vi "MC_8_27_12cbad_JW.vi"() -> ()   [LabVIEW 2011]
uses:
  <vilib>/Utility/file.llb/Read From Spreadsheet File (string).vi
  <vilib>/Utility/inputDevices.llb/keyboardAcquire.vi
  <vilib>/Utility/file.llb/Write To Spreadsheet File (DBL).vi
  <vilib>/Utility/file.llb/Write To Spreadsheet File (string).vi
  <vilib>/regexp/Match Regular Expression.xnode
panel:
  out "Vd Header Row 2":sgl
  in  "default (0 dbl)":ext format="%.2e"
  out "Vd Header Row":sgl
  out "Transport Array":string[][](array[string])
  in  "Treatment Concentration (mM):":dbl=nan
  in  "Surface Treatment:":string="NaN"
  in  "# Drops*:":dbl=inf
  in  "Solution Temp (C):":dbl=nan
  in  "Relative Humidity (%):":dbl=nan
  in  "Room Temp (F):":dbl=nan
  in  "Time (s):":dbl=nan
  in  "RPM:":dbl=nan
  in  "Wait Time (s):":dbl=nan
  in  "Sample #:":dbl=1.0
  in  "Fabricator:":string="NaN"
  in  "Ramp (s):":dbl=3.0
  out "X Axis Display Type":string
  out "Opj X Axis":string
  in  "Room Temp":dbl=294.0
  out "No Image 2":path=path "\\\\acad1\\physics/Jurchescu-group/JW-PD/Image Not Found.png"
  out "Save1 Array":string[][](array[string])
  out "Lin Vd":dbl
  out "Lin-Vg Array-Used":dbl[](array[numeric])
  out "Lin Id-Used":dbl[](array[numeric])
  out "Rec: Comments":string
  out "Folder Index":dbl caption="Length"
  out "Current \nRecord":string[](array[string])
  out "Transformer \nHeaders":string[](array[string])
  out "Current Device ID":string
  out "Column":string
  out "Row":string
  out "Rec: Concentration":dbl
  out "Rec: Solvent":string
  out "Rec: Method":string
  in  "?":T1(tab)
  in  "Transport File":path
  out "Transport Folder":path
  out "Rec: Material":string
  out "Accel (RPM/s):":dbl
  in  "Transfer File":path
  out "Transfer Folder":path
  in  "Image Folder":path
  out "Image File":path=path "D:/UserData/Desktop/Jeremy/WFU/Research/Programs/VI mods/Image Not Found.png"
  in  "Manual Comments":bool
  in  "Comments:":string
  out "Calc: On/Off":dbl caption="On/Off-Sat" format="%#.2e"
  out "Calc: Off I-Sat":dbl caption="Off I-Sat" format="%#.2e"
  in  "Manuel-Dielectric":bool
  in  "Manuel-Length":bool
  out "Calc: VT-Lin":dbl
  out "New: VT-Lin":dbl
  out "Rec: VT-Lin":dbl caption="VT-Lin" format="%#_3g"
  out "Calc: Trap Density-STS":dbl format="%#.2e"
  out "New: Trap Density-STS":dbl format="%#.2e"
  out "Rec: Trap Density-STS":dbl caption="N-Sat (STS)" format="%#.2e"
  out "Calc: Trap Density-VT":dbl format="%#.2e"
  out "New: Trap Density-VT":dbl format="%#.2e"
  out "Rec: Trap Density-VT":dbl caption="N-Sat (VT)" format="%#.2e"
  out "Calc: Mobility-Lin":dbl format="%#.2e"
  out "New: Mobility-Lin":dbl format="%#_4e"
  out "Rec: Mobility-Lin":dbl caption="Mobility-Lin" format="%#_3e"
  out "Calc: Mobility-Sat":dbl format="%#.2e"
  out "Rec: Length":dbl caption="Length" format="%#_3g"
  out "Rec: Width":dbl caption="Width" format="%#_4g"
  out "Rec: Dielectric (d)":dbl caption="Dielectric (d)" format="%#_3g"
  in  "Cancel Button":bool
  in  "Up Button":bool
  in  "Down Button":bool
  out "Data Name:":string
  in  "Save Changes?":bool
  in  "New: Dielectric":dbl
  in  "New: Length":dbl
  in  "New: Width":dbl
  out "New: Mobility-Sat":dbl format="%#.2e"
  in  "Blank Button":bool
  in  "Zoom":i16(slide)=-3 scale=-5.0..5.0
  out "Image Out 2":T2(plugin-control)
  out "Image Out":T2(plugin-control)
  in  "Magnification":u16(ring) items=["5x", "10x", "20x", "50x", "80x"]
  out "Total Width":dbl
  out "Distances":dbl[](array[numeric])
  in  "Undo Button":bool
  in  "Remove Button":bool
  out "Rec: Mobility-Sat":dbl caption="Mobility-Sat" format="%#.2e"
  in  "Export":bool
  out "Calc: VT-Sat":dbl format="%#.2g"
  out "New: VT-Sat":dbl format="%#.2g"
  in  "Manual-Width":bool caption="Manual"
  out "Calc: STS":dbl format="%#.2g"
  out "New: STS":dbl format="%#.2g"
  out "Rec: VT-Sat":dbl caption="VT-Sat" format="%#.2g"
  out "Rec: STS":dbl caption="STS-Sat" format="%#.2g"
  out "Rec: On/Off":dbl caption="On/Off-Sat" format="%#.2e"
  in  "Save Changes? 2":bool
  in  "Save Changes? 3":bool
  out "Rec: Temp":dbl caption="Sample Temp" format="%.1f"
  in  "New: Temp":dbl format="%.1f"
  out "Rec: Off I-Sat":dbl caption="Off I-Sat" format="%#.2e"
  in  "Independant Variable":string(combo)="Length (um):"
  in  "Transfer Plots":T3(tab)=enum."Saturation"
  in  "Lin-Trans Slider":dbl(slide) step=1.0 scale=-22.0..89.0 scale format="%#_1p"
  out "Sqrt-Lin":cluster{dbl[], dbl[]}[](graph)
  in  "Next Sqrt Lin":bool
  in  "Previous Sqrt Lin":bool
  in  "Sat-Trans Slider":dbl(slide) step=1.0 scale=-22.0..89.0 scale format="%#_1p"
  out "Sqrt-Sat":cluster{dbl[], dbl[]}[](graph)
  in  "Previous Sqrt Sat":bool
  in  "Next Sqrt Sat":bool
  out "Raw- Lin":cluster{dbl[], dbl[]}[](graph)
  out "Raw- Sat":cluster{dbl[], dbl[]}[](graph)
  in  "Log Plots":enum32{"Linear", "Saturation", "Transport"}(tab)=enum."Saturation"
  in  "Lin-Log Slider":dbl(slide) step=1.0 scale=-1.0..82.0 scale format="%#_1p"
  in  "Previous Log Lin":bool
  in  "Next Log Lin":bool
  out "Log-Lin":cluster{dbl[], dbl[]}[](graph)
  in  "Sat-Log Slider":dbl(slide) step=1.0 scale=-1.0..82.0 scale format="%#_1p"
  out "Log-Sat":cluster{dbl[], dbl[]}[](graph)
  in  "Previous Log Sat":bool
  in  "Next Log Sat":bool
  out "Transport":cluster{dbl[], dbl[]}[](graph)
  in  "Manual-Temp":bool caption="Manual"
  out "Date Created":string caption="Fabricated"
  out "Date Recorded":string="Date Recorded" caption="Measured"
  out "Image Name":string
  out "Index":string
  in  "Num Pts":dbl=5.0
  in  "NumPoints Log":dbl=5.0 caption="Num Pts"
  in  "Origin Project File":path=path "\\\\acad1\\physics/Jurchescu-group/JW-PD/Group Library/Origin Project Files/DeviceData_8_10_12a_JW.opj"
  in  "No Image File":path=path "\\\\acad1\\physics/Jurchescu-group/JW-PD/Mega Awesome/Image Not Found.png"
  out "String":string
  out "Index 2":dbl
  out "Sat Id-Log-Used":dbl[](array[numeric])
  out "Vg Array-Log-Used":dbl[](array[numeric])
  out "ROI Descriptor out":T4 {"Contours"."Type" items=["No Selection", "Point", "Line", "Rectangle", "Oval", "Polygon", "Freehand Region", "Annulus", "Unused2", "Unused3", "Broken Line", "Freehand Line", "Rotated Rectangle"]}
  out "ROI Descriptor":T4 {"Contours"."Type" items=["No Selection", "Point", "Line", "Rectangle", "Oval", "Polygon", "Freehand Region", "Annulus", "Unused2", "Unused3", "Broken Line", "Freehand Line", "Rotated Rectangle"]}
  out "Numeric 3":dbl
  out "Array 6":dbl[][](array[numeric])
  out "Cluster":T5
  out "Array 5":dbl[](array[numeric])
  out "Array 4":dbl[](array[numeric])
  out "Array 3":dbl[](array[numeric])
  out "Numeric 2":dbl
  out "Numeric":dbl
  out "Sat Id-Used":dbl[](array[numeric])
  out "Sat Vg Array-Used":dbl[](array[numeric])
  out "MobVi Index":dbl
  in  "Row Start":dbl=20.0
  # "Sample Properties"
  # "*     Inf = Full coverage\n   NaN = Unknown or Not Applicable"
  # "Data Locations"
  # "Transport Location"
  # "Transfer Location"
  # "Image Location"
  # "Recorded"
  # "Calculated"
  # "Re-Calculated"
  # "Manual"
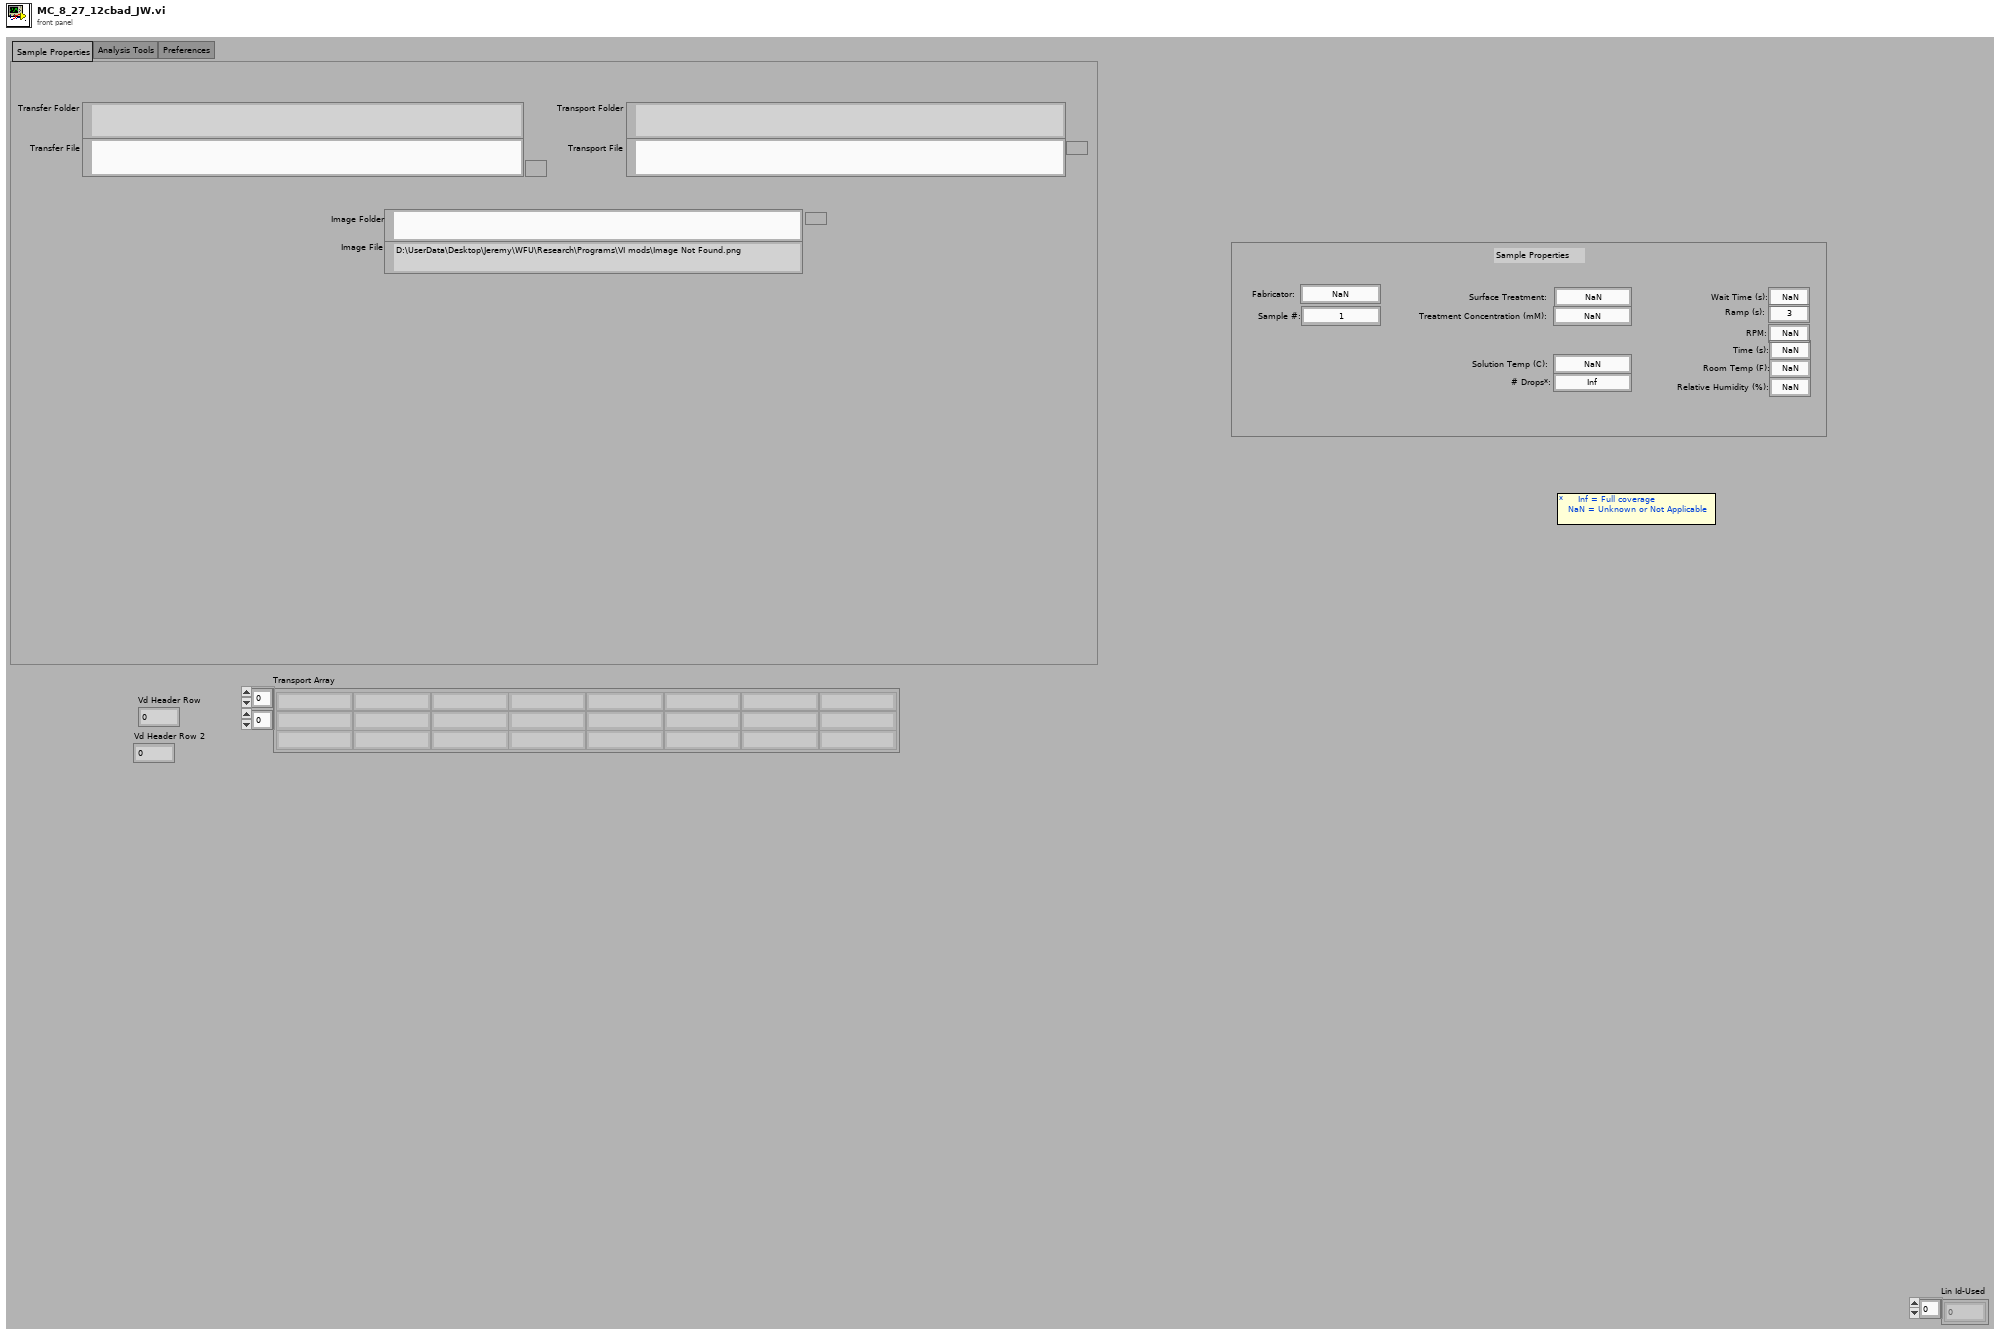
[diagram p1: front panel]
types:
  T1 = enum32{"Sample Properties", "Analysis Tools", "Preferences", "Current Database"}
  T2 = typedef "IMAQ Image.ctl" = refnum<image>
  T3 = enum32{"Linear", "Saturation", "Raw-Linear", "Raw-Saturation"}
  T4 = typedef "ROI Descriptor" = cluster{"Global Rectangle":i32[], "Contours":cluster{"ID":enum32{"External", "Internal"}, "Type":u32, "Coordinates":i32[]}[]}
  T5 = cluster{"Numeric":dbl, "Numeric 2":dbl, "Numeric 3":dbl, "Numeric 4":dbl}
  T6 = cluster{"Mobility-Sat":dbl, "Moblitity-Lin":dbl, "On/Off":dbl, "Off Current":dbl, "Vt-Sat":dbl, "STS":dbl, "Trap Density-VT":dbl, "Trap Density-STS":dbl}
  T7 = cluster{"Date Recorded":string, "Index":string, "Length":dbl, "Width":dbl, "Sample Temp":dbl}
  T8 = cluster{"Date Created":string, "Material":string, "Solvent":string, "Concentration":dbl, "Method":string, "Dielectric (nm)":dbl, "Treatment":string, "Comments":string}
  T9 = cluster{"Raw Sat":cluster{dbl[], dbl[]}[], "Sqrt Sat":cluster{dbl[], dbl[]}[], "Log Sat":cluster{dbl[], dbl[]}[], "Raw Lin":cluster{dbl[], dbl[]}[], "Sqrt Lin":cluster{dbl[], dbl[]}[], "Log Lin":cluster{dbl[], dbl[]}[]}
  T10 = cluster{"Mobility-Sat":dbl, "Vt-Sat":dbl, "Mobility-Lin":dbl, "Vt-Lin":dbl, "Off I-Sat":dbl, "On/Off I-Sat":dbl}
  T11 = cluster{"[0]":cluster{dbl[], dbl[]}, "[1]":cluster{dbl[], dbl[]}, "[2]":cluster{dbl[], dbl[]}, "[3]":cluster{dbl[], dbl[]}, "[4]":cluster{dbl[], dbl[]}, "[5]":cluster{dbl[], dbl[]}, "[6]":cluster{dbl[], dbl[]}, "[7]":cluster{dbl[], dbl[]}, "[8]":cluster{dbl[], dbl[]}}
  T12 = cluster{"Global Rectangle":i32[], "Contours":cluster{"Contour Type":u32, "ROI Type":u32, "Points":i32[]}[]}
  T13 = typedef "LVBoundsTypeDef.ctl" = cluster{"Width":u32, "Height":u32}
  T14 = enum16{"0", "1", "2", "3", "4", "5", "6", "7", "8", "9", "A", "B", "C", "D", "E", "F", "G", "H", "I", "J", "K", "L", "M", "N", "O", "P", "Q", "R", "S", "T", "U", "V", "W", "X", "Y", "Z", "F1", "F2", "F3", "F4", "F5", "F6", "F7", "F8", "F9", "F10", "F11", "F12", "F13", "F14", "F15", "ADD", "BACK", "BACKSLASH", "CAPITAL", "COMMA", "DECIMAL", "DELETE", "DIVIDE", "DOWN", "END", "EQUALS", "ESCAPE", "GRAVE (`)", "HOME", "INSERT", "LBRACKET", "LCONTROL", "LEFT", "L ALT", "LSHIFT", "LWIN", "MINUS", "MULTIPLY", "NEXT", "NUMLOCK", "NUMPAD_0", "NUMPAD_1", "NUMPAD_2", "NUMPAD_3", "NUMPAD_4", "NUMPAD_5", "NUMPAD_6", "NUMPAD_7", "NUMPAD_8", "NUMPAD_9", "PAUSE", "PERIOD", "PRIOR (PG UP)", "RBRACKET", "RCONTROL", "RETURN", "RIGHT", "R ALT", "RSHIFT", "RWIN", "SCROLL", "SEMICOLON", "SLASH", "SPACE", "SUBTRACT", "TAB", "UP", "ENTER (num pad)", "' (quote)"}[]
  T15 = enum16{"0", "1", "2", "3", "4", "5", "6", "7", "8", "9", "A", "B", "C", "D", "E", "F", "G", "H", "I", "J", "K", "L", "M", "N", "O", "P", "Q", "R", "S", "T", "U", "V", "W", "X", "Y", "Z", "F1", "F2", "F3", "F4", "F5", "F6", "F7", "F8", "F9", "F10", "F11", "F12", "F13", "F14", "F15", "ADD", "BACK", "BACKSLASH", "CAPITAL", "COMMA", "DECIMAL", "DELETE", "DIVIDE", "DOWN", "END", "EQUALS", "ESCAPE", "GRAVE (`)", "HOME", "INSERT", "LBRACKET", "LCONTROL", "LEFT", "L ALT", "LSHIFT", "LWIN", "MINUS", "MULTIPLY", "NEXT", "NUMLOCK", "NUMPAD_0", "NUMPAD_1", "NUMPAD_2", "NUMPAD_3", "NUMPAD_4", "NUMPAD_5", "NUMPAD_6", "NUMPAD_7", "NUMPAD_8", "NUMPAD_9", "PAUSE", "PERIOD", "PRIOR (PG UP)", "RBRACKET", "RCONTROL", "RETURN", "RIGHT", "R ALT", "RSHIFT", "RWIN", "SCROLL", "SEMICOLON", "SLASH", "SPACE", "SUBTRACT", "TAB", "UP", "ENTER (num pad)", "' (quote)"}
  T16 = cluster{"Contour Type":u32, "ROI Type":u32, "Points":i32[]}[]
  T17 = cluster{i32[], cluster{"Contour Type":u32, "ROI Type":u32, "Points":i32[]}[]}
  T18 = cluster{"Independant  Variable Indicator":string, "Parameter String Indicator":string}
  T19 = cluster{string, sgl, bool, bool, bool, bool, bool, bool, i32}
  T20 = cluster{i32, cluster{string, sgl, bool, bool, bool, bool, bool, bool, i32}, i32, i32}
  T21 = cluster{"Contour Type":u32, "ROI Type":u32, "Points":i32[]}
  T22 = cluster{"Points[0]":i32, "Points[1]":i32, "Points[2]":i32, "Points[3]":i32, "Points[4]":i32, "Points[5]":i32, "Points[6]":i32, "Points[7]":i32, "Points[8]":i32}
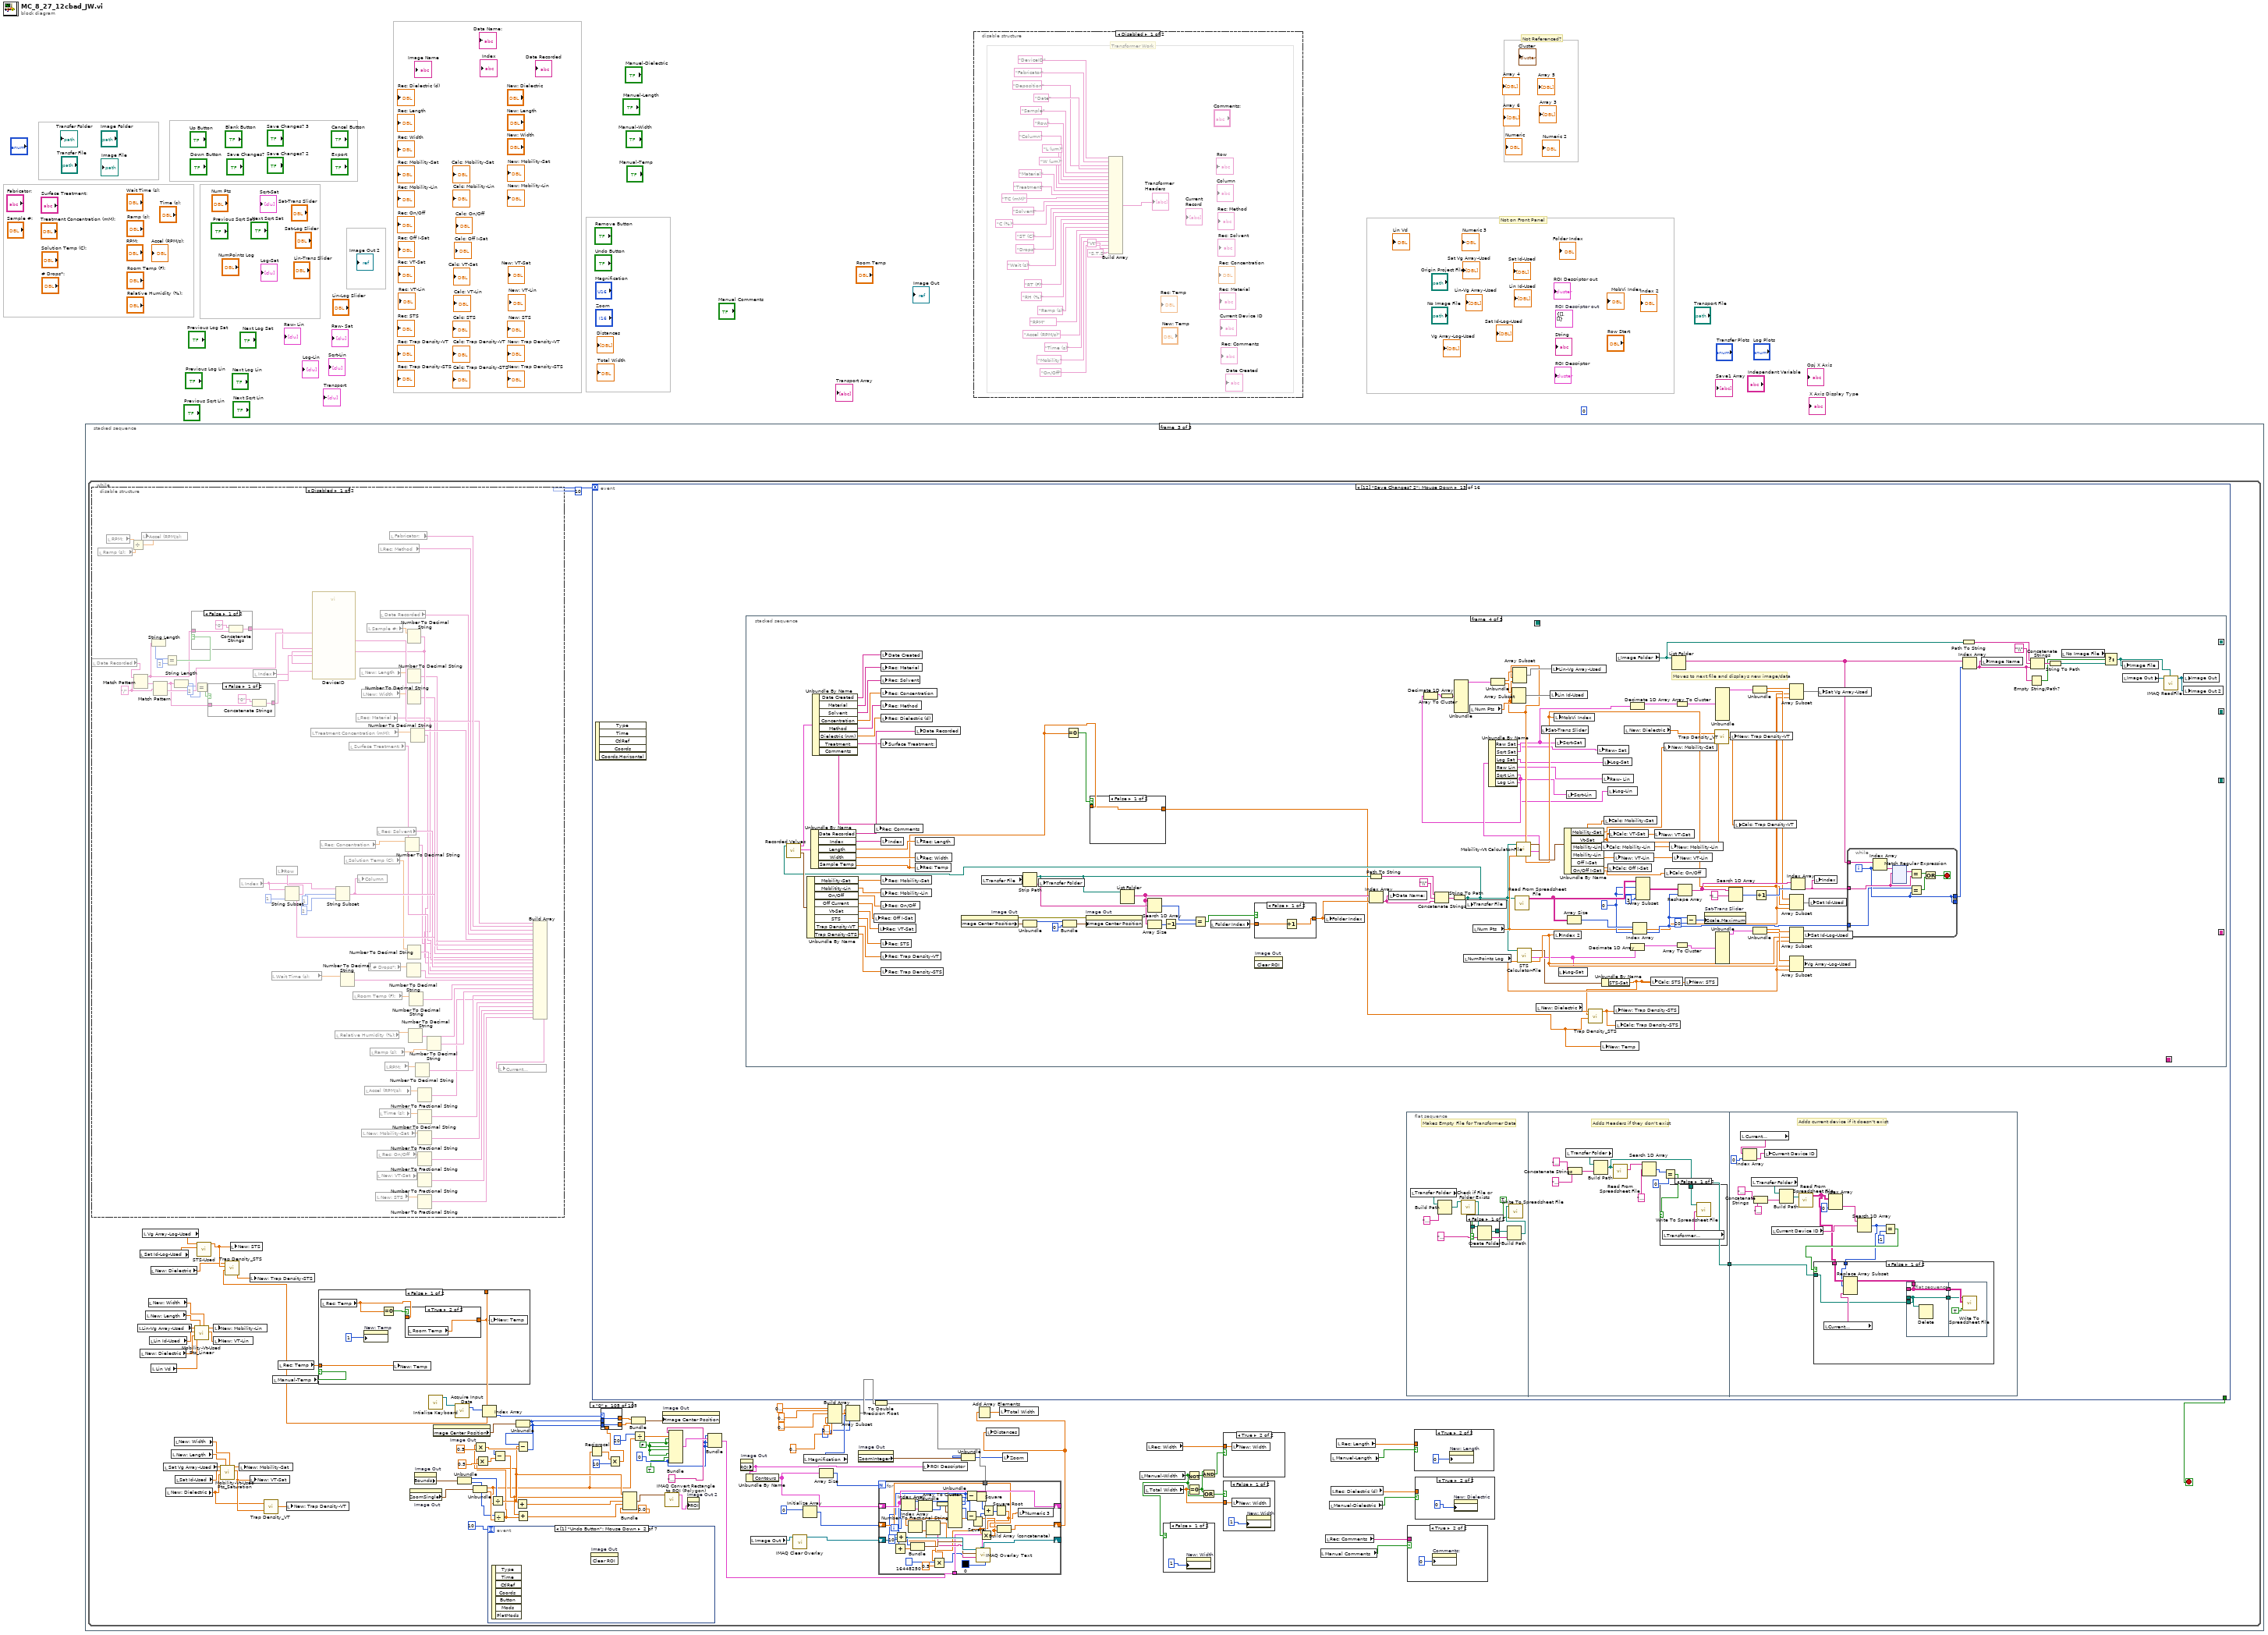
[diagram p0: block diagram]
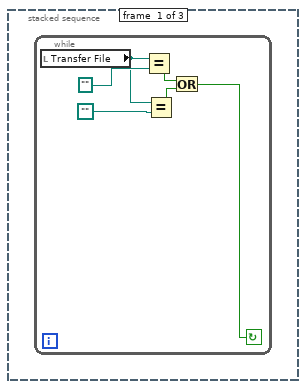
[diagram p3: hidden frame]
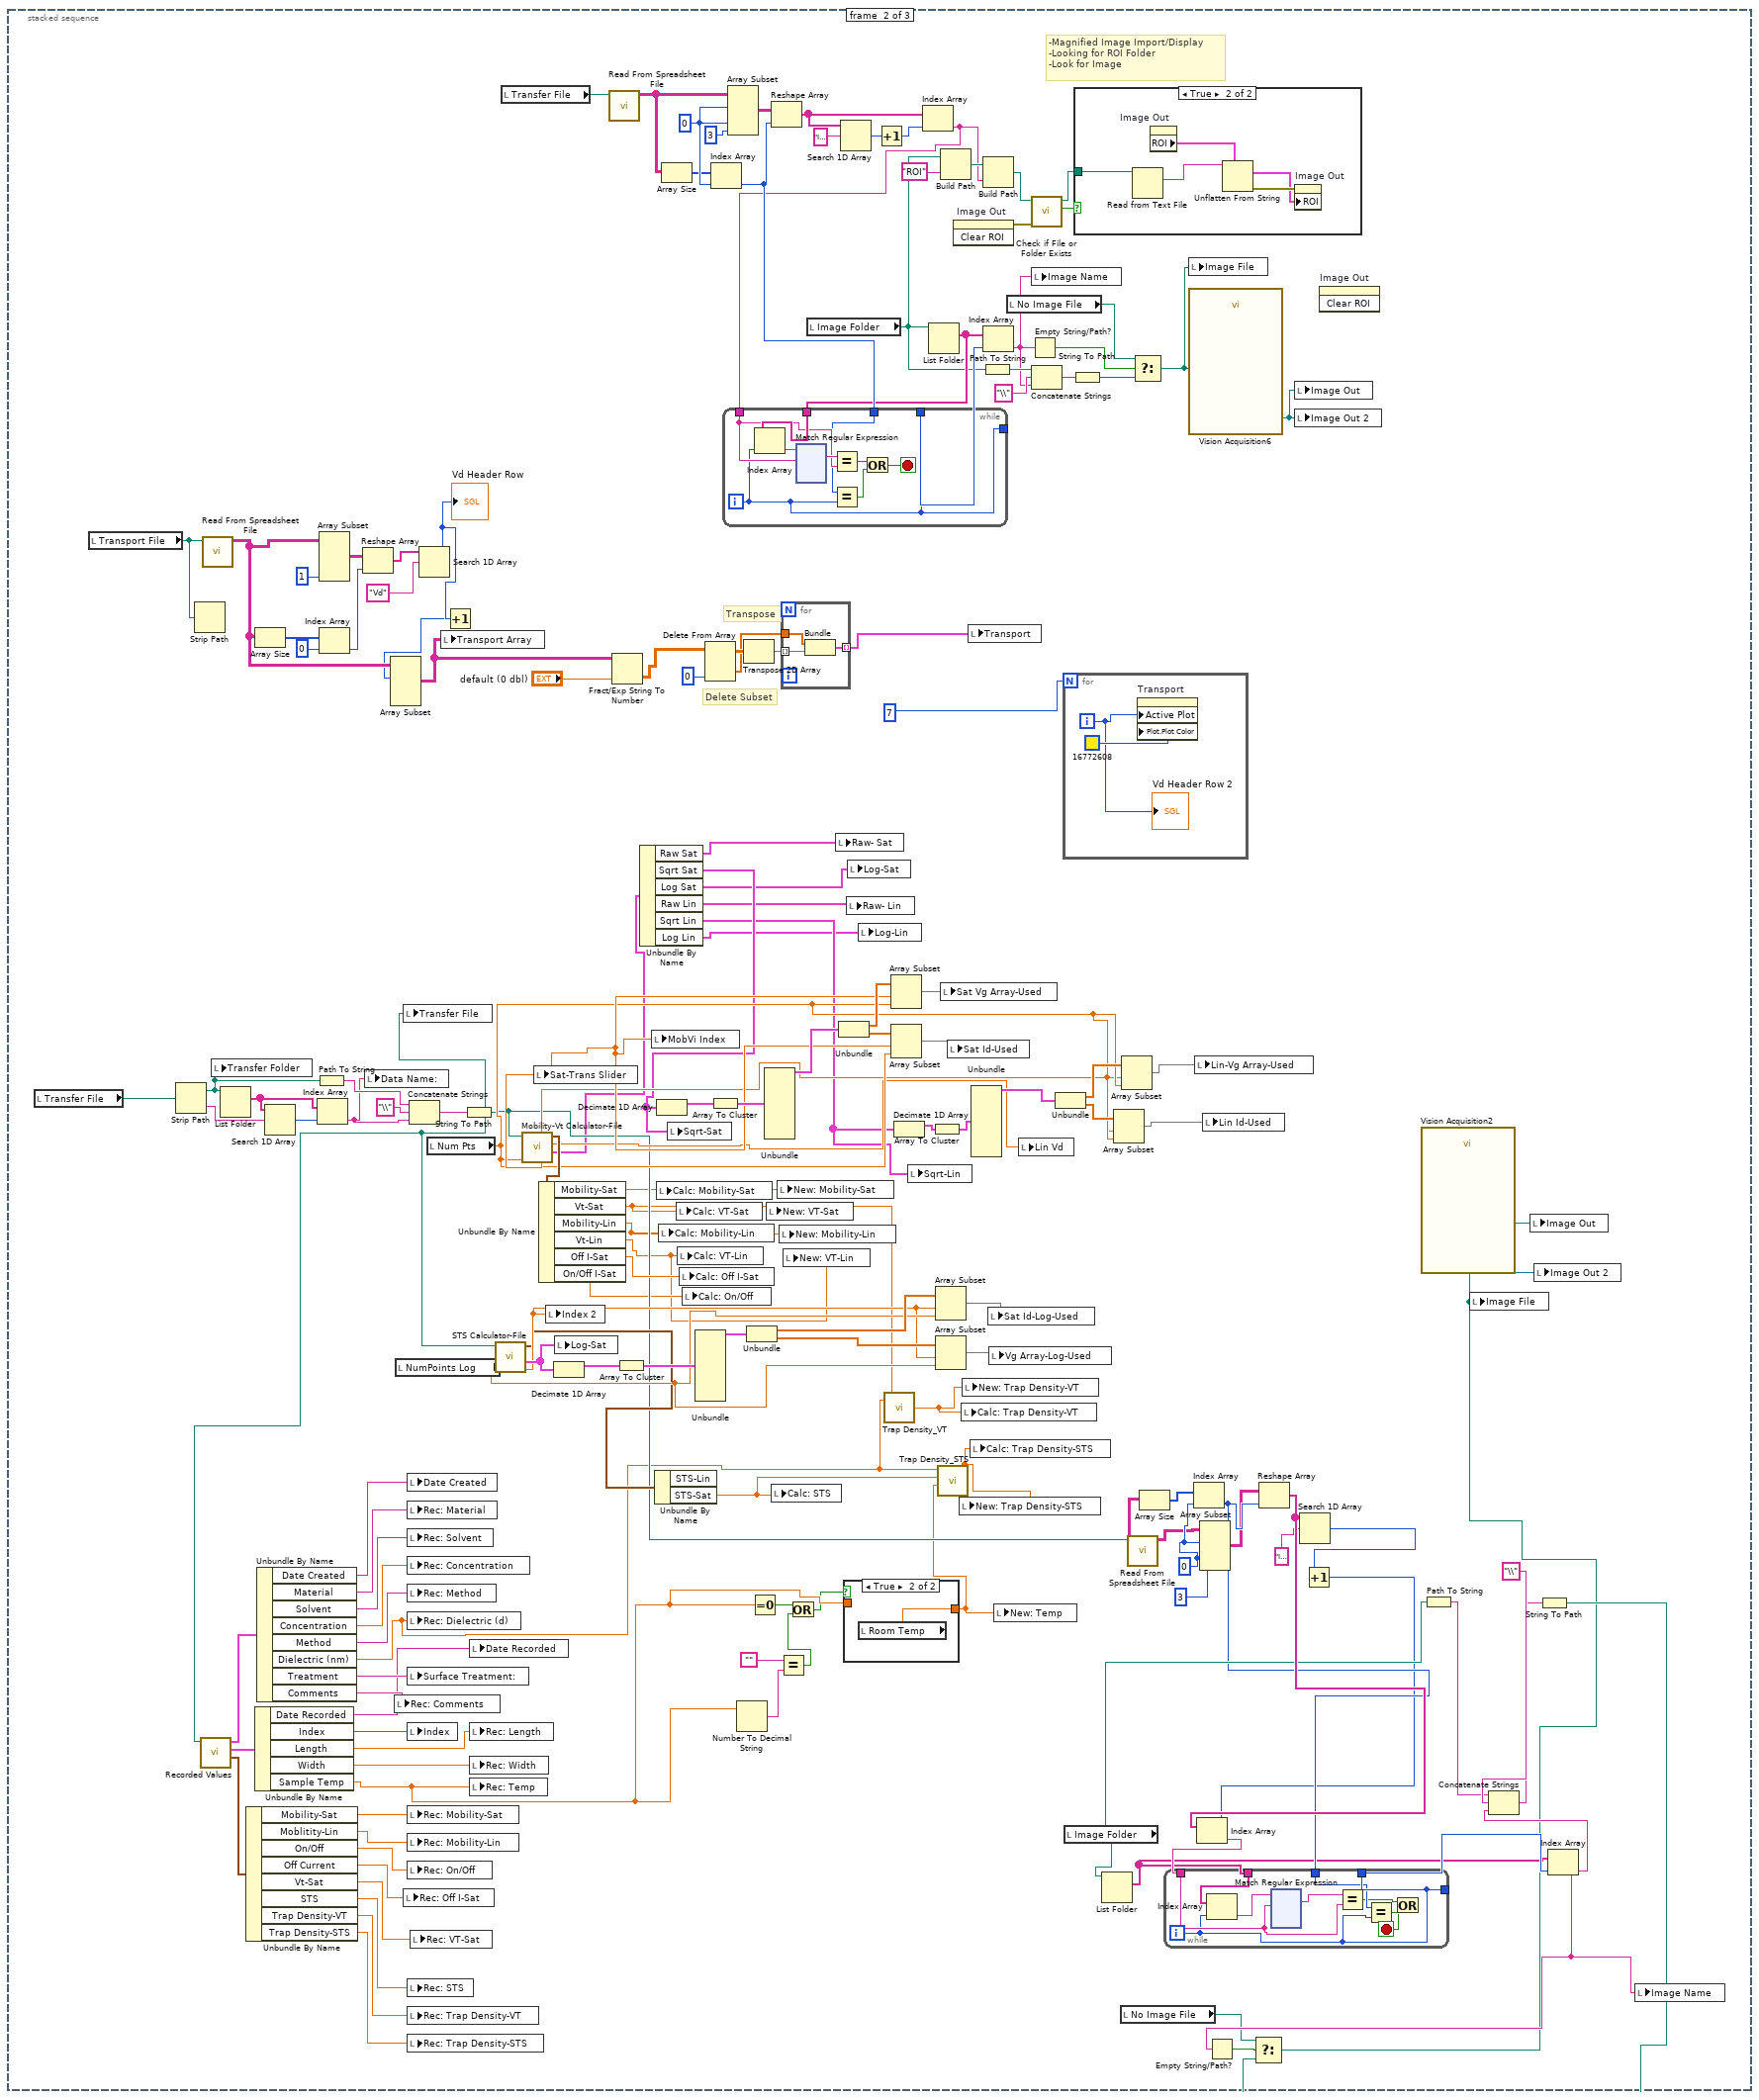
[diagram p4: hidden frame]
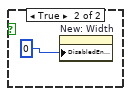
[diagram p10: hidden frame]
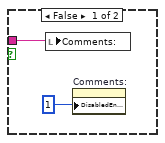
[diagram p11: hidden frame]
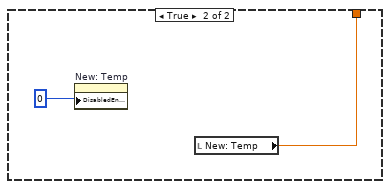
[diagram p13: hidden frame]
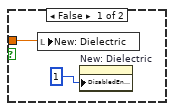
[diagram p14: hidden frame]
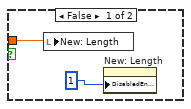
[diagram p15: hidden frame]
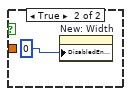
[diagram p17: hidden frame]
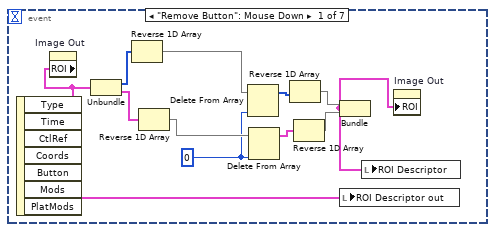
[diagram p18: hidden frame]
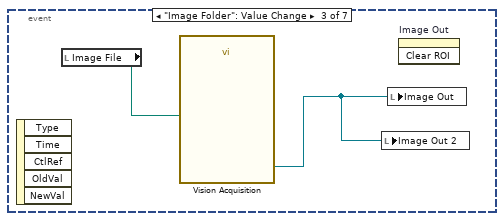
[diagram p19: hidden frame]
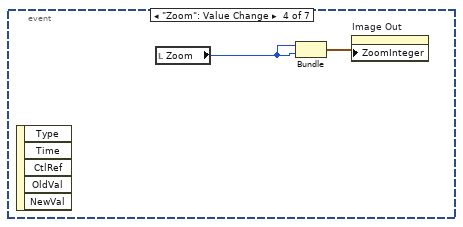
[diagram p20: hidden frame]
diagram:
  (unwired) 0
  (unwired) T4 {"Global Rectangle"=[], "Contours"=[]}  # ROI Descriptor out
  # "Not Referenced?"
  # "Not on Front Panel"
  n1 = stacked-sequence {
    frame #0 {
      n2 = while {
        stop <- w1 continue-if-true
        n3 = local read "Transfer File"() -> (w3:path)
        n4 = Equal?(x=w3, y=path "") -> (x = y?=w5:bool)
        n5 = Equal?(x=w3, y=path "") -> (x = y?=w4:bool)
        n6 = Or(x=w5, y=w4) -> (x .or. y?=w1:bool)
      }
    }
    frame #1 {
      w130 = 0
      w154 = 0
      # "Transpose"
      # "Delete Subset"
      # "-Magnified Image Import/Display\n-Looking for ROI Folder\n-Look for Image"
      n7 = local read "Transfer File"() -> (w134:path)
      n8 = local read "Transport File"() -> (w26:path)
      n9 = Strip Path(path=w134) -> (stripped path=w135:path, name=w121:string)
      n10 = Strip Path(path=w26) -> ()  [unwired: 2 out]
      n11 = call-poly <vilib>:"Read From Spreadsheet File.vi"("file path (dialog if empty)"=w26) -> ("all rows"=w19:string[][])  [unwired: 6 in, 4 out]
      n12 = local write "Transfer Folder"(w135) -> ()
      n13 = List Folder(path=w135) -> (filenames=w125:string[])  [unwired: 3 in, 3 out]
      n14 = Array Size(array=w19) -> (size(s)=w25:i32[])
      n15 = Search 1D Array(1D array=w125, element=w121) -> (index of element=w124:i32)  [unwired: 1 in]
      n16 = Path To String(path=w135) -> (string=w120:string)
      n17 = Index Array(array=w125, index=w124) -> (element=w90:string)
      n18 = Array Subset(array=w19, length (col)=1) -> (w21:string[][])  [unwired: 3 in]
      n19 = Index Array(array=w25, index=0) -> (element=w14:i32)
      n20 = Reshape Array(w21, w14) -> (w20:string[])
      n21 = local write "Data Name:"(w90) -> ()
      n22 = local read "NumPoints Log"() -> (w66:dbl)
      n23 = Concatenate Strings(w120, "\\", w90) -> (w122:string)
      n24 = Search 1D Array(1D array=w20, element="Vd") -> (index of element=w18:i32)  [unwired: 1 in]
      "Vd Header Row" <- w18
      n25 = local read "Num Pts"() -> (w57:dbl)
      n26 = Increment(x=w18) -> (x+1=w17:i32)
      n27 = Array Subset(array=w19, index (row)=w17) -> (w15:string[][])  [unwired: 3 in]
      n28 = local write "Transport Array"(w15) -> ()
      n29 = String To Path(string=w122) -> (path=w51:path)
      n30 = call "Recorded Values.vi"("Path"=w51) -> ("Recorded Char"=w88:T6, "Recorded Prop"=w87:T7, "Fabrication Prop"=w89:T8)  [unwired: 8 in]
      n31 = Unbundle By Name(w88) -> ("Mobility-Sat"=w76:dbl, "Moblitity-Lin"=w75:dbl, "On/Off"=w74:dbl, "Off Current"=w73:dbl, "Vt-Sat"=w37:dbl, "STS"=w72:dbl, "Trap Density-VT"=w71:dbl, "Trap Density-STS"=w70:dbl)
      n32 = Unbundle By Name(w87) -> ("Date Recorded"=w80:string, "Index"=w79:string, "Length"=w78:dbl, "Width"=w77:dbl, "Sample Temp"=w43:dbl)
      n33 = Unbundle By Name(w89) -> ("Date Created"=w69:string, "Material"=w86:string, "Solvent"=w85:string, "Concentration"=w84:dbl, "Method"=w83:string, "Dielectric (nm)"=w47:dbl, "Treatment"=w82:string, "Comments"=w81:string)
      n34 = local write "Rec: Comments"(w81) -> ()
      n35 = local write "Transfer File"(w51) -> ()
      n36 = local write "Rec: Off I-Sat"(w73) -> ()
      n37 = local write "Date Created"(w69) -> ()
      n38 = local write "Rec: Material"(w86) -> ()
      n39 = local write "Rec: Solvent"(w85) -> ()
      n40 = local write "Rec: Concentration"(w84) -> ()
      n41 = local write "Rec: Method"(w83) -> ()
      n42 = local write "Rec: Dielectric (d)"(w47) -> ()
      n43 = local write "Surface Treatment:"(w82) -> ()
      n44 = local write "Index"(w79) -> ()
      n45 = local write "Rec: Mobility-Sat"(w76) -> ()
      n46 = local write "Rec: Mobility-Lin"(w75) -> ()
      n47 = local write "Rec: On/Off"(w74) -> ()
      n48 = local write "Rec: STS"(w72) -> ()
      n49 = local write "Rec: Trap Density-VT"(w71) -> ()
      n50 = local write "Rec: Trap Density-STS"(w70) -> ()
      n51 = local write "Rec: VT-Sat"(w37) -> ()
      n52 = local write "Date Recorded"(w80) -> ()
      n53 = local write "Rec: Length"(w78) -> ()
      n54 = local write "Rec: Width"(w77) -> ()
      n55 = local write "Rec: Temp"(w43) -> ()
      n56 = call "STS Calculator-File.vi"("NumPts"=w66, "Path"=w51) -> ("STS Index-Sat"=w64:dbl, "XY Graph-Sat"=w65:cluster{dbl[], dbl[]}[], "Ouput"=w63:cluster{"STS-Sat":dbl, "STS-Lin":dbl})  [unwired: 5 in, 2 out]
      n57 = local read "Transfer File"() -> (w149:path)
      n58 = call "Mobility-Vt Calculator-File.vi"("NumPts"=w57, "Path"=w51) -> ("Graph Cluster"=w27:T9, "Lin Vd"=w53:dbl, "Output"=w68:T10, "Index-Sat"=w67:dbl, "Index-Lin"=w56:dbl)  [unwired: 5 in]
      n59 = local write "Sat-Trans Slider"(w67) -> ()
      n60 = Unbundle By Name(w68) -> ("Mobility-Sat"=w46:dbl, "Vt-Sat"=w45:dbl, "Mobility-Lin"=w36:dbl, "Vt-Lin"=w34:dbl, "Off I-Sat"=w52:dbl, "On/Off I-Sat"=w35:dbl)
      n61 = local write "Index 2"(w64) -> ()
      n62 = Decimate 1D Array(w65) -> (w112:cluster{dbl[], dbl[]}[])  [unwired: 1 out]
      n63 = local write "Log-Sat"(w65) -> ()
      n64 = call-poly <vilib>:"Read From Spreadsheet File.vi"("file path (dialog if empty)"=w149) -> ("all rows"=w152:string[][])  [unwired: 6 in, 4 out]
      n65 = Fract/Exp String To Number(string=w15, default (0 dbl)="default (0 dbl)") -> (number=w9:ext[][])  [unwired: 2 in, 1 out]
      n66 = Array To Cluster(array=w112) -> (cluster=w114:T11)
      n67 = Unbundle By Name(w27) -> ("Raw Sat"=w31:cluster{dbl[], dbl[]}[], "Sqrt Sat"=w33:cluster{dbl[], dbl[]}[], "Log Sat"=w28:cluster{dbl[], dbl[]}[], "Raw Lin"=w30:cluster{dbl[], dbl[]}[], "Sqrt Lin"=w32:cluster{dbl[], dbl[]}[], "Log Lin"=w29:cluster{dbl[], dbl[]}[])
      n68 = local write "MobVi Index"(w67) -> ()
      n69 = Unbundle By Name(w63) -> ("STS-Sat"=w50:dbl)  [unwired: 1 out]
      n70 = Decimate 1D Array(w33) -> (w148:cluster{dbl[], dbl[]}[])  [unwired: 1 out]
      n71 = local write "Calc: Mobility-Sat"(w46) -> ()
      n72 = local write "Calc: Mobility-Lin"(w36) -> ()
      n73 = Array Size(array=w152) -> (size(s)=w153:i32[])
      n74 = local write "Sqrt-Sat"(w33) -> ()
      n75 = local write "Calc: VT-Sat"(w45) -> ()
      n76 = local write "Calc: VT-Lin"(w34) -> ()
      n77 = local write "Calc: Off I-Sat"(w52) -> ()
      n78 = local write "Calc: On/Off"(w35) -> ()
      n79 = Unbundle(w114) -> ("[0]"=w113:cluster{dbl[], dbl[]})  [unwired: 8 out]
      n80 = Delete From Array(array=w9, index (col)=0 ("Deaktivierter Index (Spalte)")) -> (deleted portion=w11:ext[], array with subset deleted=w12:ext[][])  [unwired: 2 in]
      n81 = Array To Cluster(array=w148) -> (cluster=w146:T11)
      n82 = Index Array(array=w153, index=w154) -> (element=w160:i32)
      n83 = Array Subset(array=w152, index (row)=w154, index (col)=w154, length (col)=3) -> (w151:string[][])  [unwired: 1 in]
      n84 = Number To Decimal String(number=w43) -> (decimal integer string=w41:string)  [unwired: 1 in]
      n85 = Transpose 2D Array(2D array=w12) -> (transposed array=w13:ext[][])
      n86 = Unbundle(w113) -> (w110:dbl[], w109:dbl[])
      n87 = Equal To 0?(x=w43) -> (x = 0?=w42:bool)
      n88 = Unbundle(w146) -> ("[0]"=w147:cluster{dbl[], dbl[]})  [unwired: 8 out]
      n89 = local write "New: VT-Sat"(w45) -> ()
      n90 = Reshape Array(w151, w160) -> (w165:string[])
      n91 = local write "Calc: STS"(w50) -> ()
      n92 = local write "New: Mobility-Sat"(w46) -> ()
      n93 = Equal?(x="", y=w41) -> (x = y?=w39:bool)
      n94 = local write "New: Mobility-Lin"(w36) -> ()
      n95 = for {
        tunnel: w11 -> [w169]
        tunnel: w13 -> [w170] mode=indexing
        tunnel: [w168] -> w8 mode=indexing
        n96 = Bundle(w169, w170) -> (w168:cluster{ext[], ext[]})  [unwired: 1 in]
      }
      n97 = local write "New: VT-Lin"(w34) -> ()
      n98 = Or(x=w42, y=w39) -> (x .or. y?=w38:bool)
      n99 = local read "Image Folder"() -> (w91:path)
      n100 = local write "Raw- Sat"(w31) -> ()
      n101 = Unbundle(w147) -> (w111:dbl[], w115:dbl[])
      n102 = Search 1D Array(1D array=w165, element="Index:") -> (index of element=w157:i32)  [unwired: 1 in]
      n103 = case shown="True" w38 {
        tunnel: [w171 w172] -> w49
        tunnel: w43 -> [w171 _]
        frame False {
        }
        frame True {
          n104 = local read "Room Temp"() -> (w172:dbl)
        }
      }
      n105 = local write "Raw- Lin"(w30) -> ()
      n106 = local write "Log-Sat"(w28) -> ()
      n107 = local write "Log-Lin"(w29) -> ()
      n108 = Increment(x=w157) -> (x+1=w156:i32)
      n109 = call "Trap Density_VT.vi"("VT"=w45, "Dielectric"=w47) -> ("Trap Density-VT"=w44:dbl)
      n110 = Array Subset(array=w111, index=w67, length=w57) -> (w118:dbl[])
      n111 = Array Subset(array=w115, index=w67, length=w57) -> (w119:dbl[])
      n112 = Decimate 1D Array(w32) -> (w62:cluster{dbl[], dbl[]}[])  [unwired: 1 out]
      n113 = local write "Sqrt-Lin"(w32) -> ()
      n114 = Index Array(array=w165, index=w156) -> (element=w92:string)
      n115 = List Folder(path=w91) -> (filenames=w158:string[])  [unwired: 3 in, 3 out]
      n116 = while {
        tunnel: w158 -> [w305]
        tunnel: w92 -> [w303]
        tunnel: [w302] -> _
        tunnel: [w302] -> w159
        tunnel: w160 -> [w301]
        i -> [w302]
        stop <- w298 stop-if-true
        n117 = Index Array(array=w305, index=w302) -> (element=w306:string)
        n118 = xnode "Match Regular Expression"("input string"=w306, "regular expression"=w303) -> ("whole match"=w304:string)  [unwired: 4 in, 4 out]
        n119 = Equal?(x=w304, y=w303) -> (x = y?=w300:bool)
        n120 = Equal?(x=w301, y=w302) -> (x = y?=w299:bool)
        n121 = Or(x=w300, y=w299) -> (x .or. y?=w298:bool)
      }
      n122 = Array To Cluster(array=w62) -> (cluster=w61:T11)
      n123 = Array Subset(array=w110, index=w64, length=w66) -> (w117:dbl[])
      n124 = Array Subset(array=w109, index=w64, length=w66) -> (w116:dbl[])
      n125 = call "Trap Density_STS.vi"("Temp (T) [K]"=w49, "S.T.S. (S)"=w50, "Dielectric"=w47) -> ("Trap Density (N)"=w48:dbl)  [unwired: 8 in]
      n126 = Build Path(base path=w91, name or relative path="ROI") -> (appended path=w94:path)
      n127 = local write "Sat Vg Array-Used"(w118) -> ()
      n128 = local write "Sat Id-Used"(w119) -> ()
      n129 = invoke on="Image Out" class="ImageControl" method="Clear ROI"() -> (error out=w98:errorcluster)  [unwired: 3 in, 2 out]
      n130 = local write "New: Trap Density-STS"(w48) -> ()
      n131 = local write "Calc: Trap Density-VT"(w44) -> ()
      n132 = local write "New: Trap Density-VT"(w44) -> ()
      n133 = local write "Transport"(w8) -> ()
      n134 = local write "Calc: Trap Density-STS"(w48) -> ()
      n135 = Unbundle(w61) -> ("[0]"=w60:cluster{dbl[], dbl[]})  [unwired: 8 out]
      n136 = Path To String(path=w91) -> (string=w162:string)
      n137 = Build Path(base path=w94, name or relative path=w92) -> (appended path=w93:path)
      n138 = Index Array(array=w158, index=w159) -> (element=w108:string)
      n139 = local write "Sat Id-Log-Used"(w117) -> ()
      n140 = local write "Vg Array-Log-Used"(w116) -> ()
      n141 = local write "New: Temp"(w49) -> ()
      n142 = local read "No Image File"() -> (w99:path)
      n143 = local write "Lin Vd"(w53) -> ()
      n144 = Empty String/Path?(string/path=w108) -> (empty?=w107:bool)
      n145 = call <vilib>:"Check if File or Folder Exists.vi"("error in (no error)"=w98, "path"=w93) -> ("file or folder exists?"=w96:bool, "dup path"=w97:path)  [unwired: 7 in, 1 out]
      n146 = local write "Image Name"(w108) -> ()
      n147 = Concatenate Strings(w162, "\\", w108) -> (w163:string)
      n148 = Unbundle(w60) -> (w59:dbl[], w58:dbl[])
      n149 = for {
        N: 7 -> [_]
        i -> [w166]
        n150 = property on="Transport" class="XYGraph (strict)"("Active Plot"=w166, "Plot.Plot Color"=u32 16772608) -> ()  [unwired: 2 in, 2 out]
        "Vd Header Row 2" <- w166
      }
      n151 = local read "Image Folder"() -> (w141:path)
      n152 = String To Path(string=w163) -> (path=w106:path)
      n153 = case shown="True" w96 {
        tunnel: w97 -> [_ w173]
        frame False {
        }
        frame True {
          n154 = Read from Text File(file (use dialog)=w173) -> (text=w177:string)  [unwired: 3 in, 3 out]
          n155 = property on="Image Out" class="ImageControl"() -> ("ROI"=w174:T12)  [unwired: 2 in, 2 out]
          n156 = Unflatten From String(type=w174, binary string=w177) -> (value=w175:T12, error out=w176:errorcluster)  [unwired: 3 in, 1 out]
          n157 = property on="Image Out" class="ImageControl"(error in=w176, "ROI"=w175) -> ()  [unwired: 1 in, 2 out]
        }
      }
      n158 = List Folder(path=w141) -> (filenames=w137:string[])  [unwired: 3 in, 3 out]
      n159 = Array Subset(array=w58, index=w56, length=w57) -> (w54:dbl[])
      n160 = local read "No Image File"() -> (w100:path)
      n161 = Array Subset(array=w59, index=w56, length=w57) -> (w55:dbl[])
      n162 = call-poly <vilib>:"Read From Spreadsheet File.vi"("file path (dialog if empty)"=w51) -> ("all rows"=w128:string[][])  [unwired: 6 in, 4 out]
      n163 = Select(t=w99, s=w107, f=w106) -> (s? t:f=w105:path)
      n164 = Array Size(array=w128) -> (size(s)=w129:i32[])
      n165 = local write "Image File"(w105) -> ()
      n166 = call "Vision Acquisition6"("Image Path"=w105) -> ("Image Out"=w161:T2)  [unwired: 25 in, 1 out]
      n167 = Index Array(array=w129, index=w130) -> (element=w140:i32)
      n168 = local write "Lin-Vg Array-Used"(w55) -> ()
      n169 = Array Subset(array=w128, index (row)=w130, index (col)=w130, length (col)=3) -> (w127:string[][])  [unwired: 1 in]
      n170 = local write "Lin Id-Used"(w54) -> ()
      n171 = Reshape Array(w127, w140) -> (w145:string[])
      n172 = local write "Image Out"(w161) -> ()
      n173 = local write "Image Out 2"(w161) -> ()
      n174 = Search 1D Array(1D array=w145, element="Index:") -> (index of element=w133:i32)  [unwired: 1 in]
      n175 = Increment(x=w133) -> (x+1=w132:i32)
      n176 = Index Array(array=w145, index=w132) -> (element=w138:string)
      n177 = while {
        tunnel: w137 -> [w185]
        tunnel: w138 -> [w183]
        tunnel: [w182] -> _
        tunnel: [w182] -> w139
        tunnel: w140 -> [w181]
        i -> [w182]
        stop <- w178 stop-if-true
        n178 = Index Array(array=w185, index=w182) -> (element=w186:string)
        n179 = xnode "Match Regular Expression"("input string"=w186, "regular expression"=w183) -> ("whole match"=w184:string)  [unwired: 4 in, 4 out]
        n180 = Equal?(x=w184, y=w183) -> (x = y?=w180:bool)
        n181 = Equal?(x=w181, y=w182) -> (x = y?=w179:bool)
        n182 = Or(x=w180, y=w179) -> (x .or. y?=w178:bool)
      }
      n183 = invoke on="Image Out" class="ImageControl" method="Clear ROI"() -> ()  [unwired: 3 in, 3 out]
      n184 = Path To String(path=w141) -> (string=w142:string)
      n185 = Index Array(array=w137, index=w139) -> (element=w103:string)
      n186 = Empty String/Path?(string/path=w103) -> (empty?=w104:bool)
      n187 = Concatenate Strings(w142, "\\", w103) -> (w143:string)
      n188 = String To Path(string=w143) -> (path=w102:path)
      n189 = Select(t=w100, s=w104, f=w102) -> (s? t:f=w101:path)
      n190 = call "Vision Acquisition2"("Image Path"=w101) -> ("Image Out"=w136:T2)  [unwired: 25 in, 1 out]
      n191 = local write "Image File"(w101) -> ()
      n192 = local write "Image Out"(w136) -> ()
      n193 = local write "Image Out 2"(w136) -> ()
      n194 = local write "Image Name"(w103) -> ()
    }
    frame #2 {
      n195 = while {
        stop <- w517 stop-if-true
        w467 = FALSE
        w465 = 0
        n196 = disable-structure shown="Disabled" {
          frame Disabled {
            w551 = "/"
            n197 = local read "Date Recorded"() -> (w554:string)
            n198 = local read "Ramp (s):"() -> (w521:dbl)
            n199 = local read "RPM:"() -> (w522:dbl)
            n200 = Divide(x=w522, y=w521) -> (x/y=w520:dbl)
            n201 = Match Pattern(string=w554, regular expression=w551) -> (before substring=w545:string, after substring=w552:string)  [unwired: 1 in, 2 out]
            n202 = local write "Accel (RPM/s):"(w520) -> ()
            n203 = String Length(string=w545) -> (length=w548:i32)
            n204 = Match Pattern(string=w552, regular expression=w551) -> (before substring=w539:string, after substring=w550:string)  [unwired: 1 in, 2 out]
            n205 = Equal?(x=w548, y=2) -> (x = y?=w546:bool)
            n206 = String Length(string=w539) -> (length=w541:i32)
            n207 = case shown="False" w546 {
              tunnel: w545 -> [w591 w593]
              tunnel: [w590 w593] -> w544
              frame False {
                n208 = Concatenate Strings("0", w591) -> (w590:string)
              }
              frame True {
              }
            }
            n209 = Equal?(x=w541, y=2) -> (x = y?=w543:bool)
            n210 = case shown="False" w543 {
              tunnel: w539 -> [w587 w589]
              tunnel: [w586 w589] -> w540
              frame False {
                n211 = Concatenate Strings("0", w587) -> (w586:string)
              }
              frame True {
              }
            }
            n212 = local read "Index"() -> (w524:string)
            n213 = local read "Index"() -> (w538:string)
            n214 = local read "Wait Time (s):"() -> (w584:dbl)
            n215 = String Subset(string=w524, length (rest)=1) -> (substring=w579:string)  [unwired: 1 in]
            n216 = local write "Row"(w579) -> ()
            n217 = local read "Treatment Concentration (mM):"() -> (w532:dbl)
            n218 = local read "Rec: Concentration"() -> (w519:dbl)
            n219 = local read "Relative Humidity (%):"() -> (w529:dbl)
            n220 = String Subset(string=w524, offset (0)=1, length (rest)=2) -> (substring=w580:string)
            n221 = Number To Decimal String(number=w584) -> (decimal integer string=w585:string)  [unwired: 1 in]
            n222 = local read "Solution Temp (C):"() -> (w573:dbl)
            n223 = local read "Surface Treatment:"() -> (w531:string)
            n224 = local read "Room Temp (F):"() -> (w577:dbl)
            n225 = local read "Rec: Material"() -> (w527:string)
            n226 = local write "Column"(w580) -> ()
            n227 = local read "New: Length"() -> (w537:dbl)
            n228 = local read "New: Width"() -> (w536:dbl)
            n229 = local read "New: Mobility-Sat"() -> (w566:dbl)
            n230 = local read "Accel (RPM/s):"() -> (w564:dbl)
            n231 = local read "Sample #:"() -> (w556:dbl)
            n232 = local read "# Drops*:"() -> (w574:dbl)
            n233 = local read "Ramp (s):"() -> (w582:dbl)
            n234 = local read "New: STS"() -> (w558:dbl)
            n235 = local read "Rec: Solvent"() -> (w533:string)
            n236 = local read "New: VT-Sat"() -> (w560:dbl)
            n237 = local read "Rec: On/Off"() -> (w562:dbl)
            n238 = local read "Rec: Method"() -> (w557:string)
            n239 = local read "Time (s):"() -> (w569:dbl)
            n240 = local read "Date Recorded"() -> (w553:string)
            n241 = local read "RPM:"() -> (w570:dbl)
            n242 = local read "Fabricator:"() -> (w578:string)
            n243 = Number To Decimal String(number=w519) -> (decimal integer string=w518:string)  [unwired: 1 in]
            n244 = Number To Decimal String(number=w574) -> (decimal integer string=w575:string)  [unwired: 1 in]
            n245 = Number To Decimal String(number=w556) -> (decimal integer string=w549:string)  [unwired: 1 in]
            n246 = call "DeviceID"("Sample"=w549, "Year"=w550, "Month"=w544, "Day"=w540, "Index"=w538) -> ("Result"=w555:string)  [unwired: 9 in, 1 out]
            n247 = Number To Decimal String(number=w537) -> (decimal integer string=w535:string)  [unwired: 1 in]
            n248 = Number To Decimal String(number=w536) -> (decimal integer string=w534:string)  [unwired: 1 in]
            n249 = Number To Decimal String(number=w573) -> (decimal integer string=w572:string)  [unwired: 1 in]
            n250 = Number To Decimal String(number=w529) -> (decimal integer string=w528:string)  [unwired: 1 in]
            n251 = Number To Decimal String(number=w577) -> (decimal integer string=w576:string)  [unwired: 1 in]
            n252 = Number To Decimal String(number=w532) -> (decimal integer string=w530:string)  [unwired: 1 in]
            n253 = Number To Decimal String(number=w570) -> (decimal integer string=w571:string)  [unwired: 1 in]
            n254 = Number To Fractional String(number=w564) -> (F-format string=w565:string)  [unwired: 3 in]
            n255 = Number To Decimal String(number=w569) -> (decimal integer string=w568:string)  [unwired: 1 in]
            n256 = Number To Fractional String(number=w566) -> (F-format string=w567:string)  [unwired: 3 in]
            n257 = Number To Fractional String(number=w562) -> (F-format string=w563:string)  [unwired: 3 in]
            n258 = Number To Fractional String(number=w560) -> (F-format string=w561:string)  [unwired: 3 in]
            n259 = Number To Fractional String(number=w558) -> (F-format string=w559:string)  [unwired: 3 in]
            n260 = Number To Decimal String(number=w582) -> (decimal integer string=w583:string)  [unwired: 1 in]
            n261 = Build Array(w555, w578, w557, w553, w549, w579, w580, w535, w534, w527, w531, w530, w533, w518, w572, w575, w585, w576, w528, w583, w571, w565, w568, w567, w563, w561, w559) -> (w581:string[])
            n262 = local write "Current \nRecord"(w581) -> ()
          }
          frame Enabled {
          }
        }
        n263 = local read "Lin-Vg Array-Used"() -> (w435:dbl[])
        n264 = local read "Sat Id-Log-Used"() -> (w439:dbl[])
        n265 = local read "New: Dielectric"() -> (w432:dbl)
        n266 = local read "Vg Array-Log-Used"() -> (w438:dbl[])
        n267 = local read "New: Length"() -> (w434:dbl)
        n268 = local read "New: Width"() -> (w431:dbl)
        n269 = local read "Lin Id-Used"() -> (w436:dbl[])
        n270 = local read "New: Dielectric"() -> (w428:dbl)
        n271 = local read "Lin Vd"() -> (w430:dbl)
        n272 = local read "Sat Vg Array-Used"() -> (w441:dbl[])
        n273 = local read "New: Dielectric"() -> (w426:dbl)
        n274 = local read "New: Length"() -> (w442:dbl)
        n275 = local read "New: Width"() -> (w444:dbl)
        n276 = local read "Sat Id-Used"() -> (w440:dbl[])
        n277 = call "Mobility-Vt-Used Pts_Linear.vi"("Width"=w431, "Length"=w434, "Vd"=w430, "Dielectric (d)"=w432, "Sat Id Used"=w436, "Vg Used"=w435) -> ("Vt"=w437:dbl, "Mobility"=w433:dbl)  [unwired: 3 in, 1 out]
        n278 = call "STS-Used.vi"("Id Used"=w439, "Vg-Used"=w438) -> ("STS"=w429:dbl)  [unwired: 9 in]
        n279 = local write "New: Mobility-Lin"(w433) -> ()
        n280 = local write "New: VT-Lin"(w437) -> ()
        n281 = call "Mobility-Vt-Used Pts_Saturation.vi"("Width"=w444, "Length"=w442, "Dielectric (d)"=w426, "Sat Id Used"=w440, "Vg Used"=w441) -> ("Vt"=w427:dbl, "Mobility"=w443:dbl)  [unwired: 4 in, 1 out]
        n282 = local write "New: STS"(w429) -> ()
        n283 = local write "New: Mobility-Sat"(w443) -> ()
        n284 = local write "New: VT-Sat"(w427) -> ()
        n285 = call "Trap Density_VT.vi"("VT"=w427, "Dielectric"=w426) -> ("Trap Density-VT"=w425:dbl)
        n286 = local read "Manual-Temp"() -> (w422:bool)
        n287 = local read "Rec: Temp"() -> (w423:dbl)
        n288 = local write "New: Trap Density-VT"(w425) -> ()
        n289 = case shown="False" w422 {
          tunnel: w423 -> [w603 _]
          tunnel: [w600 w607] -> w421
          frame False {
            n290 = local read "Rec: Temp"() -> (w601:dbl)
            n291 = property on="New: Temp" class="DigNum (strict)"("DisabledEnum"=1) -> ()  [unwired: 2 in, 2 out]
            n292 = Equal To 0?(x=w601) -> (x = 0?=w602:bool)
            n293 = local write "New: Temp"(w603) -> ()
            n294 = case shown="True" w602 {
              tunnel: [w604 w605] -> w600
              tunnel: w601 -> [w604 _]
              frame False {
              }
              frame True {
                n295 = local read "Room Temp"() -> (w605:dbl)
              }
            }
            n296 = local write "New: Temp"(w600) -> ()
          }
          frame True {
            n297 = property on="New: Temp" class="DigNum (strict)"("DisabledEnum"=0) -> ()  [unwired: 2 in, 2 out]
            n298 = local read "New: Temp"() -> (w607:dbl)
          }
        }
        n299 = call "Trap Density_STS.vi"("Temp (T) [K]"=w421, "S.T.S. (S)"=w429, "Dielectric"=w428) -> ("Trap Density (N)"=w424:dbl)  [unwired: 8 in]
        n300 = local write "New: Trap Density-STS"(w424) -> ()
        n301 = property on="Image Out" class="ImageControl"() -> ("ZoomSingle"=w485:cluster{"X":sgl, "Y":sgl})  [unwired: 2 in, 2 out]
        n302 = property on="Image Out" class="ImageControl"() -> ("Bounds"=w486:T13)  [unwired: 2 in, 2 out]
        n303 = call <vilib>:"Intialize Keyboard.vi"() -> ("device ID"=w497:refnum<k1>)  [unwired: 10 in, 1 out]
        n304 = property on="Image Out" class="ImageControl"() -> ("Image Center Position"=w492:cluster{"X":u32, "Y":u32})  [unwired: 2 in, 2 out]
        n305 = call-poly <vilib>:"Acquire Input Data.vi"("device ID"=w497) -> ("keys pressed"=w496:T14)  [unwired: 16 in, 2 out]
        n306 = Unbundle(w486) -> ("Width"=w483:u32, "Height"=w482:u32)
        n307 = Unbundle(w485) -> ("X"=w460:sgl, "Y"=w484:sgl)
        n308 = Index Array(array=w496) -> (element=w500:T15)  [unwired: 1 in]
        n309 = event shown="[1] \"Undo Button\": Mouse Down" {
          selector: _ -> [_ _ _ _ _ _ _]
          dyn-events: _ -> [_ _ _ _ _ _ _]
          timeout: 10 -> [_ _ _ _ _ _ _]
          event "Remove Button": Mouse Down {
            w620 = 0
            n310 = event-data() -> ()  [unwired: 1 in, 7 out]
            n311 = property on="Image Out" class="ImageControl"() -> ("ROI"=w618:T12)  [unwired: 2 in, 2 out]
            n312 = Unbundle(w618) -> ("Global Rectangle"=w621:i32[], "Contours"=w623:T16)
            n313 = Reverse 1D Array(array=w621) -> (reversed array=w622:i32[])
            n314 = Reverse 1D Array(array=w623) -> (reversed array=w624:T16)
            n315 = Delete From Array(array=w622, index=w620) -> (array with subset deleted=w625:i32[])  [unwired: 1 in, 1 out]
            n316 = Delete From Array(array=w624, index=w620) -> (array with subset deleted=w626:T16)  [unwired: 1 in, 1 out]
            n317 = Reverse 1D Array(array=w625) -> (reversed array=w627:i32[])
            n318 = Reverse 1D Array(array=w626) -> (reversed array=w628:T16)
            n319 = Bundle(w627, w628) -> (w619:T17)  [unwired: 1 in]
            n320 = local write "ROI Descriptor out"(w618) -> ()
            n321 = local write "ROI Descriptor"(w619) -> ()
            n322 = property on="Image Out" class="ImageControl"("ROI"=w619) -> ()  [unwired: 2 in, 2 out]
          }
          event "Undo Button": Mouse Down {
            n323 = event-data() -> ()  [unwired: 1 in, 7 out]
            n324 = invoke on="Image Out" class="ImageControl" method="Clear ROI"() -> ()  [unwired: 3 in, 3 out]
          }
          event "Image Folder": Value Change {
            n325 = event-data() -> ()  [unwired: 1 in, 5 out]
            n326 = local read "Image File"() -> (w630:path)
            n327 = call "Vision Acquisition"("Image Path"=w630) -> ("Image Out"=w629:T2)  [unwired: 25 in, 1 out]
            n328 = local write "Image Out 2"(w629) -> ()
            n329 = local write "Image Out"(w629) -> ()
            n330 = invoke on="Image Out" class="ImageControl" method="Clear ROI"() -> ()  [unwired: 3 in, 3 out]
          }
          event "Zoom": Value Change {
            n331 = event-data() -> ()  [unwired: 1 in, 5 out]
            n332 = local read "Zoom"() -> (w631:i16)
            n333 = Bundle("Zoom"=w631, "Zoom"=w631) -> (w632:cluster{"Zoom":i16, "Zoom":i16})  [unwired: 1 in]
            n334 = property on="Image Out" class="ImageControl"("ZoomInteger"=w632) -> ()  [unwired: 2 in, 2 out]
          }
          event Timeout {
            n335 = event-data() -> ()  [unwired: 1 in, 2 out]
          }
          event "Image Out": Mouse Enter {
            (unwired) 6
            n336 = event-data() -> ()  [unwired: 1 in, 3 out]
            n337 = call "Simulate_Keyboard.vi"("Action"=0, "Virtual Key"=162) -> ()  [unwired: 7 in, 1 out]
          }
          event "Image Out": Mouse Leave {
            n338 = event-data() -> ()  [unwired: 1 in, 3 out]
            n339 = flat-sequence {
              frame #0 {
                n340 = Wait (ms)(milliseconds to wait=10) -> ()  [unwired: 1 out]
              }
              frame #1 {
                (unwired) 6
                n341 = call "Simulate_Keyboard.vi"("Action"=2, "Virtual Key"=162) -> ()  [unwired: 7 in, 1 out]
              }
            }
          }
        }
        n342 = Divide(x=w483, y=w460) -> (x/y=w473:sgl)
        n343 = Multiply(x=w473, y=0.5) -> (x*y=w479:dbl)
        n344 = Divide(x=w482, y=w484) -> (x/y=w472:sgl)
        n345 = Multiply(x=w472, y=0.5) -> (x*y=w478:dbl)
        n346 = Unbundle(w492) -> ("X"=w474:u32, "Y"=w475:u32)
        n347 = Subtract(x=w475, y=w478) -> (x-y=w476:dbl)
        n348 = Subtract(x=w474, y=w479) -> (x-y=w477:dbl)
        n349 = Add(x=w477, y=w473) -> (x+y=w491:dbl)
        n350 = Add(x=w476, y=w472) -> (x+y=w490:dbl)
        n351 = Reciprocal(x=w460) -> (1/x=w459:sgl)
        n352 = event shown="[12] \"Save Changes? 2\": Mouse Down" {
          selector: _ -> [_ _ _ _ _ _ _ _ _ _ _ _ _ _ _ _]
          dyn-events: _ -> [_ _ _ _ _ _ _ _ _ _ _ _ _ _ _ _]
          timeout: 10 -> [_ _ _ _ _ _ _ _ _ _ _ _ _ _ _ _]
          tunnel: [_ _ _ _ _ _ _ _ _ _ _ _ _ TRUE _ TRUE] -> w517
          event Timeout {
            n353 = event-data() -> ()  [unwired: 1 in, 2 out]
          }
          event "Down Button": Mouse Down {
            w977 = 0
            n354 = event-data() -> ()  [unwired: 1 in, 7 out]
            n355 = local read "Transfer File"() -> (w982:path)
            n356 = Strip Path(path=w982) -> (stripped path=w973:path, name=w991:string)
            n357 = local write "Transfer Folder"(w973) -> ()
            n358 = List Folder(path=w973) -> (filenames=w987:string[], error out=w927:errorcluster)  [unwired: 3 in, 2 out]
            n359 = local read "Folder Index"() -> (w929:dbl)
            n360 = Array Size(array=w987) -> (size(s)=w983:i32)
            n361 = Search 1D Array(1D array=w987, element=w991) -> (index of element=w984:i32)  [unwired: 1 in]
            n362 = property on="Image Out" class="ImageControl"() -> (error out=w930:errorcluster, "Image Center Position"=w934:cluster{"X":u32, "Y":u32})  [unwired: 2 in, 1 out]
            n363 = Decrement(x=w983) -> (x-1=w985:i32)
            n364 = Equal?(x=w984, y=w985) -> (x = y?=w986:bool)
            n365 = invoke on="Image Out" class="ImageControl" method="Clear ROI"() -> ()  [unwired: 3 in, 3 out]
            n366 = case shown="False" w986 {
              tunnel: w929 -> [w1144 _]
              tunnel: [w1143 0] -> w928
              tunnel: w927 -> [w1142 w1145]
              tunnel: [w1142 w1145] -> w926
              frame False {
                n367 = Increment(x=w1144) -> (x+1=w1143:dbl)
              }
              frame True {
              }
            }
            n368 = Unbundle(w934) -> ("X"=w932:u32)  [unwired: 1 out]
            n369 = local write "Folder Index"(w928) -> ()
            n370 = Bundle("X"=w932, 0) -> (w933:cluster{"X":u32, i32})  [unwired: 1 in]
            n371 = property on="Image Out" class="ImageControl"(error in=w930, "Image Center Position"=w933) -> ()  [unwired: 1 in, 2 out]
            n372 = Path To String(path=w973) -> (string=w992:string)
            n373 = Index Array(array=w987, index=w928) -> (element=w988:string)
            n374 = local write "Data Name:"(w988) -> ()
            n375 = Concatenate Strings(w992, "\\", w988) -> (w990:string)
            n376 = String To Path(string=w990) -> (path=w901:path)
            n377 = call "Recorded Values.vi"("Path"=w901) -> ("Recorded Char"=w994:T6, "Recorded Prop"=w995:T7, "Fabrication Prop"=w993:T8)  [unwired: 8 in]
            n378 = Unbundle By Name(w994) -> ("Mobility-Sat"=w1007:dbl, "Moblitity-Lin"=w1008:dbl, "On/Off"=w1009:dbl, "Off Current"=w1010:dbl, "Vt-Sat"=w896:dbl, "STS"=w1011:dbl, "Trap Density-VT"=w1012:dbl, "Trap Density-STS"=w1013:dbl)
            n379 = Unbundle By Name(w993) -> ("Date Created"=w1014:string, "Material"=w996:string, "Solvent"=w997:string, "Concentration"=w998:dbl, "Method"=w999:string, "Dielectric (nm)"=w1000:dbl, "Treatment"=w1001:string, "Comments"=w1002:string)
            n380 = Unbundle By Name(w995) -> ("Date Recorded"=w1003:string, "Index"=w1004:string, "Length"=w1005:dbl, "Width"=w1006:dbl, "Sample Temp"=w898:dbl)
            n381 = local write "Date Created"(w1014) -> ()
            n382 = local write "Rec: Off I-Sat"(w1010) -> ()
            n383 = local write "Rec: Comments"(w1002) -> ()
            n384 = local write "Rec: Material"(w996) -> ()
            n385 = local write "Rec: VT-Sat"(w896) -> ()
            n386 = local write "Rec: Concentration"(w998) -> ()
            n387 = local write "Rec: Method"(w999) -> ()
            n388 = local write "Rec: Dielectric (d)"(w1000) -> ()
            n389 = local write "Surface Treatment:"(w1001) -> ()
            n390 = local write "Index"(w1004) -> ()
            n391 = local write "Rec: Mobility-Sat"(w1007) -> ()
            n392 = local write "Rec: Mobility-Lin"(w1008) -> ()
            n393 = local write "Rec: On/Off"(w1009) -> ()
            n394 = local write "Rec: STS"(w1011) -> ()
            n395 = local write "Rec: Trap Density-VT"(w1012) -> ()
            n396 = local write "Rec: Trap Density-STS"(w1013) -> ()
            n397 = local write "Rec: Solvent"(w997) -> ()
            n398 = local write "Date Recorded"(w1003) -> ()
            n399 = local write "Rec: Length"(w1005) -> ()
            n400 = local write "Rec: Width"(w1006) -> ()
            n401 = local write "Rec: Temp"(w898) -> ()
            n402 = Equal To 0?(x=w898) -> (x = 0?=w899:bool)
            n403 = case shown="True" w899 {
              tunnel: [w1015 w1016] -> w897
              tunnel: w898 -> [w1015 _]
              frame False {
              }
              frame True {
                n404 = local read "Room Temp"() -> (w1016:dbl)
              }
            }
            n405 = local read "NumPoints Log"() -> (w922:dbl)
            n406 = local write "Transfer File"(w901) -> ()
            n407 = local read "Num Pts"() -> (w925:dbl)
            n408 = call-poly <vilib>:"Read From Spreadsheet File.vi"("file path (dialog if empty)"=w901) -> ("all rows"=w979:string[][])  [unwired: 6 in, 4 out]
            n409 = call "Mobility-Vt Calculator-File.vi"("NumPts"=w925, "Path"=w901) -> ("Graph Cluster"=w894:T9, "Output"=w924:T10, "Index-Sat"=w923:dbl, "Index-Lin"=w909:dbl)  [unwired: 5 in, 1 out]
            n410 = local read "New: Dielectric"() -> (w906:dbl)
            n411 = call "STS Calculator-File.vi"("NumPts"=w922, "Path"=w901) -> ("STS Index-Sat"=w921:dbl, "XY Graph-Sat"=w920:cluster{dbl[], dbl[]}[], "Ouput"=w919:cluster{"STS-Sat":dbl, "STS-Lin":dbl})  [unwired: 5 in, 2 out]
            n412 = local write "Sat-Trans Slider"(w923) -> ()
            n413 = Unbundle By Name(w924) -> ("Mobility-Sat"=w918:dbl, "Vt-Sat"=w905:dbl, "Mobility-Lin"=w917:dbl, "Vt-Lin"=w916:dbl, "Off I-Sat"=w902:dbl, "On/Off I-Sat"=w895:dbl)
            n414 = Unbundle By Name(w919) -> ("STS-Sat"=w900:dbl)  [unwired: 1 out]
            n415 = local write "Index 2"(w921) -> ()
            n416 = local write "MobVi Index"(w923) -> ()
            n417 = local write "Log-Sat"(w920) -> ()
            n418 = Array Size(array=w979) -> (size(s)=w978:i32[])
            n419 = Unbundle By Name(w894) -> ("Raw Sat"=w891:cluster{dbl[], dbl[]}[], "Sqrt Sat"=w893:cluster{dbl[], dbl[]}[], "Log Sat"=w890:cluster{dbl[], dbl[]}[], "Raw Lin"=w889:cluster{dbl[], dbl[]}[], "Sqrt Lin"=w892:cluster{dbl[], dbl[]}[], "Log Lin"=w888:cluster{dbl[], dbl[]}[])
            n420 = local write "Sqrt-Sat"(w893) -> ()
            n421 = call "Trap Density_VT.vi"("VT"=w905, "Dielectric"=w906) -> ("Trap Density-VT"=w904:dbl)
            n422 = call "Trap Density_STS.vi"("Temp (T) [K]"=w897, "S.T.S. (S)"=w900, "Dielectric"=w906) -> ("Trap Density (N)"=w903:dbl)  [unwired: 8 in]
            n423 = local write "New: STS"(w900) -> ()
            n424 = local write "Calc: STS"(w900) -> ()
            n425 = local write "Calc: Mobility-Sat"(w918) -> ()
            n426 = local write "Calc: Off I-Sat"(w916) -> ()
            n427 = local write "Calc: Mobility-Lin"(w917) -> ()
            n428 = Index Array(array=w978, index=w977) -> (element=w959:i32)
            n429 = Decimate 1D Array(w920) -> (w953:cluster{dbl[], dbl[]}[])  [unwired: 1 out]
            n430 = Decimate 1D Array(w893) -> (w963:cluster{dbl[], dbl[]}[])  [unwired: 1 out]
            n431 = local write "Calc: Off I-Sat"(w902) -> ()
            n432 = local write "Calc: On/Off"(w895) -> ()
            n433 = Decimate 1D Array(w892) -> (w915:cluster{dbl[], dbl[]}[])  [unwired: 1 out]
            n434 = local write "Calc: VT-Sat"(w905) -> ()
            n435 = Array Subset(array=w979, index (row)=w977, index (col)=w977, length (col)=3) -> (w980:string[][])  [unwired: 1 in]
            n436 = local write "Calc: Trap Density-VT"(w904) -> ()
            n437 = local write "Calc: Trap Density-STS"(w903) -> ()
            n438 = local write "New: Trap Density-STS"(w903) -> ()
            n439 = local write "New: Trap Density-VT"(w904) -> ()
            n440 = Array To Cluster(array=w953) -> (cluster=w951:T11)
            n441 = Array To Cluster(array=w963) -> (cluster=w965:T11)
            n442 = local write "Raw- Sat"(w891) -> ()
            n443 = local write "Sqrt-Lin"(w892) -> ()
            n444 = local write "Raw- Lin"(w889) -> ()
            n445 = local write "Log-Sat"(w890) -> ()
            n446 = local write "New: VT-Lin"(w916) -> ()
            n447 = local write "Log-Lin"(w888) -> ()
            n448 = local write "New: VT-Sat"(w905) -> ()
            n449 = local write "New: Mobility-Sat"(w918) -> ()
            n450 = local write "New: Mobility-Lin"(w917) -> ()
            n451 = Reshape Array(w980, w959) -> (w966:string[])
            n452 = Array To Cluster(array=w915) -> (cluster=w914:T11)
            n453 = Subtract(x=w959, y=20) -> (x-y=w958:i32)
            n454 = property on="Sat-Trans Slider" class="Slide (strict)"("Scale.Maximum"=w958) -> ()  [unwired: 2 in, 2 out]
            n455 = Unbundle(w951) -> ("[0]"=w952:cluster{dbl[], dbl[]})  [unwired: 8 out]
            n456 = Unbundle(w965) -> ("[0]"=w964:cluster{dbl[], dbl[]})  [unwired: 8 out]
            n457 = Unbundle(w914) -> ("[0]"=w911:cluster{dbl[], dbl[]})  [unwired: 8 out]
            n458 = Search 1D Array(1D array=w966, element="Index:") -> (index of element=w974:i32)  [unwired: 1 in]
            n459 = local read "Num Pts"() -> (w910:dbl)
            n460 = Unbundle(w911) -> (w913:dbl[], w912:dbl[])
            n461 = Increment(x=w974) -> (x+1=w975:i32)
            n462 = Unbundle(w952) -> (w950:dbl[], w949:dbl[])
            n463 = Unbundle(w964) -> (w955:dbl[], w954:dbl[])
            n464 = Array Subset(array=w913, index=w909, length=w910) -> (w908:dbl[])
            n465 = Array Subset(array=w912, index=w909, length=w910) -> (w907:dbl[])
            n466 = Array Subset(array=w950, index=w921, length=w922) -> (w957:dbl[])
            n467 = Array Subset(array=w949, index=w921, length=w922) -> (w956:dbl[])
            n468 = Array Subset(array=w955, index=w923, length=w925) -> (w962:dbl[])
            n469 = Array Subset(array=w954, index=w923, length=w925) -> (w961:dbl[])
            n470 = Index Array(array=w966, index=w975) -> (element=w938:string)
            n471 = local write "Lin-Vg Array-Used"(w908) -> ()
            n472 = local write "Sat Vg Array-Used"(w962) -> ()
            n473 = local write "Vg Array-Log-Used"(w956) -> ()
            n474 = local write "Lin Id-Used"(w907) -> ()
            n475 = local read "Image Folder"() -> (w936:path)
            n476 = local write "Sat Id-Used"(w961) -> ()
            n477 = local write "Sat Id-Log-Used"(w957) -> ()
            n478 = List Folder(path=w936, error in=w926) -> (filenames=w972:string[], error out=w939:errorcluster)  [unwired: 2 in, 2 out]
            n479 = while {
              tunnel: w972 -> [w1029]
              tunnel: w938 -> [w1027]
              tunnel: [w1026] -> _
              tunnel: [w1026] -> w971
              tunnel: w959 -> [w1025]
              i -> [w1026]
              stop <- w1022 stop-if-true
              n480 = Index Array(array=w1029, index=w1026) -> (element=w1030:string)
              n481 = xnode "Match Regular Expression"("input string"=w1030, "regular expression"=w1027) -> ("whole match"=w1028:string)  [unwired: 4 in, 4 out]
              n482 = Equal?(x=w1028, y=w1027) -> (x = y?=w1024:bool)
              n483 = Equal?(x=w1025, y=w1026) -> (x = y?=w1023:bool)
              n484 = Or(x=w1024, y=w1023) -> (x .or. y?=w1022:bool)
            }
            n485 = Build Path(base path=w936, name or relative path="ROI") -> (appended path=w935:path)
            n486 = Path To String(path=w936) -> (string=w969:string)
            n487 = Index Array(array=w972, index=w971) -> (element=w947:string)
            n488 = invoke on="Image Out" class="ImageControl" method="Clear ROI"(error in=w939) -> (error out=w942:errorcluster)  [unwired: 2 in, 2 out]
            n489 = local write "Image Name"(w947) -> ()
            n490 = Build Path(base path=w935, name or relative path=w938) -> (appended path=w943:path)
            n491 = call <vilib>:"Check if File or Folder Exists.vi"("error in (no error)"=w942, "path"=w943) -> ("file or folder exists?"=w940:bool, "dup path"=w941:path)  [unwired: 7 in, 1 out]
            n492 = Concatenate Strings(w969, "\\", w947) -> (w968:string)
            n493 = case shown="False" w940 {
              tunnel: w941 -> [_ w1017]
              frame False {
              }
              frame True {
                n494 = Read from Text File(file (use dialog)=w1017) -> (text=w1021:string)  [unwired: 3 in, 3 out]
                n495 = property on="Image Out" class="ImageControl"() -> ("ROI"=w1018:T12)  [unwired: 2 in, 2 out]
                n496 = Unflatten From String(type=w1018, binary string=w1021) -> (value=w1019:T12, error out=w1020:errorcluster)  [unwired: 3 in, 1 out]
                n497 = property on="Image Out" class="ImageControl"(error in=w1020, "ROI"=w1019) -> ()  [unwired: 1 in, 2 out]
              }
            }
            n498 = String To Path(string=w968) -> (path=w946:path)
            n499 = Empty String/Path?(string/path=w947) -> (empty?=w948:bool)
            n500 = local read "No Image File"() -> (w944:path)
            n501 = Select(t=w944, s=w948, f=w946) -> (s? t:f=w945:path)
            n502 = local write "Image File"(w945) -> ()
            n503 = call "Vision Acquisition4"("Image Path"=w945) -> ("Image Out"=w970:T2)  [unwired: 25 in, 1 out]
            n504 = local write "Image Out"(w970) -> ()
            n505 = local write "Image Out 2"(w970) -> ()
          }
          event "Transfer File": Value Change {
            w1258 = 0
            n506 = event-data() -> ()  [unwired: 1 in, 5 out]
            n507 = local read "Transfer File"() -> (w1254:path)
            n508 = Strip Path(path=w1254) -> (stripped path=w1253:path, name=w1267:string)
            n509 = local write "Transfer Folder"(w1253) -> ()
            n510 = property on="Image Out" class="ImageControl"() -> (error out=w1209:errorcluster, "Image Center Position"=w1213:cluster{"X":u32, "Y":u32})  [unwired: 2 in, 1 out]
            n511 = List Folder(path=w1253) -> (filenames=w1263:string[], error out=w1219:errorcluster)  [unwired: 3 in, 2 out]
            n512 = Search 1D Array(1D array=w1263, element=w1267) -> (index of element=w1208:i32)  [unwired: 1 in]
            n513 = local write "Folder Index"(w1208) -> ()
            n514 = Unbundle(w1213) -> ("X"=w1211:u32)  [unwired: 1 out]
            n515 = Path To String(path=w1253) -> (string=w1268:string)
            n516 = Index Array(array=w1263, index=w1208) -> (element=w1264:string)
            n517 = Bundle("X"=w1211, 0) -> (w1212:cluster{"X":u32, i32})  [unwired: 1 in]
            n518 = local write "Data Name:"(w1264) -> ()
            n519 = property on="Image Out" class="ImageControl"(error in=w1209, "Image Center Position"=w1212) -> ()  [unwired: 1 in, 2 out]
            n520 = Concatenate Strings(w1268, "\\", w1264) -> (w1266:string)
            n521 = String To Path(string=w1266) -> (path=w1160:path)
            n522 = call "Recorded Values.vi"("Path"=w1160) -> ("Recorded Char"=w1206:T6, "Recorded Prop"=w1205:T7, "Fabrication Prop"=w1207:T8)  [unwired: 8 in]
            n523 = Unbundle By Name(w1206) -> ("Mobility-Sat"=w1193:dbl, "Moblitity-Lin"=w1192:dbl, "On/Off"=w1191:dbl, "Off Current"=w1190:dbl, "Vt-Sat"=w1156:dbl, "STS"=w1189:dbl, "Trap Density-VT"=w1188:dbl, "Trap Density-STS"=w1187:dbl)
            n524 = Unbundle By Name(w1207) -> ("Date Created"=w1186:string, "Material"=w1204:string, "Solvent"=w1203:string, "Concentration"=w1202:dbl, "Method"=w1201:string, "Dielectric (nm)"=w1200:dbl, "Treatment"=w1199:string, "Comments"=w1198:string)
            n525 = Unbundle By Name(w1205) -> ("Date Recorded"=w1197:string, "Index"=w1196:string, "Length"=w1195:dbl, "Width"=w1194:dbl, "Sample Temp"=w1158:dbl)
            n526 = local write "Date Created"(w1186) -> ()
            n527 = local write "Rec: Material"(w1204) -> ()
            n528 = local write "Rec: Off I-Sat"(w1190) -> ()
            n529 = local write "Rec: Comments"(w1198) -> ()
            n530 = local write "Rec: VT-Sat"(w1156) -> ()
            n531 = local write "Rec: Concentration"(w1202) -> ()
            n532 = local write "Rec: Method"(w1201) -> ()
            n533 = local write "Rec: Dielectric (d)"(w1200) -> ()
            n534 = local write "Surface Treatment:"(w1199) -> ()
            n535 = local write "Index"(w1196) -> ()
            n536 = local write "Rec: Mobility-Sat"(w1193) -> ()
            n537 = local write "Rec: Mobility-Lin"(w1192) -> ()
            n538 = local write "Rec: On/Off"(w1191) -> ()
            n539 = local write "Rec: STS"(w1189) -> ()
            n540 = local write "Rec: Trap Density-VT"(w1188) -> ()
            n541 = local write "Rec: Trap Density-STS"(w1187) -> ()
            n542 = local write "Rec: Solvent"(w1203) -> ()
            n543 = local write "Date Recorded"(w1197) -> ()
            n544 = local write "Rec: Length"(w1195) -> ()
            n545 = local write "Rec: Width"(w1194) -> ()
            n546 = local write "Rec: Temp"(w1158) -> ()
            n547 = Equal To 0?(x=w1158) -> (x = 0?=w1159:bool)
            n548 = case shown="False" w1159 {
              tunnel: [w1269 w1270] -> w1157
              tunnel: w1158 -> [w1269 _]
              frame False {
              }
              frame True {
                n549 = local read "Room Temp"() -> (w1270:dbl)
              }
            }
            n550 = local read "NumPoints Log"() -> (w1182:dbl)
            n551 = local write "Transfer File"(w1160) -> ()
            n552 = local read "Num Pts"() -> (w1183:dbl)
            n553 = call-poly <vilib>:"Read From Spreadsheet File.vi"("file path (dialog if empty)"=w1160) -> ("all rows"=w1260:string[][])  [unwired: 6 in, 4 out]
            n554 = local read "New: Dielectric"() -> (w1166:dbl)
            n555 = call "STS Calculator-File.vi"("NumPts"=w1182, "Path"=w1160) -> ("STS Index-Sat"=w1180:dbl, "XY Graph-Sat"=w1181:cluster{dbl[], dbl[]}[], "Ouput"=w1179:cluster{"STS-Sat":dbl, "STS-Lin":dbl})  [unwired: 5 in, 2 out]
            n556 = call "Mobility-Vt Calculator-File.vi"("NumPts"=w1183, "Path"=w1160) -> ("Graph Cluster"=w1153:T9, "Output"=w1184:T10, "Index-Sat"=w1185:dbl, "Index-Lin"=w1172:dbl)  [unwired: 5 in, 1 out]
            n557 = Unbundle By Name(w1184) -> ("Mobility-Sat"=w1168:dbl, "Vt-Sat"=w1162:dbl, "Mobility-Lin"=w1167:dbl, "Vt-Lin"=w1154:dbl, "Off I-Sat"=w1161:dbl, "On/Off I-Sat"=w1155:dbl)
            n558 = local write "Index 2"(w1180) -> ()
            n559 = Unbundle By Name(w1179) -> ("STS-Sat"=w1163:dbl)  [unwired: 1 out]
            n560 = local write "MobVi Index"(w1185) -> ()
            n561 = local write "Log-Sat"(w1181) -> ()
            n562 = local write "Sat-Trans Slider"(w1185) -> ()
            n563 = Array Size(array=w1260) -> (size(s)=w1259:i32[])
            n564 = call "Trap Density_VT.vi"("VT"=w1162, "Dielectric"=w1166) -> ("Trap Density-VT"=w1165:dbl)
            n565 = call "Trap Density_STS.vi"("Temp (T) [K]"=w1157, "S.T.S. (S)"=w1163, "Dielectric"=w1166) -> ("Trap Density (N)"=w1164:dbl)  [unwired: 8 in]
            n566 = local write "Calc: Mobility-Lin"(w1167) -> ()
            n567 = local write "Calc: Mobility-Sat"(w1168) -> ()
            n568 = local write "Calc: VT-Sat"(w1162) -> ()
            n569 = local write "Calc: Off I-Sat"(w1161) -> ()
            n570 = local write "Calc: VT-Lin"(w1154) -> ()
            n571 = local write "Calc: On/Off"(w1155) -> ()
            n572 = local write "Calc: STS"(w1163) -> ()
            n573 = Unbundle By Name(w1153) -> ("Raw Sat"=w1150:cluster{dbl[], dbl[]}[], "Sqrt Sat"=w1151:cluster{dbl[], dbl[]}[], "Log Sat"=w1149:cluster{dbl[], dbl[]}[], "Raw Lin"=w1148:cluster{dbl[], dbl[]}[], "Sqrt Lin"=w1152:cluster{dbl[], dbl[]}[], "Log Lin"=w1147:cluster{dbl[], dbl[]}[])
            n574 = Decimate 1D Array(w1152) -> (w1178:cluster{dbl[], dbl[]}[])  [unwired: 1 out]
            n575 = local write "Calc: Trap Density-VT"(w1165) -> ()
            n576 = local write "Calc: Trap Density-STS"(w1164) -> ()
            n577 = local write "New: Trap Density-STS"(w1164) -> ()
            n578 = local write "New: Trap Density-VT"(w1165) -> ()
            n579 = local write "Sqrt-Lin"(w1152) -> ()
            n580 = local write "New: VT-Sat"(w1162) -> ()
            n581 = Decimate 1D Array(w1181) -> (w1234:cluster{dbl[], dbl[]}[])  [unwired: 1 out]
            n582 = Index Array(array=w1259, index=w1258) -> (element=w1240:i32)
            n583 = Decimate 1D Array(w1151) -> (w1243:cluster{dbl[], dbl[]}[])  [unwired: 1 out]
            n584 = local write "Sqrt-Sat"(w1151) -> ()
            n585 = local write "New: Mobility-Lin"(w1167) -> ()
            n586 = Array Subset(array=w1260, index (row)=w1258, index (col)=w1258, length (col)=3) -> (w1261:string[][])  [unwired: 1 in]
            n587 = local write "New: VT-Lin"(w1154) -> ()
            n588 = Array To Cluster(array=w1178) -> (cluster=w1177:T11)
            n589 = local write "New: STS"(w1163) -> ()
            n590 = local write "New: Mobility-Sat"(w1168) -> ()
            n591 = Array To Cluster(array=w1234) -> (cluster=w1232:T11)
            n592 = Array To Cluster(array=w1243) -> (cluster=w1245:T11)
            n593 = Reshape Array(w1261, w1240) -> (w1246:string[])
            n594 = Subtract(x=w1240, y=20) -> (x-y=w1238:i32)
            n595 = local write "Raw- Sat"(w1150) -> ()
            n596 = Unbundle(w1177) -> ("[0]"=w1176:cluster{dbl[], dbl[]})  [unwired: 8 out]
            n597 = local write "Raw- Lin"(w1148) -> ()
            n598 = local write "Log-Sat"(w1149) -> ()
            n599 = local read "Num Pts"() -> (w1173:dbl)
            n600 = property on="Sat-Trans Slider" class="Slide (strict)"("Scale.Maximum"=w1238) -> ()  [unwired: 2 in, 2 out]
            n601 = local write "Log-Lin"(w1147) -> ()
            n602 = Unbundle(w1176) -> (w1175:dbl[], w1174:dbl[])
            n603 = Unbundle(w1232) -> ("[0]"=w1233:cluster{dbl[], dbl[]})  [unwired: 8 out]
            n604 = Unbundle(w1245) -> ("[0]"=w1244:cluster{dbl[], dbl[]})  [unwired: 8 out]
            n605 = Search 1D Array(1D array=w1246, element="Index:") -> (index of element=w1255:i32)  [unwired: 1 in]
            n606 = local read "Num Pts"() -> (w1169:dbl)
            n607 = Array Subset(array=w1175, index=w1172, length=w1173) -> (w1171:dbl[])
            n608 = Array Subset(array=w1174, index=w1172, length=w1173) -> (w1170:dbl[])
            n609 = Increment(x=w1255) -> (x+1=w1256:i32)
            n610 = Unbundle(w1233) -> (w1230:dbl[], w1229:dbl[])
            n611 = Unbundle(w1244) -> (w1231:dbl[], w1235:dbl[])
            n612 = local read "Image Folder"() -> (w1215:path)
            n613 = local write "Lin-Vg Array-Used"(w1171) -> ()
            n614 = Array Subset(array=w1230, index=w1180, length=w1182) -> (w1237:dbl[])
            n615 = Array Subset(array=w1229, index=w1180, length=w1182) -> (w1236:dbl[])
            n616 = Array Subset(array=w1231, index=w1185, length=w1169) -> (w1242:dbl[])
            n617 = Array Subset(array=w1235, index=w1185, length=w1169) -> (w1241:dbl[])
            n618 = Index Array(array=w1246, index=w1256) -> (element=w1217:string)
            n619 = local write "Lin Id-Used"(w1170) -> ()
            n620 = local write "Sat Vg Array-Used"(w1242) -> ()
            n621 = local write "Vg Array-Log-Used"(w1236) -> ()
            n622 = local write "Sat Id-Log-Used"(w1237) -> ()
            n623 = local write "Sat Id-Used"(w1241) -> ()
            n624 = local write "Index"(w1217) -> ()
            n625 = List Folder(path=w1215, error in=w1219) -> (filenames=w1251:string[], error out=w1218:errorcluster)  [unwired: 2 in, 2 out]
            n626 = Build Path(base path=w1215, name or relative path="ROI") -> (appended path=w1214:path)
            n627 = invoke on="Image Out" class="ImageControl" method="Clear ROI"(error in=w1218) -> (error out=w1222:errorcluster)  [unwired: 2 in, 2 out]
            n628 = Build Path(base path=w1214, name or relative path=w1217) -> (appended path=w1223:path)
            n629 = while {
              tunnel: w1251 -> [w1283]
              tunnel: w1217 -> [w1281]
              tunnel: [w1280] -> _
              tunnel: [w1280] -> w1250
              tunnel: w1240 -> [w1279]
              i -> [w1280]
              stop <- w1276 stop-if-true
              n630 = Index Array(array=w1283, index=w1280) -> (element=w1284:string)
              n631 = xnode "Match Regular Expression"("input string"=w1284, "regular expression"=w1281) -> ("whole match"=w1282:string)  [unwired: 4 in, 4 out]
              n632 = Equal?(x=w1282, y=w1281) -> (x = y?=w1278:bool)
              n633 = Equal?(x=w1279, y=w1280) -> (x = y?=w1277:bool)
              n634 = Or(x=w1278, y=w1277) -> (x .or. y?=w1276:bool)
            }
            n635 = call <vilib>:"Check if File or Folder Exists.vi"("error in (no error)"=w1222, "path"=w1223) -> ("file or folder exists?"=w1220:bool, "dup path"=w1221:path)  [unwired: 7 in, 1 out]
            n636 = case shown="True" w1220 {
              tunnel: w1221 -> [_ w1271]
              frame False {
              }
              frame True {
                n637 = Read from Text File(file (use dialog)=w1271) -> (text=w1275:string)  [unwired: 3 in, 3 out]
                n638 = property on="Image Out" class="ImageControl"() -> ("ROI"=w1272:T12)  [unwired: 2 in, 2 out]
                n639 = Unflatten From String(type=w1272, binary string=w1275) -> (value=w1273:T12, error out=w1274:errorcluster)  [unwired: 3 in, 1 out]
                n640 = property on="Image Out" class="ImageControl"(error in=w1274, "ROI"=w1273) -> ()  [unwired: 1 in, 2 out]
              }
            }
            n641 = invoke on="Image Out" class="ImageControl" method="Clear ROI"() -> ()  [unwired: 3 in, 3 out]
            n642 = Path To String(path=w1215) -> (string=w1249:string)
            n643 = Index Array(array=w1251, index=w1250) -> (element=w1227:string)
            n644 = Concatenate Strings(w1249, "\\", w1227) -> (w1248:string)
            n645 = local write "Image Name"(w1227) -> ()
            n646 = String To Path(string=w1248) -> (path=w1226:path)
            n647 = Empty String/Path?(string/path=w1227) -> (empty?=w1228:bool)
            n648 = local read "No Image File"() -> (w1224:path)
            n649 = Select(t=w1224, s=w1228, f=w1226) -> (s? t:f=w1225:path)
            n650 = local write "Image File"(w1225) -> ()
            n651 = call "Vision Acquisition3"("Image Path"=w1225) -> ("Image Out"=w1252:T2)  [unwired: 25 in, 1 out]
            n652 = local write "Image Out"(w1252) -> ()
            n653 = local write "Image Out 2"(w1252) -> ()
          }
          event "Up Button": Mouse Down {
            w1508 = 0
            n654 = event-data() -> ()  [unwired: 1 in, 5 out]
            n655 = local read "Transfer File"() -> (w1504:path)
            n656 = Strip Path(path=w1504) -> (stripped path=w1503:path, name=w1519:string)
            n657 = local write "Transfer Folder"(w1503) -> ()
            n658 = List Folder(path=w1503) -> (filenames=w1513:string[], error out=w1470:errorcluster)  [unwired: 3 in, 2 out]
            n659 = Array Size(array=w1513) -> (size(s)=w1458:i32)
            n660 = Search 1D Array(1D array=w1513, element=w1519) -> (index of element=w1514:i32)  [unwired: 1 in]
            n661 = Equal To 0?(x=w1514) -> (x = 0?=w1515:bool)
            n662 = local read "Folder Index"() -> (w1457:dbl)
            n663 = property on="Image Out" class="ImageControl"() -> (error out=w1460:errorcluster, "Image Center Position"=w1464:cluster{"X":u32, "Y":u32})  [unwired: 2 in, 1 out]
            n664 = case shown="True" w1515 {
              tunnel: w1457 -> [w1649 _]
              tunnel: [w1648 w1650] -> w1456
              tunnel: w1458 -> [_ w1651]
              frame False {
                n665 = Decrement(x=w1649) -> (x-1=w1648:dbl)
              }
              frame True {
                n666 = Decrement(x=w1651) -> (x-1=w1650:i32)
              }
            }
            n667 = Unbundle(w1464) -> ("X"=w1462:u32)  [unwired: 1 out]
            n668 = local write "Folder Index"(w1456) -> ()
            n669 = Bundle("X"=w1462, 0) -> (w1463:cluster{"X":u32, i32})  [unwired: 1 in]
            n670 = Path To String(path=w1503) -> (string=w1520:string)
            n671 = Index Array(array=w1513, index=w1456) -> (element=w1516:string)
            n672 = local write "Data Name:"(w1516) -> ()
            n673 = property on="Image Out" class="ImageControl"(error in=w1460, "Image Center Position"=w1463) -> ()  [unwired: 1 in, 2 out]
            n674 = Concatenate Strings(w1520, "\\", w1516) -> (w1518:string)
            n675 = String To Path(string=w1518) -> (path=w1408:path)
            n676 = call "Recorded Values.vi"("Path"=w1408) -> ("Recorded Char"=w1454:T6, "Recorded Prop"=w1453:T7, "Fabrication Prop"=w1455:T8)  [unwired: 8 in]
            n677 = Unbundle By Name(w1454) -> ("Mobility-Sat"=w1441:dbl, "Moblitity-Lin"=w1440:dbl, "On/Off"=w1439:dbl, "Off Current"=w1438:dbl, "Vt-Sat"=w1404:dbl, "STS"=w1437:dbl, "Trap Density-VT"=w1436:dbl, "Trap Density-STS"=w1435:dbl)
            n678 = Unbundle By Name(w1455) -> ("Date Created"=w1434:string, "Material"=w1452:string, "Solvent"=w1451:string, "Concentration"=w1450:dbl, "Method"=w1449:string, "Dielectric (nm)"=w1448:dbl, "Treatment"=w1447:string, "Comments"=w1446:string)
            n679 = Unbundle By Name(w1453) -> ("Date Recorded"=w1445:string, "Index"=w1444:string, "Length"=w1443:dbl, "Width"=w1442:dbl, "Sample Temp"=w1405:dbl)
            n680 = local write "Date Created"(w1434) -> ()
            n681 = local write "Rec: Material"(w1452) -> ()
            n682 = local write "Rec: Off I-Sat"(w1438) -> ()
            n683 = local write "Rec: Comments"(w1446) -> ()
            n684 = local write "Rec: VT-Sat"(w1404) -> ()
            n685 = local write "Rec: Solvent"(w1451) -> ()
            n686 = local write "Rec: Concentration"(w1450) -> ()
            n687 = local write "Rec: Method"(w1449) -> ()
            n688 = local write "Rec: Dielectric (d)"(w1448) -> ()
            n689 = local write "Surface Treatment:"(w1447) -> ()
            n690 = local write "Index"(w1444) -> ()
            n691 = local write "Rec: Mobility-Sat"(w1441) -> ()
            n692 = local write "Rec: Mobility-Lin"(w1440) -> ()
            n693 = local write "Rec: On/Off"(w1439) -> ()
            n694 = local write "Rec: STS"(w1437) -> ()
            n695 = local write "Rec: Trap Density-VT"(w1436) -> ()
            n696 = local write "Rec: Trap Density-STS"(w1435) -> ()
            n697 = local write "Date Recorded"(w1445) -> ()
            n698 = local write "Rec: Length"(w1443) -> ()
            n699 = local write "Rec: Width"(w1442) -> ()
            n700 = local write "Rec: Temp"(w1405) -> ()
            n701 = Equal To 0?(x=w1405) -> (x = 0?=w1407:bool)
            n702 = case shown="False" w1407 {
              tunnel: [w1521 w1522] -> w1406
              tunnel: w1405 -> [w1521 _]
              frame False {
              }
              frame True {
                n703 = local read "Room Temp"() -> (w1522:dbl)
              }
            }
            n704 = local read "NumPoints Log"() -> (w1430:dbl)
            n705 = local write "Transfer File"(w1408) -> ()
            n706 = local read "Num Pts"() -> (w1433:dbl)
            n707 = local read "New: Dielectric"() -> (w1414:dbl)
            n708 = call "Mobility-Vt Calculator-File.vi"("NumPts"=w1433, "Path"=w1408) -> ("Graph Cluster"=w1402:T9, "Output"=w1432:T10, "Index-Sat"=w1431:dbl, "Index-Lin"=w1418:dbl)  [unwired: 5 in, 1 out]
            n709 = call "STS Calculator-File.vi"("NumPts"=w1430, "Path"=w1408) -> ("STS Index-Sat"=w1429:dbl, "XY Graph-Sat"=w1428:cluster{dbl[], dbl[]}[], "Ouput"=w1427:cluster{"STS-Sat":dbl, "STS-Lin":dbl})  [unwired: 5 in, 2 out]
            n710 = call-poly <vilib>:"Read From Spreadsheet File.vi"("file path (dialog if empty)"=w1408) -> ("all rows"=w1510:string[][])  [unwired: 6 in, 4 out]
            n711 = Unbundle By Name(w1432) -> ("Mobility-Sat"=w1417:dbl, "Vt-Sat"=w1410:dbl, "Mobility-Lin"=w1416:dbl, "Vt-Lin"=w1415:dbl, "Off I-Sat"=w1409:dbl, "On/Off I-Sat"=w1403:dbl)
            n712 = local write "Sat-Trans Slider"(w1431) -> ()
            n713 = Unbundle By Name(w1427) -> ("STS-Sat"=w1411:dbl)  [unwired: 1 out]
            n714 = local write "Index 2"(w1429) -> ()
            n715 = local write "MobVi Index"(w1431) -> ()
            n716 = local write "Log-Sat"(w1428) -> ()
            n717 = local write "Calc: Mobility-Sat"(w1417) -> ()
            n718 = local write "Calc: VT-Sat"(w1410) -> ()
            n719 = local write "Calc: Mobility-Lin"(w1416) -> ()
            n720 = local write "Calc: Off I-Sat"(w1409) -> ()
            n721 = local write "Calc: On/Off"(w1403) -> ()
            n722 = Array Size(array=w1510) -> (size(s)=w1509:i32[])
            n723 = local write "Calc: VT-Lin"(w1415) -> ()
            n724 = call "Trap Density_VT.vi"("VT"=w1410, "Dielectric"=w1414) -> ("Trap Density-VT"=w1413:dbl)
            n725 = call "Trap Density_STS.vi"("Temp (T) [K]"=w1406, "S.T.S. (S)"=w1411, "Dielectric"=w1414) -> ("Trap Density (N)"=w1412:dbl)  [unwired: 8 in]
            n726 = Unbundle By Name(w1402) -> ("Raw Sat"=w1399:cluster{dbl[], dbl[]}[], "Sqrt Sat"=w1400:cluster{dbl[], dbl[]}[], "Log Sat"=w1398:cluster{dbl[], dbl[]}[], "Raw Lin"=w1397:cluster{dbl[], dbl[]}[], "Sqrt Lin"=w1401:cluster{dbl[], dbl[]}[], "Log Lin"=w1396:cluster{dbl[], dbl[]}[])
            n727 = local write "Sqrt-Sat"(w1400) -> ()
            n728 = local write "Calc: STS"(w1411) -> ()
            n729 = local write "New: STS"(w1411) -> ()
            n730 = Decimate 1D Array(w1401) -> (w1426:cluster{dbl[], dbl[]}[])  [unwired: 1 out]
            n731 = local write "Calc: Trap Density-VT"(w1413) -> ()
            n732 = local write "New: VT-Sat"(w1410) -> ()
            n733 = local write "Calc: Trap Density-STS"(w1412) -> ()
            n734 = local write "New: Trap Density-STS"(w1412) -> ()
            n735 = local write "New: Trap Density-VT"(w1413) -> ()
            n736 = local write "New: VT-Lin"(w1415) -> ()
            n737 = local write "Sqrt-Lin"(w1401) -> ()
            n738 = local write "New: Mobility-Sat"(w1417) -> ()
            n739 = local write "New: Mobility-Lin"(w1416) -> ()
            n740 = Decimate 1D Array(w1428) -> (w1487:cluster{dbl[], dbl[]}[])  [unwired: 1 out]
            n741 = Index Array(array=w1509, index=w1508) -> (element=w1493:i32)
            n742 = Decimate 1D Array(w1400) -> (w1497:cluster{dbl[], dbl[]}[])  [unwired: 1 out]
            n743 = Array To Cluster(array=w1426) -> (cluster=w1425:T11)
            n744 = Array Subset(array=w1510, index (row)=w1508, index (col)=w1508, length (col)=3) -> (w1511:string[][])  [unwired: 1 in]
            n745 = local write "Raw- Sat"(w1399) -> ()
            n746 = local write "Raw- Lin"(w1397) -> ()
            n747 = local write "Log-Sat"(w1398) -> ()
            n748 = local write "Log-Lin"(w1396) -> ()
            n749 = Array To Cluster(array=w1487) -> (cluster=w1485:T11)
            n750 = Array To Cluster(array=w1497) -> (cluster=w1499:T11)
            n751 = Reshape Array(w1511, w1493) -> (w1500:string[])
            n752 = Subtract(x=w1493, y=20) -> (x-y=w1492:i32)
            n753 = Unbundle(w1425) -> ("[0]"=w1422:cluster{dbl[], dbl[]})  [unwired: 8 out]
            n754 = property on="Sat-Trans Slider" class="Slide (strict)"("Scale.Maximum"=w1492) -> ()  [unwired: 2 in, 2 out]
            n755 = local read "Num Pts"() -> (w1419:dbl)
            n756 = Unbundle(w1485) -> ("[0]"=w1486:cluster{dbl[], dbl[]})  [unwired: 8 out]
            n757 = Unbundle(w1499) -> ("[0]"=w1498:cluster{dbl[], dbl[]})  [unwired: 8 out]
            n758 = Unbundle(w1422) -> (w1421:dbl[], w1420:dbl[])
            n759 = Search 1D Array(1D array=w1500, element="Index:") -> (index of element=w1505:i32)  [unwired: 1 in]
            n760 = Increment(x=w1505) -> (x+1=w1506:i32)
            n761 = Unbundle(w1486) -> (w1484:dbl[], w1483:dbl[])
            n762 = Unbundle(w1498) -> (w1491:dbl[], w1490:dbl[])
            n763 = Array Subset(array=w1421, index=w1418, length=w1419) -> (w1423:dbl[])
            n764 = Array Subset(array=w1420, index=w1418, length=w1419) -> (w1424:dbl[])
            n765 = local read "Image Folder"() -> (w1459:path)
            n766 = local write "Lin-Vg Array-Used"(w1423) -> ()
            n767 = Array Subset(array=w1484, index=w1429, length=w1430) -> (w1489:dbl[])
            n768 = Array Subset(array=w1483, index=w1429, length=w1430) -> (w1488:dbl[])
            n769 = Array Subset(array=w1491, index=w1431, length=w1433) -> (w1496:dbl[])
            n770 = Array Subset(array=w1490, index=w1431, length=w1433) -> (w1495:dbl[])
            n771 = local write "Lin Id-Used"(w1424) -> ()
            n772 = Index Array(array=w1500, index=w1506) -> (element=w1466:string)
            n773 = local write "Sat Vg Array-Used"(w1496) -> ()
            n774 = local write "Vg Array-Log-Used"(w1488) -> ()
            n775 = local write "Sat Id-Log-Used"(w1489) -> ()
            n776 = local write "Sat Id-Used"(w1495) -> ()
            n777 = local write "Index"(w1466) -> ()
            n778 = List Folder(path=w1459, error in=w1470) -> (filenames=w1502:string[], error out=w1469:errorcluster)  [unwired: 2 in, 2 out]
            n779 = Build Path(base path=w1459, name or relative path="ROI") -> (appended path=w1467:path)
            n780 = invoke on="Image Out" class="ImageControl" method="Clear ROI"(error in=w1469) -> (error out=w1473:errorcluster)  [unwired: 2 in, 2 out]
            n781 = while {
              tunnel: w1502 -> [w1535]
              tunnel: w1466 -> [w1533]
              tunnel: [w1532] -> w1501
              tunnel: w1493 -> [w1531]
              i -> [w1532]
              stop <- w1528 stop-if-true
              n782 = Index Array(array=w1535, index=w1532) -> (element=w1536:string)
              n783 = xnode "Match Regular Expression"("input string"=w1536, "regular expression"=w1533) -> ("whole match"=w1534:string)  [unwired: 4 in, 4 out]
              n784 = Equal?(x=w1534, y=w1533) -> (x = y?=w1530:bool)
              n785 = Equal?(x=w1531, y=w1532) -> (x = y?=w1529:bool)
              n786 = Or(x=w1530, y=w1529) -> (x .or. y?=w1528:bool)
            }
            n787 = Build Path(base path=w1467, name or relative path=w1466) -> (appended path=w1465:path)
            n788 = call <vilib>:"Check if File or Folder Exists.vi"("error in (no error)"=w1473, "path"=w1465) -> ("file or folder exists?"=w1471:bool, "dup path"=w1472:path)  [unwired: 7 in, 1 out]
            n789 = case shown="True" w1471 {
              tunnel: w1472 -> [_ w1523]
              frame False {
              }
              frame True {
                n790 = Read from Text File(file (use dialog)=w1523) -> (text=w1527:string)  [unwired: 3 in, 3 out]
                n791 = property on="Image Out" class="ImageControl"() -> ("ROI"=w1524:T12)  [unwired: 2 in, 2 out]
                n792 = Unflatten From String(type=w1524, binary string=w1527) -> (value=w1525:T12, error out=w1526:errorcluster)  [unwired: 3 in, 1 out]
                n793 = property on="Image Out" class="ImageControl"(error in=w1526, "ROI"=w1525) -> ()  [unwired: 1 in, 2 out]
              }
            }
            n794 = Index Array(array=w1502, index=w1501) -> (element=w1475:string)
            n795 = local write "Image Name"(w1475) -> ()
            n796 = Empty String/Path?(string/path=w1475) -> (empty?=w1482:bool)
            n797 = Build Path(base path=w1459, name or relative path=w1475) -> (appended path=w1474:path)
            n798 = local read "No Image File"() -> (w1481:path)
            n799 = Select(t=w1481, s=w1482, f=w1474) -> (s? t:f=w1476:path)
            n800 = call <vilib>:"Get File Extension.vi"("file"=w1476) -> ("lowercase file extension"=w1478:string)  [unwired: 7 in, 3 out]
            n801 = local write "Image File"(w1476) -> ()
            n802 = local write "String"(w1478) -> ()
            n803 = Search 1D Array(1D array=string[] ["bmp", "jpeg", "png", "jpg", "gif"], element=w1478) -> (index of element=w1477:i32)  [unwired: 1 in]
            n804 = call "Vision Acquisition5"("Image Path"=w1476) -> ("Image Out"=w1480:T2)  [unwired: 25 in, 1 out]
            n805 = Less Than 0?(x=w1477) -> ()  [unwired: 1 out]
            n806 = local write "Image Out"(w1480) -> ()
            n807 = local write "Image Out 2"(w1480) -> ()
          }
          event "Save Changes? 3": Mouse Down {
            n808 = event-data() -> ()  [unwired: 1 in, 7 out]
            n809 = local read "Image Folder"() -> (w1652:path)
            n810 = Build Path(base path=w1652, name or relative path="ROI") -> (appended path=w1659:path)
            n811 = call <vilib>:"Check if File or Folder Exists.vi"("path"=w1659) -> ("file or folder exists?"=w1661:bool, "dup path"=w1658:path)  [unwired: 8 in, 1 out]
            n812 = case shown="False" w1661 {
              tunnel: w1658 -> [w1663 w1664]
              tunnel: [w1662 w1664] -> w1653
              frame False {
                n813 = Create Folder(path (use dialog)=w1663) -> (created path=w1662:path)  [unwired: 2 in, 2 out]
              }
              frame True {
              }
            }
            n814 = local read "Index"() -> (w1655:string)
            n815 = property on="Image Out" class="ImageControl"() -> ("ROI"=w1657:T12)  [unwired: 2 in, 2 out]
            n816 = Build Path(base path=w1653, name or relative path=w1655) -> (appended path=w1654:path)
            n817 = Flatten To String(anything=w1657) -> (data string=w1656:string)  [unwired: 3 in, 2 out]
            n818 = Write to Text File(file (use dialog)=w1654, text=w1656) -> ()  [unwired: 2 in, 3 out]
          }
          event "Next Sqrt Sat": Mouse Down {
            n819 = event-data() -> ()  [unwired: 1 in, 5 out]
            n820 = local read "Sqrt-Sat"() -> (w1677:cluster{dbl[], dbl[]}[])
            n821 = Decimate 1D Array(w1677) -> (w1673:cluster{dbl[], dbl[]}[], w1672:cluster{dbl[], dbl[]}[])
            n822 = Array To Cluster(array=w1673) -> (cluster=w1683:T11)
            n823 = local read "MobVi Index"() -> (w1679:dbl)
            n824 = Unbundle(w1683) -> ("[0]"=w1682:cluster{dbl[], dbl[]})  [unwired: 8 out]
            n825 = local read "Num Pts"() -> (w1678:dbl)
            n826 = Unbundle(w1682) -> (w1681:dbl[], w1680:dbl[])
            n827 = Increment(x=w1679) -> (x+1=w1674:dbl)
            n828 = local read "New: Dielectric"() -> (w1668:dbl)
            n829 = local read "New: Length"() -> (w1667:dbl)
            n830 = local read "New: Width"() -> (w1666:dbl)
            n831 = local write "MobVi Index"(w1674) -> ()
            n832 = Array Subset(array=w1681, index=w1674, length=w1678) -> (w1670:dbl[])
            n833 = Array Subset(array=w1680, index=w1674, length=w1678) -> (w1669:dbl[])
            n834 = local write "Sat Vg Array-Used"(w1670) -> ()
            n835 = local write "Sat Id-Used"(w1669) -> ()
            n836 = call "Mobility-Vt-Used Pts_Saturation.vi"("Width"=w1666, "Length"=w1667, "Dielectric (d)"=w1668, "Sat Id Used"=w1669, "Vg Used"=w1670) -> ("Vt"=w1665:dbl, "Mobility"=w1671:dbl)  [unwired: 4 in, 1 out]
            n837 = Bundle(w1670, w1669) -> (w1676:cluster{dbl[], dbl[]})  [unwired: 1 in]
            n838 = Build Array (concatenate)(w1673, w1672, w1676) -> (w1675:cluster{dbl[], dbl[]}[])
            n839 = local write "New: Mobility-Sat"(w1671) -> ()
            n840 = local write "New: VT-Sat"(w1665) -> ()
            n841 = local write "Sqrt-Sat"(w1675) -> ()
          }
          event "Next Log Sat": Mouse Down {
            n842 = event-data() -> ()  [unwired: 1 in, 7 out]
            n843 = local read "Log-Sat"() -> (w1692:cluster{dbl[], dbl[]}[])
            n844 = Decimate 1D Array(w1692) -> (w1688:cluster{dbl[], dbl[]}[], w1687:cluster{dbl[], dbl[]}[])
            n845 = Array To Cluster(array=w1688) -> (cluster=w1698:T11)
            n846 = local read "Index 2"() -> (w1694:dbl)
            n847 = local read "NumPoints Log"() -> (w1693:dbl)
            n848 = Unbundle(w1698) -> ("[0]"=w1697:cluster{dbl[], dbl[]})  [unwired: 8 out]
            n849 = Unbundle(w1697) -> (w1696:dbl[], w1695:dbl[])
            n850 = Increment(x=w1694) -> (x+1=w1689:dbl)
            n851 = local write "Index 2"(w1689) -> ()
            n852 = Array Subset(array=w1695, index=w1689, length=w1693) -> (w1684:dbl[])
            n853 = Array Subset(array=w1696, index=w1689, length=w1693) -> (w1685:dbl[])
            n854 = call "STS-Used.vi"("Id Used"=w1685, "Vg-Used"=w1684) -> ("STS"=w1686:dbl)  [unwired: 9 in]
            n855 = Bundle(w1685, w1684) -> (w1691:cluster{dbl[], dbl[]})  [unwired: 1 in]
            n856 = local write "Vg Array-Log-Used"(w1684) -> ()
            n857 = local write "Sat Id-Log-Used"(w1685) -> ()
            n858 = local write "New: STS"(w1686) -> ()
            n859 = Build Array (concatenate)(w1688, w1687, w1691) -> (w1690:cluster{dbl[], dbl[]}[])
            n860 = local write "Log-Sat"(w1690) -> ()
          }
          event "Previous Log Sat": Mouse Down {
            n861 = event-data() -> ()  [unwired: 1 in, 7 out]
            n862 = local read "Log-Sat"() -> (w1708:cluster{dbl[], dbl[]}[])
            n863 = Decimate 1D Array(w1708) -> (w1705:cluster{dbl[], dbl[]}[], w1704:cluster{dbl[], dbl[]}[])
            n864 = Array To Cluster(array=w1705) -> (cluster=w1713:T11)
            n865 = local read "Index 2"() -> (w1701:dbl)
            n866 = local read "NumPoints Log"() -> (w1709:dbl)
            n867 = Unbundle(w1713) -> ("[0]"=w1712:cluster{dbl[], dbl[]})  [unwired: 8 out]
            n868 = Unbundle(w1712) -> (w1711:dbl[], w1710:dbl[])
            n869 = Decrement(x=w1701) -> (x-1=w1702:dbl)
            n870 = local write "Index 2"(w1702) -> ()
            n871 = Array Subset(array=w1711, index=w1702, length=w1709) -> (w1699:dbl[])
            n872 = Array Subset(array=w1710, index=w1702, length=w1709) -> (w1700:dbl[])
            n873 = local write "Vg Array-Log-Used"(w1700) -> ()
            n874 = local write "Sat Id-Log-Used"(w1699) -> ()
            n875 = Bundle(w1699, w1700) -> (w1707:cluster{dbl[], dbl[]})  [unwired: 1 in]
            n876 = call "STS-Used.vi"("Id Used"=w1699, "Vg-Used"=w1700) -> ("STS"=w1703:dbl)  [unwired: 9 in]
            n877 = Build Array (concatenate)(w1705, w1704, w1707) -> (w1706:cluster{dbl[], dbl[]}[])
            n878 = local write "New: STS"(w1703) -> ()
            n879 = local write "Log-Sat"(w1706) -> ()
          }
          event "Previous Sqrt Sat": Mouse Down {
            n880 = event-data() -> ()  [unwired: 1 in, 5 out]
            n881 = local read "Sqrt-Sat"() -> (w1727:cluster{dbl[], dbl[]}[])
            n882 = Decimate 1D Array(w1727) -> (w1724:cluster{dbl[], dbl[]}[], w1723:cluster{dbl[], dbl[]}[])
            n883 = Array To Cluster(array=w1724) -> (cluster=w1732:T11)
            n884 = local read "MobVi Index"() -> (w1722:dbl)
            n885 = Unbundle(w1732) -> ("[0]"=w1731:cluster{dbl[], dbl[]})  [unwired: 8 out]
            n886 = local read "Num Pts"() -> (w1728:dbl)
            n887 = Unbundle(w1731) -> (w1730:dbl[], w1729:dbl[])
            n888 = Decrement(x=w1722) -> (x-1=w1721:dbl)
            n889 = local read "New: Dielectric"() -> (w1715:dbl)
            n890 = local read "New: Length"() -> (w1716:dbl)
            n891 = local read "New: Width"() -> (w1717:dbl)
            n892 = local write "MobVi Index"(w1721) -> ()
            n893 = Array Subset(array=w1730, index=w1721, length=w1728) -> (w1720:dbl[])
            n894 = Array Subset(array=w1729, index=w1721, length=w1728) -> (w1719:dbl[])
            n895 = local write "Sat Vg Array-Used"(w1720) -> ()
            n896 = local write "Sat Id-Used"(w1719) -> ()
            n897 = call "Mobility-Vt-Used Pts_Linear.vi"("Width"=w1717, "Length"=w1716, "Dielectric (d)"=w1715, "Sat Id Used"=w1719, "Vg Used"=w1720) -> ("Vt"=w1714:dbl, "Mobility"=w1718:dbl)  [unwired: 4 in, 1 out]
            n898 = Bundle(w1720, w1719) -> (w1726:cluster{dbl[], dbl[]})  [unwired: 1 in]
            n899 = local write "New: VT-Sat"(w1714) -> ()
            n900 = Build Array (concatenate)(w1724, w1723, w1726) -> (w1725:cluster{dbl[], dbl[]}[])
            n901 = local write "New: Mobility-Sat"(w1718) -> ()
            n902 = local write "Sqrt-Sat"(w1725) -> ()
          }
          event "Sat-Trans Slider": Value Change {
            n903 = event-data() -> ()  [unwired: 1 in, 5 out]
            n904 = local read "Sqrt-Sat"() -> (w1745:cluster{dbl[], dbl[]}[])
            n905 = Decimate 1D Array(w1745) -> (w1742:cluster{dbl[], dbl[]}[], w1741:cluster{dbl[], dbl[]}[])
            n906 = Array To Cluster(array=w1742) -> (cluster=w1750:T11)
            n907 = Unbundle(w1750) -> ("[0]"=w1749:cluster{dbl[], dbl[]})  [unwired: 8 out]
            n908 = local read "Sat-Trans Slider"() -> (w1734:dbl)
            n909 = local read "Num Pts"() -> (w1746:dbl)
            n910 = Unbundle(w1749) -> (w1748:dbl[], w1747:dbl[])
            n911 = local read "New: Dielectric"() -> (w1735:dbl)
            n912 = local read "New: Length"() -> (w1736:dbl)
            n913 = local read "New: Width"() -> (w1737:dbl)
            n914 = local write "MobVi Index"(w1734) -> ()
            n915 = Array Subset(array=w1748, index=w1734, length=w1746) -> (w1740:dbl[])
            n916 = Array Subset(array=w1747, index=w1734, length=w1746) -> (w1739:dbl[])
            n917 = local write "Sat Vg Array-Used"(w1740) -> ()
            n918 = local write "Sat Id-Used"(w1739) -> ()
            n919 = call "Mobility-Vt-Used Pts_Linear.vi"("Width"=w1737, "Length"=w1736, "Dielectric (d)"=w1735, "Sat Id Used"=w1739, "Vg Used"=w1740) -> ("Vt"=w1733:dbl, "Mobility"=w1738:dbl)  [unwired: 4 in, 1 out]
            n920 = Bundle(w1740, w1739) -> (w1744:cluster{dbl[], dbl[]})  [unwired: 1 in]
            n921 = local write "New: VT-Sat"(w1733) -> ()
            n922 = Build Array (concatenate)(w1742, w1741, w1744) -> (w1743:cluster{dbl[], dbl[]}[])
            n923 = local write "New: Mobility-Sat"(w1738) -> ()
            n924 = local write "Sqrt-Sat"(w1743) -> ()
          }
          event "Sat-Log Slider": Value Change {
            n925 = event-data() -> ()  [unwired: 1 in, 5 out]
            n926 = local read "Log-Sat"() -> (w1759:cluster{dbl[], dbl[]}[])
            n927 = Decimate 1D Array(w1759) -> (w1756:cluster{dbl[], dbl[]}[], w1755:cluster{dbl[], dbl[]}[])
            n928 = Array To Cluster(array=w1756) -> (cluster=w1764:T11)
            n929 = Unbundle(w1764) -> ("[0]"=w1763:cluster{dbl[], dbl[]})  [unwired: 8 out]
            n930 = local read "NumPoints Log"() -> (w1760:dbl)
            n931 = local read "Sat-Log Slider"() -> (w1754:dbl)
            n932 = Unbundle(w1763) -> (w1762:dbl[], w1761:dbl[])
            n933 = local write "Index 2"(w1754) -> ()
            n934 = Array Subset(array=w1762, index=w1754, length=w1760) -> (w1752:dbl[])
            n935 = Array Subset(array=w1761, index=w1754, length=w1760) -> (w1751:dbl[])
            n936 = local write "Vg Array-Log-Used"(w1751) -> ()
            n937 = local write "Sat Id-Log-Used"(w1752) -> ()
            n938 = call "STS-Used.vi"("Id Used"=w1752, "Vg-Used"=w1751) -> ("STS"=w1753:dbl)  [unwired: 9 in]
            n939 = Bundle(w1752, w1751) -> (w1758:cluster{dbl[], dbl[]})  [unwired: 1 in]
            n940 = local write "New: STS"(w1753) -> ()
            n941 = Build Array (concatenate)(w1756, w1755, w1758) -> (w1757:cluster{dbl[], dbl[]}[])
            n942 = local write "Log-Sat"(w1757) -> ()
          }
          event "Save Changes?": Mouse Down {
            n943 = event-data() -> ()  [unwired: 1 in, 5 out]
            n944 = flat-sequence {
              tunnel: [w1771] -> w1769
              tunnel: [w1779] -> w1768
              tunnel: [w1772] -> w1767
              tunnel: w1769 -> [w2311]
              tunnel: w1768 -> [w2308]
              tunnel: [w2309] -> w1766
              tunnel: w1767 -> [w2309]
              tunnel: [w2308] -> w1765
              tunnel: w1766 -> [w2316]
              tunnel: w1765 -> [w2315]
              frame #0 {
                n945 = Wait (ms)(milliseconds to wait=1) -> ()  [unwired: 1 out]
              }
              frame #1 {
                n946 = local read "Transfer File"() -> (w1771:path)
                n947 = local read "New: Temp"() -> (w1773:dbl)
                n948 = local read "New: Length"() -> (w1777:dbl)
                n949 = local read "New: Width"() -> (w1775:dbl)
                n950 = To Single Precision Float(number=w1773) -> (single precision float=w1774:sgl)
                n951 = Number To Decimal String(number=w1774) -> (decimal integer string=w1782:string)  [unwired: 1 in]
                n952 = To Single Precision Float(number=w1775) -> (single precision float=w1776:sgl)
                n953 = To Single Precision Float(number=w1777) -> (single precision float=w1778:sgl)
                n954 = local read "Index"() -> (w1787:string)
                n955 = Strip Path(path=w1771) -> (stripped path=w1792:path)  [unwired: 1 out]
                n956 = Number To Decimal String(number=w1778) -> (decimal integer string=w1785:string)  [unwired: 1 in]
                n957 = Number To Decimal String(number=w1776) -> (decimal integer string=w1786:string)  [unwired: 1 in]
                n958 = Concatenate Strings("_", w1782, "K") -> (w1780:string)
                n959 = call "Build Text"("Temp"=w1780, "Index"=w1787, "Length"=w1785, "Width"=w1786) -> ("Result"=w1788:string)  [unwired: 10 in, 1 out]
                n960 = flat-sequence {
                  tunnel: [w2265] -> w1784
                  tunnel: w1784 -> [w2282]
                  frame #0 {
                    # "Makes Empty File for Transformer Data"
                    n961 = local read "Transfer Folder"() -> (w2254:path)
                    n962 = Build Path(base path=w2254, name or relative path="Stats") -> (appended path=w2256:path)
                    n963 = call <vilib>:"Check if File or Folder Exists.vi"("path"=w2256) -> ("file or folder exists?"=w2257:bool, "dup path"=w2258:path)  [unwired: 8 in, 1 out]
                    n964 = case shown="False" w2257 {
                      tunnel: [w2262 w2264] -> w2259
                      tunnel: w2258 -> [w2263 w2264]
                      frame False {
                        n965 = Create Folder(path (use dialog)=w2263) -> (created path=w2262:path)  [unwired: 2 in, 2 out]
                      }
                      frame True {
                      }
                    }
                    n966 = Build Path(base path=w2259, name or relative path="Tranformer Data.txt") -> (appended path=w2261:path)
                    n967 = call-poly <vilib>:"Write To Spreadsheet File.vi"("append to file? (new file:F)"=TRUE, "file path (dialog if empty)"=w2261) -> ()  [unwired: 6 in, 1 out]
                  }
                  frame #1 {
                    # "Adds Headers if they don't exist"
                    n968 = local read "Transfer Folder"() -> (w2271:path)
                    n969 = Concatenate Strings("Stats\\", "Tranformer Data.txt") -> (w2272:string)
                    n970 = Build Path(base path=w2271, name or relative path=w2272) -> (appended path=w2265:path)
                    n971 = call-poly <vilib>:"Read From Spreadsheet File.vi"("file path (dialog if empty)"=w2265) -> ("first row"=w2270:string[])  [unwired: 6 in, 4 out]
                    n972 = Search 1D Array(1D array=w2270, element="DeviceID") -> (index of element=w2268:i32)  [unwired: 1 in]
                    n973 = Equal?(x=w2268, y=0) -> (x = y?=w2266:bool)
                    n974 = case shown="False" w2266 {
                      tunnel: w2265 -> [w2276 _]
                      frame False {
                        n975 = local read "Transformer \nHeaders"() -> (w2275:string[])
                        n976 = call-poly <vilib>:"Write To Spreadsheet File.vi"("1D data"=w2275, "file path (dialog if empty)"=w2276) -> ()  [unwired: 6 in, 1 out]
                      }
                      frame True {
                      }
                    }
                  }
                  frame #2 {
                    # "Adds current device if it doesn't exist"
                    n977 = local read "Current \nRecord"() -> (w2281:string[])
                    n978 = Index Array(array=w2281, index=0) -> (element=w2280:string)
                    n979 = local read "Transfer Folder"() -> (w2284:path)
                    n980 = Concatenate Strings("Stats\\", "Tranformer Data.txt") -> (w2285:string)
                    n981 = local write "Current Device ID"(w2280) -> ()
                    n982 = local read "Current Device ID"() -> (w2290:string)
                    n983 = Build Path(base path=w2284, name or relative path=w2285) -> (appended path=w2283:path)
                    n984 = call-poly <vilib>:"Read From Spreadsheet File.vi"("file path (dialog if empty)"=w2283) -> ("all rows"=w2277:string[][])  [unwired: 6 in, 4 out]
                    n985 = Index Array(array=w2277, index (col)=0) -> (element=w2278:string[])  [unwired: 1 in]
                    n986 = Search 1D Array(1D array=w2278, element=w2290) -> (index of element=w2279:i32)  [unwired: 1 in]
                    n987 = Equal?(x=w2279, y=-1) -> (x = y?=w2292:bool)
                    n988 = case shown="False" w2292 {
                      tunnel: w2282 -> [w2295 w2306]
                      tunnel: w2279 -> [w2298 _]
                      tunnel: w2277 -> [w2299 _]
                      frame False {
                        n989 = local read "Current \nRecord"() -> (w2297:string[])
                        n990 = Replace Array Subset(array=w2299, new element=w2297, index (row)=w2298) -> (w2296:string[][])  [unwired: 1 in]
                        n991 = flat-sequence {
                          tunnel: w2295 -> [w2300]
                          tunnel: w2296 -> [w2301]
                          tunnel: [w2301] -> w2294
                          tunnel: [w2300] -> w2293
                          tunnel: w2294 -> [w2303]
                          tunnel: w2293 -> [w2302]
                          frame #0 {
                            n992 = Delete(path (use dialog)=w2300) -> ()  [unwired: 4 in, 3 out]
                          }
                          frame #1 {
                            n993 = call-poly <vilib>:"Write To Spreadsheet File.vi"("append to file? (new file:F)"=TRUE, "2D data"=w2303, "file path (dialog if empty)"=w2302) -> ()  [unwired: 5 in, 1 out]
                          }
                        }
                      }
                      frame True {
                        n994 = local read "Current \nRecord"() -> (w2305:string[])
                        n995 = call-poly <vilib>:"Write To Spreadsheet File.vi"("append to file? (new file:F)"=TRUE, "1D data"=w2305, "file path (dialog if empty)"=w2306) -> ()  [unwired: 5 in, 1 out]
                      }
                    }
                  }
                }
                n996 = Path To String(path=w1792) -> (string=w1790:string)
                n997 = stacked-sequence {
                  tunnel: [_ _ _ _ _ _ _ _ _ _ _ _ _ w2225] -> w1772
                  tunnel: w1771 -> [w1794 _ _ _ _ _ _ _ _ _ _ _ _ _]
                  frame #0 {
                    n998 = call-poly <vilib>:"Read From Spreadsheet File.vi"("file path (dialog if empty)"=w1794) -> ("all rows"=w1793:string[][])  [unwired: 6 in, 4 out]
                    n999 = Array Size(array=w1793) -> (size(s)=w1798:i32[])
                    n1000 = Array Subset(array=w1793, index (row)=0, index (col)=0, length (col)=3) -> (w1802:string[][])  [unwired: 1 in]
                    n1001 = Index Array(array=w1798, index=0) -> (element=w1796:i32)
                    n1002 = Reshape Array(w1802, w1796) -> (w1795:string[])
                    n1003 = Search 1D Array(1D array=w1795, element="Dielectric (nm):") -> (index of element=w1805:i32)  [unwired: 1 in]
                    n1004 = Equal?(x=w1805, y=-1) -> (x = y?=w1804:bool)
                    n1005 = case shown="False" w1804 {
                      tunnel: w1793 -> [w1813 w1817]
                      tunnel: w1805 -> [w1809 _]
                      tunnel: [w1808 w1817] -> w1803
                      frame False {
                        n1006 = local read "New: Dielectric"() -> (w1815:dbl)
                        n1007 = Number To Fractional String(number=w1815) -> (F-format string=w1810:string)  [unwired: 3 in]
                        n1008 = Divide(x=w1809, y=3) -> (x/y=w1812:dbl)
                        n1009 = To Word Integer(number=w1812) -> (16bit integer=w1811:i16)
                        n1010 = Replace Array Subset(array=w1813, new element=w1810, index (row)=w1811, index (col)=1) -> (w1808:string[][])
                      }
                      frame True {
                      }
                    }
                    n1011 = local write "Save1 Array"(w1803) -> ()
                  }
                  frame #1 {
                    n1012 = local read "Save1 Array"() -> (w1819:string[][])
                    n1013 = Array Size(array=w1819) -> (size(s)=w1822:i32[])
                    n1014 = Array Subset(array=w1819, index (row)=0, index (col)=0, length (col)=3) -> (w1826:string[][])  [unwired: 1 in]
                    n1015 = Index Array(array=w1822, index=0) -> (element=w1820:i32)
                    n1016 = Reshape Array(w1826, w1820) -> (w1818:string[])
                    n1017 = Search 1D Array(1D array=w1818, element="Comments:") -> (index of element=w1829:i32)  [unwired: 1 in]
                    n1018 = Equal?(x=w1829, y=-1) -> (x = y?=w1828:bool)
                    n1019 = case shown="False" w1828 {
                      tunnel: w1819 -> [w1837 w1840]
                      tunnel: w1829 -> [w1834 _]
                      tunnel: [w1833 w1840] -> w1827
                      frame False {
                        n1020 = local read "Comments:"() -> (w1832:string)
                        n1021 = Divide(x=w1834, y=3) -> (x/y=w1836:dbl)
                        n1022 = To Word Integer(number=w1836) -> (16bit integer=w1835:i16)
                        n1023 = Replace Array Subset(array=w1837, new element=w1832, index (row)=w1835, index (col)=1) -> (w1833:string[][])
                      }
                      frame True {
                      }
                    }
                    n1024 = local write "Save1 Array"(w1827) -> ()
                  }
                  frame #2 {
                    n1025 = local read "Save1 Array"() -> (w1842:string[][])
                    n1026 = Array Size(array=w1842) -> (size(s)=w1845:i32[])
                    n1027 = Array Subset(array=w1842, index (row)=0, index (col)=0, length (col)=3) -> (w1849:string[][])  [unwired: 1 in]
                    n1028 = Index Array(array=w1845, index=0) -> (element=w1843:i32)
                    n1029 = Reshape Array(w1849, w1843) -> (w1841:string[])
                    n1030 = Search 1D Array(1D array=w1841, element="Length (um):") -> (index of element=w1852:i32)  [unwired: 1 in]
                    n1031 = Equal?(x=w1852, y=-1) -> (x = y?=w1851:bool)
                    n1032 = case shown="False" w1851 {
                      tunnel: w1842 -> [w1862 w1865]
                      tunnel: w1852 -> [w1859 _]
                      tunnel: [w1858 w1865] -> w1850
                      frame False {
                        n1033 = local read "New: Length"() -> (w1855:dbl)
                        n1034 = Divide(x=w1859, y=3) -> (x/y=w1861:dbl)
                        n1035 = Format Value(format string="%#g", value (0)=w1855) -> (output string=w1856:string)  [unwired: 1 in]
                        n1036 = To Word Integer(number=w1861) -> (16bit integer=w1860:i16)
                        n1037 = Replace Array Subset(array=w1862, new element=w1856, index (row)=w1860, index (col)=1) -> (w1858:string[][])
                      }
                      frame True {
                      }
                    }
                    n1038 = local write "Save1 Array"(w1850) -> ()
                  }
                  frame #3 {
                    n1039 = local read "Save1 Array"() -> (w1867:string[][])
                    n1040 = Array Size(array=w1867) -> (size(s)=w1872:i32[])
                    n1041 = Array Subset(array=w1867, index (row)=0, index (col)=0, length (col)=3) -> (w1868:string[][])  [unwired: 1 in]
                    n1042 = Index Array(array=w1872, index=0) -> (element=w1874:i32)
                    n1043 = Reshape Array(w1868, w1874) -> (w1866:string[])
                    n1044 = Search 1D Array(1D array=w1866, element="Width (um):") -> (index of element=w1877:i32)  [unwired: 1 in]
                    n1045 = Equal?(x=w1877, y=-1) -> (x = y?=w1876:bool)
                    n1046 = case shown="False" w1876 {
                      tunnel: w1877 -> [w1885 _]
                      tunnel: w1867 -> [w1884 w1890]
                      tunnel: [w1883 w1890] -> w1875
                      frame False {
                        n1047 = local read "New: Width"() -> (w1880:dbl)
                        n1048 = Divide(x=w1885, y=3) -> (x/y=w1887:dbl)
                        n1049 = To Word Integer(number=w1887) -> (16bit integer=w1886:i16)
                        n1050 = Format Value(format string="%#g", value (0)=w1880) -> (output string=w1881:string)  [unwired: 1 in]
                        n1051 = Replace Array Subset(array=w1884, new element=w1881, index (row)=w1886, index (col)=1) -> (w1883:string[][])
                      }
                      frame True {
                      }
                    }
                    n1052 = local write "Save1 Array"(w1875) -> ()
                  }
                  frame #4 {
                    w1900 = "Sample Temp (K):"
                    n1053 = local read "Save1 Array"() -> (w1892:string[][])
                    n1054 = Array Size(array=w1892) -> (size(s)=w1897:i32[])
                    n1055 = Array Subset(array=w1892, index (row)=0, index (col)=0, length (col)=3) -> (w1893:string[][])  [unwired: 1 in]
                    n1056 = Index Array(array=w1897, index=0) -> (element=w1899:i32)
                    n1057 = Reshape Array(w1893, w1899) -> (w1891:string[])
                    n1058 = Search 1D Array(1D array=w1891, element=w1900) -> (index of element=w1903:i32)  [unwired: 1 in]
                    n1059 = Equal?(x=w1903, y=-1) -> (x = y?=w1902:bool)
                    n1060 = case shown="True" w1902 {
                      tunnel: w1892 -> [w1912 w1926]
                      tunnel: w1903 -> [w1909 _]
                      tunnel: [w1908 w1925] -> w1901
                      tunnel: w1891 -> [_ w1928]
                      tunnel: w1900 -> [_ w1915]
                      frame False {
                        n1061 = local read "New: Temp"() -> (w1906:dbl)
                        n1062 = Divide(x=w1909, y=3) -> (x/y=w1911:dbl)
                        n1063 = Format Value(format string="%#g", value (0)=w1906) -> (output string=w1905:string)  [unwired: 1 in]
                        n1064 = To Word Integer(number=w1911) -> (16bit integer=w1910:i16)
                        n1065 = Replace Array Subset(array=w1912, new element=w1905, index (row)=w1910, index (col)=1) -> (w1908:string[][])
                      }
                      frame True {
                        n1066 = local read "New: Temp"() -> (w1917:dbl)
                        n1067 = Search 1D Array(1D array=w1928, element="Width (um):") -> (index of element=w1922:i32)  [unwired: 1 in]
                        n1068 = Divide(x=w1922, y=3) -> (x/y=w1923:dbl)
                        n1069 = To Word Integer(number=w1923) -> (16bit integer=w1921:i16)
                        n1070 = Format Value(format string="%#g", value (0)=w1917) -> (output string=w1916:string)  [unwired: 1 in]
                        n1071 = Build Array(w1915, w1916) -> (w1919:string[])
                        n1072 = Increment(x=w1921) -> (x+1=w1920:i16)
                        n1073 = Insert Into Array(array=w1926, index (row)=w1920, new element=w1919) -> (w1925:string[][])  [unwired: 1 in]
                      }
                    }
                    n1074 = local write "Save1 Array"(w1901) -> ()
                  }
                  frame #5 {
                    w1938 = "Mobility-Sat (cm^2/Vs):"
                    n1075 = local read "Save1 Array"() -> (w1930:string[][])
                    n1076 = Array Size(array=w1930) -> (size(s)=w1935:i32[])
                    n1077 = Array Subset(array=w1930, index (row)=0, index (col)=0, length (col)=3) -> (w1931:string[][])  [unwired: 1 in]
                    n1078 = Index Array(array=w1935, index=0) -> (element=w1937:i32)
                    n1079 = Reshape Array(w1931, w1937) -> (w1929:string[])
                    n1080 = Search 1D Array(1D array=w1929, element=w1938) -> (index of element=w1941:i32)  [unwired: 1 in]
                    n1081 = Equal?(x=w1941, y=-1) -> (x = y?=w1940:bool)
                    n1082 = case shown="True" w1940 {
                      tunnel: w1930 -> [w1950 w1958]
                      tunnel: w1941 -> [w1947 _]
                      tunnel: [w1946 w1957] -> w1939
                      tunnel: w1929 -> [_ w1955]
                      tunnel: w1938 -> [_ w1953]
                      frame False {
                        n1083 = local read "New: Mobility-Sat"() -> (w1943:dbl)
                        n1084 = Divide(x=w1947, y=3) -> (x/y=w1949:dbl)
                        n1085 = To Word Integer(number=w1949) -> (16bit integer=w1948:i16)
                        n1086 = Format Value(format string="%#g", value (0)=w1943) -> (output string=w1944:string)  [unwired: 1 in]
                        n1087 = Replace Array Subset(array=w1950, new element=w1944, index (row)=w1948, index (col)=1) -> (w1946:string[][])
                      }
                      frame True {
                        n1088 = local read "New: Mobility-Sat"() -> (w1959:dbl)
                        n1089 = Search 1D Array(1D array=w1955, element="Mobility (cm^2/Vs):") -> (index of element=w1962:i32)  [unwired: 1 in]
                        n1090 = Divide(x=w1962, y=3) -> (x/y=w1963:dbl)
                        n1091 = To Word Integer(number=w1963) -> (16bit integer=w1954:i16)
                        n1092 = Format Value(format string="%#g", value (0)=w1959) -> (output string=w1956:string)  [unwired: 1 in]
                        n1093 = Build Array(w1953, w1956) -> (w1961:string[])
                        n1094 = Replace Array Subset(array=w1958, new element=w1961, index (row)=w1954) -> (w1957:string[][])  [unwired: 1 in]
                      }
                    }
                    n1095 = local write "Save1 Array"(w1939) -> ()
                  }
                  frame #6 {
                    w1975 = "Mobility-Lin (cm^2/Vs):"
                    n1096 = local read "Save1 Array"() -> (w1966:string[][])
                    n1097 = Array Size(array=w1966) -> (size(s)=w1972:i32[])
                    n1098 = Array Subset(array=w1966, index (row)=0, index (col)=0, length (col)=3) -> (w1968:string[][])  [unwired: 1 in]
                    n1099 = Index Array(array=w1972, index=0) -> (element=w1974:i32)
                    n1100 = Reshape Array(w1968, w1974) -> (w1967:string[])
                    n1101 = Search 1D Array(1D array=w1967, element=w1975) -> (index of element=w1978:i32)  [unwired: 1 in]
                    n1102 = Equal?(x=w1978, y=-1) -> (x = y?=w1977:bool)
                    n1103 = case shown="True" w1977 {
                      tunnel: w1966 -> [w1987 w1993]
                      tunnel: w1978 -> [w1984 _]
                      tunnel: [w1983 w1992] -> w1976
                      tunnel: w1967 -> [_ w1991]
                      tunnel: w1975 -> [_ w1990]
                      frame False {
                        n1104 = local read "Calc: Mobility-Lin"() -> (w1980:dbl)
                        n1105 = Divide(x=w1984, y=3) -> (x/y=w1986:dbl)
                        n1106 = To Word Integer(number=w1986) -> (16bit integer=w1985:i16)
                        n1107 = Format Value(format string="%#g", value (0)=w1980) -> (output string=w1981:string)  [unwired: 1 in]
                        n1108 = Replace Array Subset(array=w1987, new element=w1981, index (row)=w1985, index (col)=1) -> (w1983:string[][])
                      }
                      frame True {
                        n1109 = local read "Calc: Mobility-Lin"() -> (w1994:dbl)
                        n1110 = Search 1D Array(1D array=w1991, element="Mobility-Sat (cm^2/Vs):") -> (index of element=w1999:i32)  [unwired: 1 in]
                        n1111 = Divide(x=w1999, y=3) -> (x/y=w2000:dbl)
                        n1112 = To Word Integer(number=w2000) -> (16bit integer=w1998:i16)
                        n1113 = Format Value(format string="%#g", value (0)=w1994) -> (output string=w2003:string)  [unwired: 1 in]
                        n1114 = Build Array(w1990, w2003) -> (w1996:string[])
                        n1115 = Increment(x=w1998) -> (x+1=w1997:i16)
                        n1116 = Insert Into Array(array=w1993, index (row)=w1997, new element=w1996) -> (w1992:string[][])  [unwired: 1 in]
                      }
                    }
                    n1117 = local write "Save1 Array"(w1976) -> ()
                  }
                  frame #7 {
                    w2013 = "On/Off I-Sat:"
                    n1118 = local read "Save1 Array"() -> (w2004:string[][])
                    n1119 = Array Size(array=w2004) -> (size(s)=w2010:i32[])
                    n1120 = Array Subset(array=w2004, index (row)=0, index (col)=0, length (col)=3) -> (w2006:string[][])  [unwired: 1 in]
                    n1121 = Index Array(array=w2010, index=0) -> (element=w2012:i32)
                    n1122 = Reshape Array(w2006, w2012) -> (w2005:string[])
                    n1123 = Search 1D Array(1D array=w2005, element=w2013) -> (index of element=w2016:i32)  [unwired: 1 in]
                    n1124 = Equal?(x=w2016, y=-1) -> (x = y?=w2015:bool)
                    n1125 = case shown="True" w2015 {
                      tunnel: w2004 -> [w2025 w2032]
                      tunnel: w2016 -> [w2022 _]
                      tunnel: [w2021 w2033] -> w2014
                      tunnel: w2005 -> [_ w2030]
                      tunnel: w2013 -> [_ w2028]
                      frame False {
                        n1126 = local read "Calc: On/Off"() -> (w2018:dbl)
                        n1127 = Divide(x=w2022, y=3) -> (x/y=w2024:dbl)
                        n1128 = To Word Integer(number=w2024) -> (16bit integer=w2023:i16)
                        n1129 = Format Value(format string="%#g", value (0)=w2018) -> (output string=w2019:string)  [unwired: 1 in]
                        n1130 = Replace Array Subset(array=w2025, new element=w2019, index (row)=w2023, index (col)=1) -> (w2021:string[][])
                      }
                      frame True {
                        n1131 = local read "Calc: On/Off"() -> (w2034:dbl)
                        n1132 = Search 1D Array(1D array=w2030, element="On/Off Current:") -> (index of element=w2037:i32)  [unwired: 1 in]
                        n1133 = Divide(x=w2037, y=3) -> (x/y=w2038:dbl)
                        n1134 = To Word Integer(number=w2038) -> (16bit integer=w2029:i16)
                        n1135 = Format Value(format string="%#g", value (0)=w2034) -> (output string=w2031:string)  [unwired: 1 in]
                        n1136 = Build Array(w2028, w2031) -> (w2036:string[])
                        n1137 = Replace Array Subset(array=w2032, new element=w2036, index (row)=w2029) -> (w2033:string[][])  [unwired: 1 in]
                      }
                    }
                    n1138 = local write "Save1 Array"(w2014) -> ()
                  }
                  frame #8 {
                    w2050 = "Off I-Sat (A):"
                    n1139 = local read "Save1 Array"() -> (w2041:string[][])
                    n1140 = Array Size(array=w2041) -> (size(s)=w2047:i32[])
                    n1141 = Array Subset(array=w2041, index (row)=0, index (col)=0, length (col)=3) -> (w2043:string[][])  [unwired: 1 in]
                    n1142 = Index Array(array=w2047, index=0) -> (element=w2049:i32)
                    n1143 = Reshape Array(w2043, w2049) -> (w2042:string[])
                    n1144 = Search 1D Array(1D array=w2042, element=w2050) -> (index of element=w2053:i32)  [unwired: 1 in]
                    n1145 = Equal?(x=w2053, y=-1) -> (x = y?=w2052:bool)
                    n1146 = case shown="True" w2052 {
                      tunnel: w2041 -> [w2062 w2068]
                      tunnel: w2053 -> [w2059 _]
                      tunnel: [w2058 w2067] -> w2051
                      tunnel: w2042 -> [_ w2066]
                      tunnel: w2050 -> [_ w2065]
                      frame False {
                        n1147 = local read "Calc: Off I-Sat"() -> (w2057:dbl)
                        n1148 = Divide(x=w2059, y=3) -> (x/y=w2061:dbl)
                        n1149 = Format Value(format string="%#g", value (0)=w2057) -> (output string=w2055:string)  [unwired: 1 in]
                        n1150 = To Word Integer(number=w2061) -> (16bit integer=w2060:i16)
                        n1151 = Replace Array Subset(array=w2062, new element=w2055, index (row)=w2060, index (col)=1) -> (w2058:string[][])
                      }
                      frame True {
                        n1152 = local read "Calc: Off I-Sat"() -> (w2069:dbl)
                        n1153 = Search 1D Array(1D array=w2066, element="On/Off I-Sat:") -> (index of element=w2074:i32)  [unwired: 1 in]
                        n1154 = Divide(x=w2074, y=3) -> (x/y=w2075:dbl)
                        n1155 = To Word Integer(number=w2075) -> (16bit integer=w2073:i16)
                        n1156 = Format Value(format string="%#g", value (0)=w2069) -> (output string=w2078:string)  [unwired: 1 in]
                        n1157 = Build Array(w2065, w2078) -> (w2071:string[])
                        n1158 = Increment(x=w2073) -> (x+1=w2072:i16)
                        n1159 = Insert Into Array(array=w2068, index (row)=w2072, new element=w2071) -> (w2067:string[][])  [unwired: 1 in]
                      }
                    }
                    n1160 = local write "Save1 Array"(w2051) -> ()
                  }
                  frame #9 {
                    w2080 = "Vt-Sat (V):"
                    n1161 = local read "Save1 Array"() -> (w2081:string[][])
                    n1162 = Array Size(array=w2081) -> (size(s)=w2086:i32[])
                    n1163 = Array Subset(array=w2081, index (row)=0, index (col)=0, length (col)=3) -> (w2082:string[][])  [unwired: 1 in]
                    n1164 = Index Array(array=w2086, index=0) -> (element=w2088:i32)
                    n1165 = Reshape Array(w2082, w2088) -> (w2079:string[])
                    n1166 = Search 1D Array(1D array=w2079, element=w2080) -> (index of element=w2091:i32)  [unwired: 1 in]
                    n1167 = Equal?(x=w2091, y=-1) -> (x = y?=w2090:bool)
                    n1168 = case shown="True" w2090 {
                      tunnel: w2081 -> [w2098 w2107]
                      tunnel: w2091 -> [w2094 _]
                      tunnel: [w2093 w2106] -> w2089
                      tunnel: w2080 -> [_ w2105]
                      tunnel: w2079 -> [_ w2104]
                      frame False {
                        n1169 = local read "New: VT-Sat"() -> (w2100:dbl)
                        n1170 = Number To Fractional String(number=w2100) -> (F-format string=w2095:string)  [unwired: 3 in]
                        n1171 = Divide(x=w2094, y=3) -> (x/y=w2097:dbl)
                        n1172 = To Word Integer(number=w2097) -> (16bit integer=w2096:i16)
                        n1173 = Replace Array Subset(array=w2098, new element=w2095, index (row)=w2096, index (col)=1) -> (w2093:string[][])
                      }
                      frame True {
                        n1174 = local read "New: VT-Sat"() -> (w2108:dbl)
                        n1175 = Search 1D Array(1D array=w2104, element="Threshold V (V):") -> (index of element=w2103:i32)  [unwired: 1 in]
                        n1176 = Divide(x=w2103, y=3) -> (x/y=w2111:dbl)
                        n1177 = To Word Integer(number=w2111) -> (16bit integer=w2102:i16)
                        n1178 = Format Value(format string="%#g", value (0)=w2108) -> (output string=w2114:string)  [unwired: 1 in]
                        n1179 = Build Array(w2105, w2114) -> (w2110:string[])
                        n1180 = Replace Array Subset(array=w2107, new element=w2110, index (row)=w2102) -> (w2106:string[][])  [unwired: 1 in]
                      }
                    }
                    n1181 = local write "Save1 Array"(w2089) -> ()
                  }
                  frame #10 {
                    n1182 = local read "Save1 Array"() -> (w2115:string[][])
                    n1183 = Array Size(array=w2115) -> (size(s)=w2121:i32[])
                    n1184 = Array Subset(array=w2115, index (row)=0, index (col)=0, length (col)=3) -> (w2117:string[][])  [unwired: 1 in]
                    n1185 = Index Array(array=w2121, index=0) -> (element=w2123:i32)
                    n1186 = Reshape Array(w2117, w2123) -> (w2116:string[])
                    n1187 = Search 1D Array(1D array=w2116, element="VT-Lin (V):") -> (index of element=w2126:i32)  [unwired: 1 in]
                    n1188 = Equal?(x=w2126, y=-1) -> (x = y?=w2125:bool)
                    n1189 = case shown="False" w2125 {
                      tunnel: w2115 -> [w2136 w2139]
                      tunnel: w2126 -> [w2133 _]
                      tunnel: [w2132 w2139] -> w2124
                      frame False {
                        n1190 = local read "New: VT-Lin"() -> (w2130:dbl)
                        n1191 = Divide(x=w2133, y=3) -> (x/y=w2135:dbl)
                        n1192 = Format Value(format string="%#g", value (0)=w2130) -> (output string=w2129:string)  [unwired: 1 in]
                        n1193 = To Word Integer(number=w2135) -> (16bit integer=w2134:i16)
                        n1194 = Replace Array Subset(array=w2136, new element=w2129, index (row)=w2134, index (col)=1) -> (w2132:string[][])
                      }
                      frame True {
                      }
                    }
                    n1195 = local write "Save1 Array"(w2124) -> ()
                  }
                  frame #11 {
                    w2140 = "STS-Sat (V/decade):"
                    n1196 = local read "Save1 Array"() -> (w2142:string[][])
                    n1197 = Array Size(array=w2142) -> (size(s)=w2147:i32[])
                    n1198 = Array Subset(array=w2142, index (row)=0, index (col)=0, length (col)=3) -> (w2143:string[][])  [unwired: 1 in]
                    n1199 = Index Array(array=w2147, index=0) -> (element=w2149:i32)
                    n1200 = Reshape Array(w2143, w2149) -> (w2141:string[])
                    n1201 = Search 1D Array(1D array=w2141, element=w2140) -> (index of element=w2152:i32)  [unwired: 1 in]
                    n1202 = Equal?(x=w2152, y=-1) -> (x = y?=w2151:bool)
                    n1203 = case shown="True" w2151 {
                      tunnel: w2142 -> [w2161 w2167]
                      tunnel: w2152 -> [w2158 _]
                      tunnel: [w2157 w2168] -> w2150
                      tunnel: w2141 -> [_ w2166]
                      tunnel: w2140 -> [_ w2165]
                      frame False {
                        n1204 = local read "New: STS"() -> (w2155:dbl)
                        n1205 = Divide(x=w2158, y=3) -> (x/y=w2160:dbl)
                        n1206 = Format Value(format string="%#g", value (0)=w2155) -> (output string=w2154:string)  [unwired: 1 in]
                        n1207 = To Word Integer(number=w2160) -> (16bit integer=w2159:i16)
                        n1208 = Replace Array Subset(array=w2161, new element=w2154, index (row)=w2159, index (col)=1) -> (w2157:string[][])
                      }
                      frame True {
                        n1209 = local read "New: STS"() -> (w2169:dbl)
                        n1210 = Search 1D Array(1D array=w2166, element="S.T.S. (V/decade):") -> (index of element=w2172:i32)  [unwired: 1 in]
                        n1211 = Divide(x=w2172, y=3) -> (x/y=w2173:dbl)
                        n1212 = To Word Integer(number=w2173) -> (16bit integer=w2164:i16)
                        n1213 = Format Value(format string="%#g", value (0)=w2169) -> (output string=w2176:string)  [unwired: 1 in]
                        n1214 = Build Array(w2165, w2176) -> (w2171:string[])
                        n1215 = Replace Array Subset(array=w2167, new element=w2171, index (row)=w2164) -> (w2168:string[][])  [unwired: 1 in]
                      }
                    }
                    n1216 = local write "Save1 Array"(w2150) -> ()
                  }
                  frame #12 {
                    w2177 = "Trap Density-VT (Traps/Vcm^2):"
                    n1217 = local read "Save1 Array"() -> (w2179:string[][])
                    n1218 = Array Size(array=w2179) -> (size(s)=w2184:i32[])
                    n1219 = Array Subset(array=w2179, index (row)=0, index (col)=0, length (col)=3) -> (w2180:string[][])  [unwired: 1 in]
                    n1220 = Index Array(array=w2184, index=0) -> (element=w2186:i32)
                    n1221 = Reshape Array(w2180, w2186) -> (w2178:string[])
                    n1222 = Search 1D Array(1D array=w2178, element=w2177) -> (index of element=w2189:i32)  [unwired: 1 in]
                    n1223 = Equal?(x=w2189, y=-1) -> (x = y?=w2188:bool)
                    n1224 = case shown="True" w2188 {
                      tunnel: w2179 -> [w2198 w2203]
                      tunnel: w2189 -> [w2194 _]
                      tunnel: [w2193 w2204] -> w2187
                      tunnel: w2178 -> [_ w2202]
                      tunnel: w2177 -> [_ w2201]
                      frame False {
                        n1225 = local read "New: Trap Density-VT"() -> (w2192:dbl)
                        n1226 = Format Value(format string="%#g", value (0)=w2192) -> (output string=w2195:string)  [unwired: 1 in]
                        n1227 = Divide(x=w2194, y=3) -> (x/y=w2197:dbl)
                        n1228 = To Word Integer(number=w2197) -> (16bit integer=w2196:i16)
                        n1229 = Replace Array Subset(array=w2198, new element=w2195, index (row)=w2196, index (col)=1) -> (w2193:string[][])
                      }
                      frame True {
                        n1230 = local read "New: Trap Density-VT"() -> (w2214:dbl)
                        n1231 = Search 1D Array(1D array=w2202, element="STS-Sat (V/decade):") -> (index of element=w2209:i32)  [unwired: 1 in]
                        n1232 = Divide(x=w2209, y=3) -> (x/y=w2208:dbl)
                        n1233 = To Word Integer(number=w2208) -> (16bit integer=w2210:i16)
                        n1234 = Format Value(format string="%#g", value (0)=w2214) -> (output string=w2205:string)  [unwired: 1 in]
                        n1235 = Build Array(w2201, w2205) -> (w2212:string[])
                        n1236 = Increment(x=w2210) -> (x+1=w2211:i16)
                        n1237 = Insert Into Array(array=w2203, index (row)=w2211, new element=w2212) -> (w2204:string[][])  [unwired: 1 in]
                      }
                    }
                    n1238 = local write "Save1 Array"(w2187) -> ()
                  }
                  frame #13 {
                    w2215 = "Trap Density-STS (Traps/Vcm^2):"
                    n1239 = local read "Save1 Array"() -> (w2217:string[][])
                    n1240 = Array Size(array=w2217) -> (size(s)=w2222:i32[])
                    n1241 = Array Subset(array=w2217, index (row)=0, index (col)=0, length (col)=3) -> (w2218:string[][])  [unwired: 1 in]
                    n1242 = Index Array(array=w2222, index=0) -> (element=w2224:i32)
                    n1243 = Reshape Array(w2218, w2224) -> (w2216:string[])
                    n1244 = Search 1D Array(1D array=w2216, element=w2215) -> (index of element=w2227:i32)  [unwired: 1 in]
                    n1245 = Equal?(x=w2227, y=-1) -> (x = y?=w2226:bool)
                    n1246 = case shown="True" w2226 {
                      tunnel: w2217 -> [w2236 w2241]
                      tunnel: w2227 -> [w2233 _]
                      tunnel: [w2232 w2242] -> w2225
                      tunnel: w2216 -> [_ w2240]
                      tunnel: w2215 -> [_ w2239]
                      frame False {
                        n1247 = local read "New: Trap Density-STS"() -> (w2230:dbl)
                        n1248 = Divide(x=w2233, y=3) -> (x/y=w2235:dbl)
                        n1249 = To Word Integer(number=w2235) -> (16bit integer=w2234:i16)
                        n1250 = Format Value(format string="%#g", value (0)=w2230) -> (output string=w2229:string)  [unwired: 1 in]
                        n1251 = Replace Array Subset(array=w2236, new element=w2229, index (row)=w2234, index (col)=1) -> (w2232:string[][])
                      }
                      frame True {
                        n1252 = local read "New: Trap Density-STS"() -> (w2243:dbl)
                        n1253 = Search 1D Array(1D array=w2240, element="Trap Density-VT (Traps/Vcm^2):") -> (index of element=w2248:i32)  [unwired: 1 in]
                        n1254 = Divide(x=w2248, y=3) -> (x/y=w2249:dbl)
                        n1255 = To Word Integer(number=w2249) -> (16bit integer=w2247:i16)
                        n1256 = Format Value(format string="%#g", value (0)=w2243) -> (output string=w2252:string)  [unwired: 1 in]
                        n1257 = Build Array(w2239, w2252) -> (w2245:string[])
                        n1258 = Increment(x=w2247) -> (x+1=w2246:i16)
                        n1259 = Insert Into Array(array=w2241, index (row)=w2246, new element=w2245) -> (w2242:string[][])  [unwired: 1 in]
                      }
                    }
                    n1260 = local write "Save1 Array"(w2225) -> ()
                  }
                }
                n1261 = Concatenate Strings(w1790, "\\", w1788) -> (w1789:string)
                n1262 = String To Path(string=w1789) -> (path=w1779:path)
                n1263 = disable-structure shown="Disabled" {
                  frame Disabled {
                  }
                  frame Enabled {
                  }
                }
              }
              frame #2 {
                n1264 = Equal?(x=w2311, y=w2308) -> (x = y?=w2310:bool)
                n1265 = case shown="False" w2310 {
                  tunnel: w2311 -> [w2314 _]
                  tunnel: w2308 -> [w2313 _]
                  frame False {
                    n1266 = Move(source path=w2314, 9:TRUE, 10:w2313) -> ()  [unwired: 2 in, 3 out]
                  }
                  frame True {
                  }
                }
              }
              frame #3 {
                n1267 = local write "Transfer File"(w2315) -> ()
                n1268 = call-poly <vilib>:"Write To Spreadsheet File.vi"("2D data"=w2316, "file path (dialog if empty)"=w2315) -> ()  [unwired: 6 in, 1 out]
              }
            }
          }
          event "Save Changes? 2": Mouse Down {
            n1269 = event-data() -> ()  [unwired: 1 in, 5 out]
            n1270 = stacked-sequence {
              seq-local: [w2374 _ _ _ _] -> [_ w2857 _ _ _]
              seq-local: [w2373 _ _ _ _] -> [_ w2858 _ _ _]
              seq-local: [w2373 _ _ _ _] -> [_ w2856 _ _ _]
              seq-local: [w2375 _ _ _ _] -> [_ w2854 _ _ _]
              seq-local: [_ w2858 _ _ _] -> [_ _ w2863 _ _]
              seq-local: [_ w2854 _ _ _] -> [_ _ w2862 _ _]
              frame #0 {
                n1271 = local read "Transfer File"() -> (w2374:path)
                n1272 = local read "New: Temp"() -> (w2377:dbl)
                n1273 = local read "New: Length"() -> (w2380:dbl)
                n1274 = local read "New: Width"() -> (w2378:dbl)
                n1275 = To Word Integer(number=w2377) -> (16bit integer=w2376:i16)
                n1276 = Number To Decimal String(number=w2376) -> (decimal integer string=w2384:string)  [unwired: 1 in]
                n1277 = To Single Precision Float(number=w2378) -> (single precision float=w2379:sgl)
                n1278 = To Single Precision Float(number=w2380) -> (single precision float=w2381:sgl)
                n1279 = local read "Index"() -> (w2388:string)
                n1280 = Strip Path(path=w2374) -> (stripped path=w2393:path)  [unwired: 1 out]
                n1281 = Number To Decimal String(number=w2381) -> (decimal integer string=w2386:string)  [unwired: 1 in]
                n1282 = Number To Decimal String(number=w2379) -> (decimal integer string=w2387:string)  [unwired: 1 in]
                n1283 = Concatenate Strings("_", w2384, "K") -> (w2382:string)
                n1284 = call "Build Text2"("Temp"=w2382, "Index"=w2388, "Length"=w2386, "Width"=w2387) -> ("Result"=w2389:string)  [unwired: 10 in, 1 out]
                n1285 = Path To String(path=w2393) -> (string=w2391:string)
                n1286 = Concatenate Strings(w2391, "\\", w2389) -> (w2390:string)
                n1287 = stacked-sequence {
                  tunnel: [_ _ _ _ _ _ _ _ _ _ _ _ _ w2816] -> _
                  tunnel: w2374 -> [w2395 _ _ _ _ _ _ _ _ _ _ _ _ _]
                  tunnel: [_ _ _ _ _ _ _ _ _ _ _ _ _ w2816] -> w2375
                  frame #0 {
                    n1288 = call-poly <vilib>:"Read From Spreadsheet File.vi"("file path (dialog if empty)"=w2395) -> ("all rows"=w2394:string[][])  [unwired: 6 in, 4 out]
                    n1289 = Array Size(array=w2394) -> (size(s)=w2399:i32[])
                    n1290 = Array Subset(array=w2394, index (row)=0, index (col)=0, length (col)=3) -> (w2403:string[][])  [unwired: 1 in]
                    n1291 = Index Array(array=w2399, index=0) -> (element=w2397:i32)
                    n1292 = Reshape Array(w2403, w2397) -> (w2396:string[])
                    n1293 = Search 1D Array(1D array=w2396, element="Dielectric (nm):") -> (index of element=w2406:i32)  [unwired: 1 in]
                    n1294 = Equal?(x=w2406, y=-1) -> (x = y?=w2405:bool)
                    n1295 = case shown="False" w2405 {
                      tunnel: w2394 -> [w2414 w2418]
                      tunnel: w2406 -> [w2410 _]
                      tunnel: [w2409 w2418] -> w2404
                      frame False {
                        n1296 = local read "New: Dielectric"() -> (w2416:dbl)
                        n1297 = Number To Fractional String(number=w2416) -> (F-format string=w2411:string)  [unwired: 3 in]
                        n1298 = Divide(x=w2410, y=3) -> (x/y=w2413:dbl)
                        n1299 = To Word Integer(number=w2413) -> (16bit integer=w2412:i16)
                        n1300 = Replace Array Subset(array=w2414, new element=w2411, index (row)=w2412, index (col)=1) -> (w2409:string[][])
                      }
                      frame True {
                      }
                    }
                    n1301 = local write "Save1 Array"(w2404) -> ()
                  }
                  frame #1 {
                    n1302 = local read "Save1 Array"() -> (w2420:string[][])
                    n1303 = Array Size(array=w2420) -> (size(s)=w2423:i32[])
                    n1304 = Array Subset(array=w2420, index (row)=0, index (col)=0, length (col)=3) -> (w2427:string[][])  [unwired: 1 in]
                    n1305 = Index Array(array=w2423, index=0) -> (element=w2421:i32)
                    n1306 = Reshape Array(w2427, w2421) -> (w2419:string[])
                    n1307 = Search 1D Array(1D array=w2419, element="Comments:") -> (index of element=w2430:i32)  [unwired: 1 in]
                    n1308 = Equal?(x=w2430, y=-1) -> (x = y?=w2429:bool)
                    n1309 = case shown="False" w2429 {
                      tunnel: w2420 -> [w2438 w2441]
                      tunnel: w2430 -> [w2435 _]
                      tunnel: [w2434 w2441] -> w2428
                      frame False {
                        n1310 = local read "Comments:"() -> (w2433:string)
                        n1311 = Divide(x=w2435, y=3) -> (x/y=w2437:dbl)
                        n1312 = To Word Integer(number=w2437) -> (16bit integer=w2436:i16)
                        n1313 = Replace Array Subset(array=w2438, new element=w2433, index (row)=w2436, index (col)=1) -> (w2434:string[][])
                      }
                      frame True {
                      }
                    }
                    n1314 = local write "Save1 Array"(w2428) -> ()
                  }
                  frame #2 {
                    n1315 = local read "Save1 Array"() -> (w2443:string[][])
                    n1316 = Array Size(array=w2443) -> (size(s)=w2446:i32[])
                    n1317 = Array Subset(array=w2443, index (row)=0, index (col)=0, length (col)=3) -> (w2450:string[][])  [unwired: 1 in]
                    n1318 = Index Array(array=w2446, index=0) -> (element=w2444:i32)
                    n1319 = Reshape Array(w2450, w2444) -> (w2442:string[])
                    n1320 = Search 1D Array(1D array=w2442, element="Length (um):") -> (index of element=w2453:i32)  [unwired: 1 in]
                    n1321 = Equal?(x=w2453, y=-1) -> (x = y?=w2452:bool)
                    n1322 = case shown="False" w2452 {
                      tunnel: w2443 -> [w2463 w2466]
                      tunnel: w2453 -> [w2460 _]
                      tunnel: [w2459 w2466] -> w2451
                      frame False {
                        n1323 = local read "New: Length"() -> (w2456:dbl)
                        n1324 = Divide(x=w2460, y=3) -> (x/y=w2462:dbl)
                        n1325 = Format Value(format string="%#g", value (0)=w2456) -> (output string=w2457:string)  [unwired: 1 in]
                        n1326 = To Word Integer(number=w2462) -> (16bit integer=w2461:i16)
                        n1327 = Replace Array Subset(array=w2463, new element=w2457, index (row)=w2461, index (col)=1) -> (w2459:string[][])
                      }
                      frame True {
                      }
                    }
                    n1328 = local write "Save1 Array"(w2451) -> ()
                  }
                  frame #3 {
                    n1329 = local read "Save1 Array"() -> (w2468:string[][])
                    n1330 = Array Size(array=w2468) -> (size(s)=w2473:i32[])
                    n1331 = Array Subset(array=w2468, index (row)=0, index (col)=0, length (col)=3) -> (w2469:string[][])  [unwired: 1 in]
                    n1332 = Index Array(array=w2473, index=0) -> (element=w2475:i32)
                    n1333 = Reshape Array(w2469, w2475) -> (w2467:string[])
                    n1334 = Search 1D Array(1D array=w2467, element="Width (um):") -> (index of element=w2478:i32)  [unwired: 1 in]
                    n1335 = Equal?(x=w2478, y=-1) -> (x = y?=w2477:bool)
                    n1336 = case shown="False" w2477 {
                      tunnel: w2478 -> [w2486 _]
                      tunnel: w2468 -> [w2485 w2491]
                      tunnel: [w2484 w2491] -> w2476
                      frame False {
                        n1337 = local read "New: Width"() -> (w2481:dbl)
                        n1338 = Divide(x=w2486, y=3) -> (x/y=w2488:dbl)
                        n1339 = To Word Integer(number=w2488) -> (16bit integer=w2487:i16)
                        n1340 = Format Value(format string="%#g", value (0)=w2481) -> (output string=w2482:string)  [unwired: 1 in]
                        n1341 = Replace Array Subset(array=w2485, new element=w2482, index (row)=w2487, index (col)=1) -> (w2484:string[][])
                      }
                      frame True {
                      }
                    }
                    n1342 = local write "Save1 Array"(w2476) -> ()
                  }
                  frame #4 {
                    w2501 = "Sample Temp (K):"
                    n1343 = local read "Save1 Array"() -> (w2493:string[][])
                    n1344 = Array Size(array=w2493) -> (size(s)=w2498:i32[])
                    n1345 = Array Subset(array=w2493, index (row)=0, index (col)=0, length (col)=3) -> (w2494:string[][])  [unwired: 1 in]
                    n1346 = Index Array(array=w2498, index=0) -> (element=w2500:i32)
                    n1347 = Reshape Array(w2494, w2500) -> (w2492:string[])
                    n1348 = Search 1D Array(1D array=w2492, element=w2501) -> (index of element=w2504:i32)  [unwired: 1 in]
                    n1349 = Equal?(x=w2504, y=-1) -> (x = y?=w2503:bool)
                    n1350 = case shown="True" w2503 {
                      tunnel: w2493 -> [w2513 w2527]
                      tunnel: w2504 -> [w2510 _]
                      tunnel: [w2509 w2526] -> w2502
                      tunnel: w2492 -> [_ w2529]
                      tunnel: w2501 -> [_ w2516]
                      frame False {
                        n1351 = local read "New: Temp"() -> (w2507:dbl)
                        n1352 = Divide(x=w2510, y=3) -> (x/y=w2512:dbl)
                        n1353 = Format Value(format string="%#g", value (0)=w2507) -> (output string=w2506:string)  [unwired: 1 in]
                        n1354 = To Word Integer(number=w2512) -> (16bit integer=w2511:i16)
                        n1355 = Replace Array Subset(array=w2513, new element=w2506, index (row)=w2511, index (col)=1) -> (w2509:string[][])
                      }
                      frame True {
                        n1356 = local read "New: Temp"() -> (w2518:dbl)
                        n1357 = Search 1D Array(1D array=w2529, element="Width (um):") -> (index of element=w2523:i32)  [unwired: 1 in]
                        n1358 = Divide(x=w2523, y=3) -> (x/y=w2524:dbl)
                        n1359 = To Word Integer(number=w2524) -> (16bit integer=w2522:i16)
                        n1360 = Format Value(format string="%#g", value (0)=w2518) -> (output string=w2517:string)  [unwired: 1 in]
                        n1361 = Build Array(w2516, w2517) -> (w2520:string[])
                        n1362 = Increment(x=w2522) -> (x+1=w2521:i16)
                        n1363 = Insert Into Array(array=w2527, index (row)=w2521, new element=w2520) -> (w2526:string[][])  [unwired: 1 in]
                      }
                    }
                    n1364 = local write "Save1 Array"(w2502) -> ()
                  }
                  frame #5 {
                    w2539 = "Mobility-Sat (cm^2/Vs):"
                    n1365 = local read "Save1 Array"() -> (w2531:string[][])
                    n1366 = Array Size(array=w2531) -> (size(s)=w2536:i32[])
                    n1367 = Array Subset(array=w2531, index (row)=0, index (col)=0, length (col)=3) -> (w2532:string[][])  [unwired: 1 in]
                    n1368 = Index Array(array=w2536, index=0) -> (element=w2538:i32)
                    n1369 = Reshape Array(w2532, w2538) -> (w2530:string[])
                    n1370 = Search 1D Array(1D array=w2530, element=w2539) -> (index of element=w2542:i32)  [unwired: 1 in]
                    n1371 = Equal?(x=w2542, y=-1) -> (x = y?=w2541:bool)
                    n1372 = case shown="True" w2541 {
                      tunnel: w2531 -> [w2551 w2559]
                      tunnel: w2542 -> [w2548 _]
                      tunnel: [w2547 w2558] -> w2540
                      tunnel: w2530 -> [_ w2556]
                      tunnel: w2539 -> [_ w2554]
                      frame False {
                        n1373 = local read "New: Mobility-Sat"() -> (w2544:dbl)
                        n1374 = Divide(x=w2548, y=3) -> (x/y=w2550:dbl)
                        n1375 = To Word Integer(number=w2550) -> (16bit integer=w2549:i16)
                        n1376 = Format Value(format string="%#g", value (0)=w2544) -> (output string=w2545:string)  [unwired: 1 in]
                        n1377 = Replace Array Subset(array=w2551, new element=w2545, index (row)=w2549, index (col)=1) -> (w2547:string[][])
                      }
                      frame True {
                        n1378 = local read "New: Mobility-Sat"() -> (w2560:dbl)
                        n1379 = Search 1D Array(1D array=w2556, element="Mobility (cm^2/Vs):") -> (index of element=w2563:i32)  [unwired: 1 in]
                        n1380 = Divide(x=w2563, y=3) -> (x/y=w2564:dbl)
                        n1381 = To Word Integer(number=w2564) -> (16bit integer=w2555:i16)
                        n1382 = Format Value(format string="%#g", value (0)=w2560) -> (output string=w2557:string)  [unwired: 1 in]
                        n1383 = Build Array(w2554, w2557) -> (w2562:string[])
                        n1384 = Replace Array Subset(array=w2559, new element=w2562, index (row)=w2555) -> (w2558:string[][])  [unwired: 1 in]
                      }
                    }
                    n1385 = local write "Save1 Array"(w2540) -> ()
                  }
                  frame #6 {
                    w2576 = "Mobility-Lin (cm^2/Vs):"
                    n1386 = local read "Save1 Array"() -> (w2567:string[][])
                    n1387 = Array Size(array=w2567) -> (size(s)=w2573:i32[])
                    n1388 = Array Subset(array=w2567, index (row)=0, index (col)=0, length (col)=3) -> (w2569:string[][])  [unwired: 1 in]
                    n1389 = Index Array(array=w2573, index=0) -> (element=w2575:i32)
                    n1390 = Reshape Array(w2569, w2575) -> (w2568:string[])
                    n1391 = Search 1D Array(1D array=w2568, element=w2576) -> (index of element=w2579:i32)  [unwired: 1 in]
                    n1392 = Equal?(x=w2579, y=-1) -> (x = y?=w2578:bool)
                    n1393 = case shown="True" w2578 {
                      tunnel: w2567 -> [w2588 w2594]
                      tunnel: w2579 -> [w2585 _]
                      tunnel: [w2584 w2593] -> w2577
                      tunnel: w2568 -> [_ w2592]
                      tunnel: w2576 -> [_ w2591]
                      frame False {
                        n1394 = local read "Calc: Mobility-Lin"() -> (w2581:dbl)
                        n1395 = Divide(x=w2585, y=3) -> (x/y=w2587:dbl)
                        n1396 = To Word Integer(number=w2587) -> (16bit integer=w2586:i16)
                        n1397 = Format Value(format string="%#g", value (0)=w2581) -> (output string=w2582:string)  [unwired: 1 in]
                        n1398 = Replace Array Subset(array=w2588, new element=w2582, index (row)=w2586, index (col)=1) -> (w2584:string[][])
                      }
                      frame True {
                        n1399 = local read "Calc: Mobility-Lin"() -> (w2595:dbl)
                        n1400 = Search 1D Array(1D array=w2592, element="Mobility-Sat (cm^2/Vs):") -> (index of element=w2600:i32)  [unwired: 1 in]
                        n1401 = Divide(x=w2600, y=3) -> (x/y=w2601:dbl)
                        n1402 = To Word Integer(number=w2601) -> (16bit integer=w2599:i16)
                        n1403 = Format Value(format string="%#g", value (0)=w2595) -> (output string=w2604:string)  [unwired: 1 in]
                        n1404 = Build Array(w2591, w2604) -> (w2597:string[])
                        n1405 = Increment(x=w2599) -> (x+1=w2598:i16)
                        n1406 = Insert Into Array(array=w2594, index (row)=w2598, new element=w2597) -> (w2593:string[][])  [unwired: 1 in]
                      }
                    }
                    n1407 = local write "Save1 Array"(w2577) -> ()
                  }
                  frame #7 {
                    w2614 = "On/Off I-Sat:"
                    n1408 = local read "Save1 Array"() -> (w2605:string[][])
                    n1409 = Array Size(array=w2605) -> (size(s)=w2611:i32[])
                    n1410 = Array Subset(array=w2605, index (row)=0, index (col)=0, length (col)=3) -> (w2607:string[][])  [unwired: 1 in]
                    n1411 = Index Array(array=w2611, index=0) -> (element=w2613:i32)
                    n1412 = Reshape Array(w2607, w2613) -> (w2606:string[])
                    n1413 = Search 1D Array(1D array=w2606, element=w2614) -> (index of element=w2617:i32)  [unwired: 1 in]
                    n1414 = Equal?(x=w2617, y=-1) -> (x = y?=w2616:bool)
                    n1415 = case shown="True" w2616 {
                      tunnel: w2605 -> [w2626 w2633]
                      tunnel: w2617 -> [w2623 _]
                      tunnel: [w2622 w2634] -> w2615
                      tunnel: w2606 -> [_ w2631]
                      tunnel: w2614 -> [_ w2629]
                      frame False {
                        n1416 = local read "Calc: On/Off"() -> (w2619:dbl)
                        n1417 = Divide(x=w2623, y=3) -> (x/y=w2625:dbl)
                        n1418 = To Word Integer(number=w2625) -> (16bit integer=w2624:i16)
                        n1419 = Format Value(format string="%#g", value (0)=w2619) -> (output string=w2620:string)  [unwired: 1 in]
                        n1420 = Replace Array Subset(array=w2626, new element=w2620, index (row)=w2624, index (col)=1) -> (w2622:string[][])
                      }
                      frame True {
                        n1421 = local read "Calc: On/Off"() -> (w2635:dbl)
                        n1422 = Search 1D Array(1D array=w2631, element="On/Off Current:") -> (index of element=w2638:i32)  [unwired: 1 in]
                        n1423 = Divide(x=w2638, y=3) -> (x/y=w2639:dbl)
                        n1424 = To Word Integer(number=w2639) -> (16bit integer=w2630:i16)
                        n1425 = Format Value(format string="%#g", value (0)=w2635) -> (output string=w2632:string)  [unwired: 1 in]
                        n1426 = Build Array(w2629, w2632) -> (w2637:string[])
                        n1427 = Replace Array Subset(array=w2633, new element=w2637, index (row)=w2630) -> (w2634:string[][])  [unwired: 1 in]
                      }
                    }
                    n1428 = local write "Save1 Array"(w2615) -> ()
                  }
                  frame #8 {
                    w2651 = "Off I-Sat (A):"
                    n1429 = local read "Save1 Array"() -> (w2642:string[][])
                    n1430 = Array Size(array=w2642) -> (size(s)=w2648:i32[])
                    n1431 = Array Subset(array=w2642, index (row)=0, index (col)=0, length (col)=3) -> (w2644:string[][])  [unwired: 1 in]
                    n1432 = Index Array(array=w2648, index=0) -> (element=w2650:i32)
                    n1433 = Reshape Array(w2644, w2650) -> (w2643:string[])
                    n1434 = Search 1D Array(1D array=w2643, element=w2651) -> (index of element=w2654:i32)  [unwired: 1 in]
                    n1435 = Equal?(x=w2654, y=-1) -> (x = y?=w2653:bool)
                    n1436 = case shown="True" w2653 {
                      tunnel: w2642 -> [w2663 w2669]
                      tunnel: w2654 -> [w2660 _]
                      tunnel: [w2659 w2668] -> w2652
                      tunnel: w2643 -> [_ w2667]
                      tunnel: w2651 -> [_ w2666]
                      frame False {
                        n1437 = local read "Calc: Off I-Sat"() -> (w2658:dbl)
                        n1438 = Divide(x=w2660, y=3) -> (x/y=w2662:dbl)
                        n1439 = Format Value(format string="%#g", value (0)=w2658) -> (output string=w2656:string)  [unwired: 1 in]
                        n1440 = To Word Integer(number=w2662) -> (16bit integer=w2661:i16)
                        n1441 = Replace Array Subset(array=w2663, new element=w2656, index (row)=w2661, index (col)=1) -> (w2659:string[][])
                      }
                      frame True {
                        n1442 = local read "Calc: Off I-Sat"() -> (w2670:dbl)
                        n1443 = Search 1D Array(1D array=w2667, element="On/Off I-Sat:") -> (index of element=w2675:i32)  [unwired: 1 in]
                        n1444 = Divide(x=w2675, y=3) -> (x/y=w2676:dbl)
                        n1445 = To Word Integer(number=w2676) -> (16bit integer=w2674:i16)
                        n1446 = Format Value(format string="%#g", value (0)=w2670) -> (output string=w2679:string)  [unwired: 1 in]
                        n1447 = Build Array(w2666, w2679) -> (w2672:string[])
                        n1448 = Increment(x=w2674) -> (x+1=w2673:i16)
                        n1449 = Insert Into Array(array=w2669, index (row)=w2673, new element=w2672) -> (w2668:string[][])  [unwired: 1 in]
                      }
                    }
                    n1450 = local write "Save1 Array"(w2652) -> ()
                  }
                  frame #9 {
                    w2681 = "Vt-Sat (V):"
                    n1451 = local read "Save1 Array"() -> (w2682:string[][])
                    n1452 = Array Size(array=w2682) -> (size(s)=w2687:i32[])
                    n1453 = Array Subset(array=w2682, index (row)=0, index (col)=0, length (col)=3) -> (w2683:string[][])  [unwired: 1 in]
                    n1454 = Index Array(array=w2687, index=0) -> (element=w2689:i32)
                    n1455 = Reshape Array(w2683, w2689) -> (w2680:string[])
                    n1456 = Search 1D Array(1D array=w2680, element=w2681) -> (index of element=w2692:i32)  [unwired: 1 in]
                    n1457 = Equal?(x=w2692, y=-1) -> (x = y?=w2691:bool)
                    n1458 = case shown="True" w2691 {
                      tunnel: w2682 -> [w2699 w2708]
                      tunnel: w2692 -> [w2695 _]
                      tunnel: [w2694 w2707] -> w2690
                      tunnel: w2681 -> [_ w2706]
                      tunnel: w2680 -> [_ w2705]
                      frame False {
                        n1459 = local read "New: VT-Sat"() -> (w2701:dbl)
                        n1460 = Number To Fractional String(number=w2701) -> (F-format string=w2696:string)  [unwired: 3 in]
                        n1461 = Divide(x=w2695, y=3) -> (x/y=w2698:dbl)
                        n1462 = To Word Integer(number=w2698) -> (16bit integer=w2697:i16)
                        n1463 = Replace Array Subset(array=w2699, new element=w2696, index (row)=w2697, index (col)=1) -> (w2694:string[][])
                      }
                      frame True {
                        n1464 = local read "New: VT-Sat"() -> (w2709:dbl)
                        n1465 = Search 1D Array(1D array=w2705, element="Threshold V (V):") -> (index of element=w2704:i32)  [unwired: 1 in]
                        n1466 = Divide(x=w2704, y=3) -> (x/y=w2712:dbl)
                        n1467 = To Word Integer(number=w2712) -> (16bit integer=w2703:i16)
                        n1468 = Format Value(format string="%#g", value (0)=w2709) -> (output string=w2715:string)  [unwired: 1 in]
                        n1469 = Build Array(w2706, w2715) -> (w2711:string[])
                        n1470 = Replace Array Subset(array=w2708, new element=w2711, index (row)=w2703) -> (w2707:string[][])  [unwired: 1 in]
                      }
                    }
                    n1471 = local write "Save1 Array"(w2690) -> ()
                  }
                  frame #10 {
                    n1472 = local read "Save1 Array"() -> (w2716:string[][])
                    n1473 = Array Size(array=w2716) -> (size(s)=w2722:i32[])
                    n1474 = Array Subset(array=w2716, index (row)=0, index (col)=0, length (col)=3) -> (w2718:string[][])  [unwired: 1 in]
                    n1475 = Index Array(array=w2722, index=0) -> (element=w2724:i32)
                    n1476 = Reshape Array(w2718, w2724) -> (w2717:string[])
                    n1477 = Search 1D Array(1D array=w2717, element="VT-Lin (V):") -> (index of element=w2727:i32)  [unwired: 1 in]
                    n1478 = Equal?(x=w2727, y=-1) -> (x = y?=w2726:bool)
                    n1479 = case shown="False" w2726 {
                      tunnel: w2716 -> [w2737 w2740]
                      tunnel: w2727 -> [w2734 _]
                      tunnel: [w2733 w2740] -> w2725
                      frame False {
                        n1480 = local read "New: VT-Lin"() -> (w2731:dbl)
                        n1481 = Divide(x=w2734, y=3) -> (x/y=w2736:dbl)
                        n1482 = Format Value(format string="%#g", value (0)=w2731) -> (output string=w2730:string)  [unwired: 1 in]
                        n1483 = To Word Integer(number=w2736) -> (16bit integer=w2735:i16)
                        n1484 = Replace Array Subset(array=w2737, new element=w2730, index (row)=w2735, index (col)=1) -> (w2733:string[][])
                      }
                      frame True {
                      }
                    }
                    n1485 = local write "Save1 Array"(w2725) -> ()
                  }
                  frame #11 {
                    w2741 = "STS-Sat (V/decade):"
                    n1486 = local read "Save1 Array"() -> (w2743:string[][])
                    n1487 = Array Size(array=w2743) -> (size(s)=w2748:i32[])
                    n1488 = Array Subset(array=w2743, index (row)=0, index (col)=0, length (col)=3) -> (w2744:string[][])  [unwired: 1 in]
                    n1489 = Index Array(array=w2748, index=0) -> (element=w2750:i32)
                    n1490 = Reshape Array(w2744, w2750) -> (w2742:string[])
                    n1491 = Search 1D Array(1D array=w2742, element=w2741) -> (index of element=w2753:i32)  [unwired: 1 in]
                    n1492 = Equal?(x=w2753, y=-1) -> (x = y?=w2752:bool)
                    n1493 = case shown="True" w2752 {
                      tunnel: w2743 -> [w2762 w2768]
                      tunnel: w2753 -> [w2759 _]
                      tunnel: [w2758 w2769] -> w2751
                      tunnel: w2742 -> [_ w2767]
                      tunnel: w2741 -> [_ w2766]
                      frame False {
                        n1494 = local read "New: STS"() -> (w2756:dbl)
                        n1495 = Divide(x=w2759, y=3) -> (x/y=w2761:dbl)
                        n1496 = Format Value(format string="%#g", value (0)=w2756) -> (output string=w2755:string)  [unwired: 1 in]
                        n1497 = To Word Integer(number=w2761) -> (16bit integer=w2760:i16)
                        n1498 = Replace Array Subset(array=w2762, new element=w2755, index (row)=w2760, index (col)=1) -> (w2758:string[][])
                      }
                      frame True {
                        n1499 = local read "New: STS"() -> (w2770:dbl)
                        n1500 = Search 1D Array(1D array=w2767, element="S.T.S. (V/decade):") -> (index of element=w2773:i32)  [unwired: 1 in]
                        n1501 = Divide(x=w2773, y=3) -> (x/y=w2774:dbl)
                        n1502 = To Word Integer(number=w2774) -> (16bit integer=w2765:i16)
                        n1503 = Format Value(format string="%#g", value (0)=w2770) -> (output string=w2777:string)  [unwired: 1 in]
                        n1504 = Build Array(w2766, w2777) -> (w2772:string[])
                        n1505 = Replace Array Subset(array=w2768, new element=w2772, index (row)=w2765) -> (w2769:string[][])  [unwired: 1 in]
                      }
                    }
                    n1506 = local write "Save1 Array"(w2751) -> ()
                  }
                  frame #12 {
                    w2778 = "Trap Density-VT (Traps/Vcm^2):"
                    n1507 = local read "Save1 Array"() -> (w2780:string[][])
                    n1508 = Array Size(array=w2780) -> (size(s)=w2785:i32[])
                    n1509 = Array Subset(array=w2780, index (row)=0, index (col)=0, length (col)=3) -> (w2781:string[][])  [unwired: 1 in]
                    n1510 = Index Array(array=w2785, index=0) -> (element=w2787:i32)
                    n1511 = Reshape Array(w2781, w2787) -> (w2779:string[])
                    n1512 = Search 1D Array(1D array=w2779, element=w2778) -> (index of element=w2790:i32)  [unwired: 1 in]
                    n1513 = Equal?(x=w2790, y=-1) -> (x = y?=w2789:bool)
                    n1514 = case shown="True" w2789 {
                      tunnel: w2780 -> [w2799 w2804]
                      tunnel: w2790 -> [w2795 _]
                      tunnel: [w2794 w2805] -> w2788
                      tunnel: w2779 -> [_ w2803]
                      tunnel: w2778 -> [_ w2802]
                      frame False {
                        n1515 = local read "New: Trap Density-VT"() -> (w2793:dbl)
                        n1516 = Format Value(format string="%#g", value (0)=w2793) -> (output string=w2796:string)  [unwired: 1 in]
                        n1517 = Divide(x=w2795, y=3) -> (x/y=w2798:dbl)
                        n1518 = To Word Integer(number=w2798) -> (16bit integer=w2797:i16)
                        n1519 = Replace Array Subset(array=w2799, new element=w2796, index (row)=w2797, index (col)=1) -> (w2794:string[][])
                      }
                      frame True {
                        n1520 = local read "New: Trap Density-VT"() -> (w2815:dbl)
                        n1521 = Search 1D Array(1D array=w2803, element="STS-Sat (V/decade):") -> (index of element=w2810:i32)  [unwired: 1 in]
                        n1522 = Divide(x=w2810, y=3) -> (x/y=w2809:dbl)
                        n1523 = To Word Integer(number=w2809) -> (16bit integer=w2811:i16)
                        n1524 = Format Value(format string="%#g", value (0)=w2815) -> (output string=w2806:string)  [unwired: 1 in]
                        n1525 = Build Array(w2802, w2806) -> (w2813:string[])
                        n1526 = Increment(x=w2811) -> (x+1=w2812:i16)
                        n1527 = Insert Into Array(array=w2804, index (row)=w2812, new element=w2813) -> (w2805:string[][])  [unwired: 1 in]
                      }
                    }
                    n1528 = local write "Save1 Array"(w2788) -> ()
                  }
                  frame #13 {
                    w2817 = "Trap Density-STS (Traps/Vcm^2):"
                    n1529 = local read "Save1 Array"() -> (w2819:string[][])
                    n1530 = Array Size(array=w2819) -> (size(s)=w2824:i32[])
                    n1531 = Array Subset(array=w2819, index (row)=0, index (col)=0, length (col)=3) -> (w2820:string[][])  [unwired: 1 in]
                    n1532 = Index Array(array=w2824, index=0) -> (element=w2826:i32)
                    n1533 = Reshape Array(w2820, w2826) -> (w2818:string[])
                    n1534 = Search 1D Array(1D array=w2818, element=w2817) -> (index of element=w2828:i32)  [unwired: 1 in]
                    n1535 = Equal?(x=w2828, y=-1) -> (x = y?=w2827:bool)
                    n1536 = case shown="True" w2827 {
                      tunnel: w2819 -> [w2837 w2842]
                      tunnel: w2828 -> [w2834 _]
                      tunnel: [w2833 w2843] -> w2816
                      tunnel: w2818 -> [_ w2841]
                      tunnel: w2817 -> [_ w2840]
                      frame False {
                        n1537 = local read "New: Trap Density-STS"() -> (w2831:dbl)
                        n1538 = Divide(x=w2834, y=3) -> (x/y=w2836:dbl)
                        n1539 = To Word Integer(number=w2836) -> (16bit integer=w2835:i16)
                        n1540 = Format Value(format string="%#g", value (0)=w2831) -> (output string=w2830:string)  [unwired: 1 in]
                        n1541 = Replace Array Subset(array=w2837, new element=w2830, index (row)=w2835, index (col)=1) -> (w2833:string[][])
                      }
                      frame True {
                        n1542 = local read "New: Trap Density-STS"() -> (w2844:dbl)
                        n1543 = Search 1D Array(1D array=w2841, element="Trap Density-VT (Traps/Vcm^2):") -> (index of element=w2849:i32)  [unwired: 1 in]
                        n1544 = Divide(x=w2849, y=3) -> (x/y=w2850:dbl)
                        n1545 = To Word Integer(number=w2850) -> (16bit integer=w2848:i16)
                        n1546 = Format Value(format string="%#g", value (0)=w2844) -> (output string=w2853:string)  [unwired: 1 in]
                        n1547 = Build Array(w2840, w2853) -> (w2846:string[])
                        n1548 = Increment(x=w2848) -> (x+1=w2847:i16)
                        n1549 = Insert Into Array(array=w2842, index (row)=w2847, new element=w2846) -> (w2843:string[][])  [unwired: 1 in]
                      }
                    }
                    n1550 = local write "Save1 Array"(w2816) -> ()
                  }
                }
                n1551 = String To Path(string=w2390) -> (path=w2373:path)
                "No Image 2" <- w2373
              }
              frame #1 {
                n1552 = Equal?(x=w2857, y=w2856) -> (x = y?=w2855:bool)
                n1553 = case shown="False" w2855 {
                  tunnel: w2857 -> [w2861 _]
                  tunnel: w2856 -> [w2860 _]
                  frame False {
                    n1554 = Move(source path=w2861, 9:TRUE, 10:w2860) -> ()  [unwired: 2 in, 3 out]
                  }
                  frame True {
                  }
                }
              }
              frame #2 {
                n1555 = local write "Transfer File"(w2863) -> ()
                n1556 = call-poly <vilib>:"Write To Spreadsheet File.vi"("2D data"=w2862, "file path (dialog if empty)"=w2863) -> ()  [unwired: 6 in, 1 out]
              }
              frame #3 {
                w2968 = 0
                # "Moves to next file and displays new image/data"
                n1557 = property on="Image Out" class="ImageControl"() -> (error out=w2930:errorcluster, "Image Center Position"=w2934:cluster{"X":u32, "Y":u32})  [unwired: 2 in, 1 out]
                n1558 = local read "Transfer File"() -> (w2973:path)
                n1559 = Strip Path(path=w2973) -> (stripped path=w2964:path, name=w2982:string)
                n1560 = Unbundle(w2934) -> ("X"=w2932:u32)  [unwired: 1 out]
                n1561 = local write "Transfer Folder"(w2964) -> ()
                n1562 = Bundle("X"=w2932, 0) -> (w2933:cluster{"X":u32, i32})  [unwired: 1 in]
                n1563 = property on="Image Out" class="ImageControl"(error in=w2930, "Image Center Position"=w2933) -> ()  [unwired: 1 in, 2 out]
                n1564 = List Folder(path=w2964) -> (filenames=w2978:string[])  [unwired: 3 in, 3 out]
                n1565 = Search 1D Array(1D array=w2978, element=w2982) -> (index of element=w2975:i32)  [unwired: 1 in]
                n1566 = Array Size(array=w2978) -> (size(s)=w2974:i32)
                n1567 = Decrement(x=w2974) -> (x-1=w2976:i32)
                n1568 = Equal?(x=w2975, y=w2976) -> (x = y?=w2977:bool)
                n1569 = local read "Folder Index"() -> (w2926:dbl)
                n1570 = case shown="False" w2977 {
                  tunnel: w2926 -> [w3107 _]
                  tunnel: [w3106 0] -> w2925
                  frame False {
                    n1571 = Increment(x=w3107) -> (x+1=w3106:dbl)
                  }
                  frame True {
                  }
                }
                n1572 = invoke on="Image Out" class="ImageControl" method="Clear ROI"() -> ()  [unwired: 3 in, 3 out]
                n1573 = local write "Folder Index"(w2925) -> ()
                n1574 = Path To String(path=w2964) -> (string=w2983:string)
                n1575 = Index Array(array=w2978, index=w2925) -> (element=w2979:string)
                n1576 = local write "Data Name:"(w2979) -> ()
                n1577 = Concatenate Strings(w2983, "\\", w2979) -> (w2981:string)
                n1578 = String To Path(string=w2981) -> (path=w2879:path)
                n1579 = call "Recorded Values.vi"("Path"=w2879) -> ("Recorded Char"=w2881:T6, "Recorded Prop"=w2882:T7, "Fabrication Prop"=w2880:T8)  [unwired: 8 in]
                n1580 = Unbundle By Name(w2881) -> ("Mobility-Sat"=w2894:dbl, "Moblitity-Lin"=w2895:dbl, "On/Off"=w2896:dbl, "Off Current"=w2897:dbl, "Vt-Sat"=w2873:dbl, "STS"=w2898:dbl, "Trap Density-VT"=w2899:dbl, "Trap Density-STS"=w2900:dbl)
                n1581 = Unbundle By Name(w2882) -> ("Date Recorded"=w2890:string, "Index"=w2891:string, "Length"=w2892:dbl, "Width"=w2893:dbl, "Sample Temp"=w2876:dbl)
                n1582 = Unbundle By Name(w2880) -> ("Date Created"=w2901:string, "Material"=w2883:string, "Solvent"=w2884:string, "Concentration"=w2885:dbl, "Method"=w2886:string, "Dielectric (nm)"=w2887:dbl, "Treatment"=w2888:string, "Comments"=w2889:string)
                n1583 = local write "Rec: Off I-Sat"(w2897) -> ()
                n1584 = local write "Rec: Comments"(w2889) -> ()
                n1585 = local write "Rec: VT-Sat"(w2873) -> ()
                n1586 = local write "Date Created"(w2901) -> ()
                n1587 = local write "Rec: Material"(w2883) -> ()
                n1588 = local write "Rec: Solvent"(w2884) -> ()
                n1589 = local write "Rec: Concentration"(w2885) -> ()
                n1590 = local write "Rec: Method"(w2886) -> ()
                n1591 = local write "Rec: Dielectric (d)"(w2887) -> ()
                n1592 = local write "Surface Treatment:"(w2888) -> ()
                n1593 = local write "Index"(w2891) -> ()
                n1594 = local write "Rec: Mobility-Sat"(w2894) -> ()
                n1595 = local write "Rec: Mobility-Lin"(w2895) -> ()
                n1596 = local write "Rec: On/Off"(w2896) -> ()
                n1597 = local write "Rec: STS"(w2898) -> ()
                n1598 = local write "Rec: Trap Density-VT"(w2899) -> ()
                n1599 = local write "Rec: Trap Density-STS"(w2900) -> ()
                n1600 = local write "Date Recorded"(w2890) -> ()
                n1601 = local write "Rec: Length"(w2892) -> ()
                n1602 = local write "Rec: Width"(w2893) -> ()
                n1603 = local write "Rec: Temp"(w2876) -> ()
                n1604 = Equal To 0?(x=w2876) -> (x = 0?=w2877:bool)
                n1605 = case shown="False" w2877 {
                  tunnel: [w2984 w2985] -> w2874
                  tunnel: w2876 -> [w2984 _]
                  frame False {
                  }
                  frame True {
                    n1606 = local read "Room Temp"() -> (w2985:dbl)
                  }
                }
                n1607 = local read "NumPoints Log"() -> (w2922:dbl)
                n1608 = local write "Transfer File"(w2879) -> ()
                n1609 = local read "Num Pts"() -> (w2911:dbl)
                n1610 = local read "Num Pts"() -> (w2923:dbl)
                n1611 = call-poly <vilib>:"Read From Spreadsheet File.vi"("file path (dialog if empty)"=w2879) -> ("all rows"=w2970:string[][])  [unwired: 6 in, 4 out]
                n1612 = call "Mobility-Vt Calculator-File.vi"("NumPts"=w2923, "Path"=w2879) -> ("Graph Cluster"=w2870:T9, "Output"=w2924:T10, "Index-Sat"=w2904:dbl, "Index-Lin"=w2910:dbl)  [unwired: 5 in, 1 out]
                n1613 = Unbundle By Name(w2870) -> ("Raw Sat"=w2867:cluster{dbl[], dbl[]}[], "Sqrt Sat"=w2869:cluster{dbl[], dbl[]}[], "Log Sat"=w2866:cluster{dbl[], dbl[]}[], "Raw Lin"=w2865:cluster{dbl[], dbl[]}[], "Sqrt Lin"=w2868:cluster{dbl[], dbl[]}[], "Log Lin"=w2864:cluster{dbl[], dbl[]}[])
                n1614 = Decimate 1D Array(w2868) -> (w2918:cluster{dbl[], dbl[]}[])  [unwired: 1 out]
                n1615 = Array To Cluster(array=w2918) -> (cluster=w2916:T11)
                n1616 = Unbundle(w2916) -> ("[0]"=w2917:cluster{dbl[], dbl[]})  [unwired: 8 out]
                n1617 = Unbundle(w2917) -> (w2915:dbl[], w2914:dbl[])
                n1618 = Array Subset(array=w2914, index=w2910, length=w2911) -> (w2912:dbl[])
                n1619 = Array Subset(array=w2915, index=w2910, length=w2911) -> (w2913:dbl[])
                n1620 = call "STS Calculator-File.vi"("NumPts"=w2922, "Path"=w2879) -> ("STS Index-Sat"=w2921:dbl, "XY Graph-Sat"=w2920:cluster{dbl[], dbl[]}[], "Ouput"=w2919:cluster{"STS-Sat":dbl, "STS-Lin":dbl})  [unwired: 5 in, 2 out]
                n1621 = local read "New: Dielectric"() -> (w2906:dbl)
                n1622 = local write "Sat-Trans Slider"(w2904) -> ()
                n1623 = local write "Lin Id-Used"(w2912) -> ()
                n1624 = local write "Lin-Vg Array-Used"(w2913) -> ()
                n1625 = local write "MobVi Index"(w2904) -> ()
                n1626 = local write "Index 2"(w2921) -> ()
                n1627 = local write "Sqrt-Sat"(w2869) -> ()
                n1628 = local write "Log-Sat"(w2920) -> ()
                n1629 = Unbundle By Name(w2924) -> ("Mobility-Sat"=w2909:dbl, "Vt-Sat"=w2871:dbl, "Mobility-Lin"=w2908:dbl, "Mobility-Lin"=w2907:dbl, "Off I-Sat"=w2902:dbl, "On/Off I-Sat"=w2872:dbl)
                n1630 = local write "Sqrt-Lin"(w2868) -> ()
                n1631 = Array Size(array=w2970) -> (size(s)=w2969:i32[])
                n1632 = local write "Raw- Sat"(w2867) -> ()
                n1633 = local write "New: Temp"(w2874) -> ()
                n1634 = Unbundle By Name(w2919) -> ("STS-Sat"=w2905:dbl)
                n1635 = call "Trap Density_STS.vi"("Temp (T) [K]"=w2874, "S.T.S. (S)"=w2905, "Dielectric"=w2906) -> ("Trap Density (N)"=w2878:dbl)  [unwired: 8 in]
                n1636 = local write "Calc: Mobility-Lin"(w2908) -> ()
                n1637 = local write "Raw- Lin"(w2865) -> ()
                n1638 = local write "Log-Sat"(w2866) -> ()
                n1639 = local write "Calc: Mobility-Sat"(w2909) -> ()
                n1640 = local write "Log-Lin"(w2864) -> ()
                n1641 = local write "Calc: Off I-Sat"(w2902) -> ()
                n1642 = local write "Calc: VT-Sat"(w2871) -> ()
                n1643 = local write "New: VT-Lin"(w2907) -> ()
                n1644 = local write "New: Trap Density-STS"(w2878) -> ()
                n1645 = local write "Calc: Trap Density-STS"(w2878) -> ()
                n1646 = local read "Image Folder"() -> (w2958:path)
                n1647 = local read "New: Dielectric"() -> (w2903:dbl)
                n1648 = Decimate 1D Array(w2869) -> (w2953:cluster{dbl[], dbl[]}[])  [unwired: 1 out]
                n1649 = Decimate 1D Array(w2920) -> (w2943:cluster{dbl[], dbl[]}[])  [unwired: 1 out]
                n1650 = Index Array(array=w2969, index=w2968) -> (element=w2949:i32)
                n1651 = Array Subset(array=w2970, index (row)=w2968, index (col)=w2968, length (col)=3) -> (w2971:string[][])  [unwired: 1 in]
                n1652 = local write "Calc: STS"(w2905) -> ()
                n1653 = local write "New: VT-Sat"(w2871) -> ()
                n1654 = local write "New: Mobility-Sat"(w2909) -> ()
                n1655 = local write "Calc: On/Off"(w2872) -> ()
                n1656 = local write "New: Mobility-Lin"(w2908) -> ()
                n1657 = List Folder(path=w2958) -> (filenames=w2963:string[])  [unwired: 3 in, 3 out]
                n1658 = local write "New: VT-Lin"(w2907) -> ()
                n1659 = Array To Cluster(array=w2953) -> (cluster=w2955:T11)
                n1660 = Array To Cluster(array=w2943) -> (cluster=w2941:T11)
                n1661 = Reshape Array(w2971, w2949) -> (w2956:string[])
                n1662 = Subtract(x=w2949, y=20) -> (x-y=w2948:i32)
                n1663 = local write "New: STS"(w2905) -> ()
                n1664 = property on="Sat-Trans Slider" class="Slide (strict)"("Scale.Maximum"=w2948) -> ()  [unwired: 2 in, 2 out]
                n1665 = call "Trap Density_VT.vi"("VT"=w2871, "Dielectric"=w2903) -> ("Trap Density-VT"=w2875:dbl)
                n1666 = Unbundle(w2955) -> ("[0]"=w2954:cluster{dbl[], dbl[]})  [unwired: 8 out]
                n1667 = Unbundle(w2941) -> ("[0]"=w2942:cluster{dbl[], dbl[]})  [unwired: 8 out]
                n1668 = Search 1D Array(1D array=w2956, element="Index:") -> (index of element=w2965:i32)  [unwired: 1 in]
                n1669 = local write "New: Trap Density-VT"(w2875) -> ()
                n1670 = local write "Calc: Trap Density-VT"(w2875) -> ()
                n1671 = Unbundle(w2954) -> (w2945:dbl[], w2944:dbl[])
                n1672 = Unbundle(w2942) -> (w2940:dbl[], w2939:dbl[])
                n1673 = Increment(x=w2965) -> (x+1=w2966:i32)
                n1674 = Array Subset(array=w2945, index=w2904, length=w2923) -> (w2952:dbl[])
                n1675 = Array Subset(array=w2944, index=w2904, length=w2923) -> (w2951:dbl[])
                n1676 = Array Subset(array=w2940, index=w2921, length=w2922) -> (w2947:dbl[])
                n1677 = Array Subset(array=w2939, index=w2921, length=w2922) -> (w2946:dbl[])
                n1678 = Index Array(array=w2956, index=w2966) -> (element=w2961:string)
                n1679 = local write "Vg Array-Log-Used"(w2946) -> ()
                n1680 = local write "Sat Id-Log-Used"(w2947) -> ()
                n1681 = local write "Sat Id-Used"(w2951) -> ()
                n1682 = local write "Index"(w2961) -> ()
                n1683 = local write "Sat Vg Array-Used"(w2952) -> ()
                n1684 = while {
                  tunnel: w2963 -> [w2993]
                  tunnel: w2961 -> [w2991]
                  tunnel: [w2990] -> _
                  tunnel: [w2990] -> w2962
                  tunnel: w2949 -> [w2989]
                  i -> [w2990]
                  stop <- w2986 stop-if-true
                  n1685 = Index Array(array=w2993, index=w2990) -> (element=w2994:string)
                  n1686 = xnode "Match Regular Expression"("input string"=w2994, "regular expression"=w2991) -> ("whole match"=w2992:string)  [unwired: 4 in, 4 out]
                  n1687 = Equal?(x=w2992, y=w2991) -> (x = y?=w2988:bool)
                  n1688 = Equal?(x=w2989, y=w2990) -> (x = y?=w2987:bool)
                  n1689 = Or(x=w2988, y=w2987) -> (x .or. y?=w2986:bool)
                }
                n1690 = Path To String(path=w2958) -> (string=w2960:string)
                n1691 = Index Array(array=w2963, index=w2962) -> (element=w2937:string)
                n1692 = local write "Image Name"(w2937) -> ()
                n1693 = Empty String/Path?(string/path=w2937) -> (empty?=w2938:bool)
                n1694 = Concatenate Strings(w2960, "\\", w2937) -> (w2959:string)
                n1695 = String To Path(string=w2959) -> (path=w2936:path)
                n1696 = local read "No Image File"() -> (w2935:path)
                n1697 = Select(t=w2935, s=w2938, f=w2936) -> (s? t:f=w2929:path)
                n1698 = local write "Image File"(w2929) -> ()
                n1699 = local read "Image Out"() -> (w2927:T2)
                n1700 = call "IMAQ ReadFile"("File Path"=w2929, "Image"=w2927) -> ("Image Out"=w2928:T2)  [unwired: 5 in, 4 out]
                n1701 = local write "Image Out"(w2928) -> ()
                n1702 = local write "Image Out 2"(w2928) -> ()
              }
              frame #4 {
                # "Output ROI data"
                n1703 = local read "Image Folder"() -> (w3109:path)
                n1704 = Build Path(base path=w3109, name or relative path="ROI") -> (appended path=w3111:path)
                n1705 = local read "Index"() -> (w3110:string)
                n1706 = Build Path(base path=w3111, name or relative path=w3110) -> (appended path=w3116:path)
                n1707 = invoke on="Image Out" class="ImageControl" method="Clear ROI"() -> (error out=w3115:errorcluster)  [unwired: 3 in, 2 out]
                n1708 = call <vilib>:"Check if File or Folder Exists.vi"("error in (no error)"=w3115, "path"=w3116) -> ("file or folder exists?"=w3113:bool, "dup path"=w3114:path)  [unwired: 7 in, 1 out]
                n1709 = case shown="True" w3113 {
                  tunnel: w3114 -> [_ w3117]
                  frame False {
                  }
                  frame True {
                    n1710 = Read from Text File(file (use dialog)=w3117) -> (text=w3121:string)  [unwired: 3 in, 3 out]
                    n1711 = property on="Image Out" class="ImageControl"() -> ("ROI"=w3118:T12)  [unwired: 2 in, 2 out]
                    n1712 = Unflatten From String(type=w3118, binary string=w3121) -> (value=w3119:T12, error out=w3120:errorcluster)  [unwired: 3 in, 1 out]
                    n1713 = property on="Image Out" class="ImageControl"(error in=w3120, "ROI"=w3119) -> ()  [unwired: 1 in, 2 out]
                  }
                }
              }
            }
            n1714 = flat-sequence {
              tunnel: [w2330] -> w2317
              tunnel: w2317 -> [w2344]
              frame #0 {
                # "Makes Empty File for Transformer Data"
                n1715 = local read "Transfer Folder"() -> (w2319:path)
                n1716 = Build Path(base path=w2319, name or relative path="Stats") -> (appended path=w2321:path)
                n1717 = call <vilib>:"Check if File or Folder Exists.vi"("path"=w2321) -> ("file or folder exists?"=w2322:bool, "dup path"=w2323:path)  [unwired: 8 in, 1 out]
                n1718 = case shown="False" w2322 {
                  tunnel: [w2327 w2329] -> w2324
                  tunnel: w2323 -> [w2328 w2329]
                  frame False {
                    n1719 = Create Folder(path (use dialog)=w2328) -> (created path=w2327:path)  [unwired: 2 in, 2 out]
                  }
                  frame True {
                  }
                }
                n1720 = Build Path(base path=w2324, name or relative path="Tranformer Data.txt") -> (appended path=w2326:path)
                n1721 = call-poly <vilib>:"Write To Spreadsheet File.vi"("append to file? (new file:F)"=TRUE, "file path (dialog if empty)"=w2326) -> ()  [unwired: 6 in, 1 out]
              }
              frame #1 {
                # "Adds Headers if they don't exist"
                n1722 = local read "Transfer Folder"() -> (w2336:path)
                n1723 = Concatenate Strings("Stats\\", "Tranformer Data.txt") -> (w2337:string)
                n1724 = Build Path(base path=w2336, name or relative path=w2337) -> (appended path=w2330:path)
                n1725 = call-poly <vilib>:"Read From Spreadsheet File.vi"("file path (dialog if empty)"=w2330) -> ("first row"=w2335:string[])  [unwired: 6 in, 4 out]
                n1726 = Search 1D Array(1D array=w2335, element="DeviceID") -> (index of element=w2333:i32)  [unwired: 1 in]
                n1727 = Equal?(x=w2333, y=0) -> (x = y?=w2331:bool)
                n1728 = case shown="False" w2331 {
                  tunnel: w2330 -> [w2341 _]
                  frame False {
                    n1729 = local read "Transformer \nHeaders"() -> (w2340:string[])
                    n1730 = call-poly <vilib>:"Write To Spreadsheet File.vi"("1D data"=w2340, "file path (dialog if empty)"=w2341) -> ()  [unwired: 6 in, 1 out]
                  }
                  frame True {
                  }
                }
              }
              frame #2 {
                # "Adds current device if it doesn't exist"
                n1731 = local read "Current \nRecord"() -> (w2347:string[])
                n1732 = Index Array(array=w2347, index=0) -> (element=w2346:string)
                n1733 = local read "Transfer Folder"() -> (w2349:path)
                n1734 = Concatenate Strings("Stats\\", "Tranformer Data.txt") -> (w2350:string)
                n1735 = local write "Current Device ID"(w2346) -> ()
                n1736 = local read "Current Device ID"() -> (w2356:string)
                n1737 = Build Path(base path=w2349, name or relative path=w2350) -> (appended path=w2348:path)
                n1738 = call-poly <vilib>:"Read From Spreadsheet File.vi"("file path (dialog if empty)"=w2348) -> ("all rows"=w2343:string[][])  [unwired: 6 in, 4 out]
                n1739 = Index Array(array=w2343, index (col)=0) -> (element=w2354:string[])  [unwired: 1 in]
                n1740 = Search 1D Array(1D array=w2354, element=w2356) -> (index of element=w2342:i32)  [unwired: 1 in]
                n1741 = Equal?(x=w2342, y=-1) -> (x = y?=w2345:bool)
                n1742 = case shown="False" w2345 {
                  tunnel: w2344 -> [w2358 w2371]
                  tunnel: w2342 -> [w2363 _]
                  tunnel: w2343 -> [w2364 _]
                  frame False {
                    n1743 = local read "Current \nRecord"() -> (w2362:string[])
                    n1744 = Replace Array Subset(array=w2364, new element=w2362, index (row)=w2363) -> (w2359:string[][])  [unwired: 1 in]
                    n1745 = flat-sequence {
                      tunnel: [w2365] -> _
                      tunnel: [w2366] -> _
                      tunnel: [w2366] -> w2361
                      tunnel: [w2365] -> w2360
                      tunnel: w2359 -> [w2366]
                      tunnel: w2358 -> [w2365]
                      tunnel: w2361 -> [w2368]
                      tunnel: w2360 -> [w2367]
                      frame #0 {
                        n1746 = Delete(path (use dialog)=w2365) -> ()  [unwired: 4 in, 3 out]
                      }
                      frame #1 {
                        n1747 = call-poly <vilib>:"Write To Spreadsheet File.vi"("append to file? (new file:F)"=TRUE, "2D data"=w2368, "file path (dialog if empty)"=w2367) -> ()  [unwired: 5 in, 1 out]
                      }
                    }
                  }
                  frame True {
                    n1748 = local read "Current \nRecord"() -> (w2370:string[])
                    n1749 = call-poly <vilib>:"Write To Spreadsheet File.vi"("append to file? (new file:F)"=TRUE, "1D data"=w2370, "file path (dialog if empty)"=w2371) -> ()  [unwired: 5 in, 1 out]
                  }
                }
              }
            }
          }
          event "Export": Mouse Down {
            n1750 = event-data() -> ()  [unwired: 1 in, 7 out]
            n1751 = flat-sequence {
              frame #0 {
                n1752 = stacked-sequence {
                  frame #0 {
                    n1753 = local read "Independant Variable"() -> (w3123:string)
                    n1754 = Equal?(x=w3123, y="Length (um):") -> (x = y?=w3124:bool)
                    n1755 = case shown="True" w3124 {
                      frame False {
                      }
                      frame True {
                        n1756 = local write "X Axis Display Type"("1") -> ()
                        n1757 = local write "Opj X Axis"("2") -> ()
                      }
                    }
                  }
                  frame #1 {
                    n1758 = local read "Independant Variable"() -> (w3128:string)
                    n1759 = Equal?(x=w3128, y="Sample Temp (K):") -> (x = y?=w3129:bool)
                    n1760 = case shown="True" w3129 {
                      frame False {
                      }
                      frame True {
                        n1761 = local write "X Axis Display Type"("1") -> ()
                        n1762 = local write "Opj X Axis"("1") -> ()
                      }
                    }
                  }
                  frame #2 {
                    n1763 = local read "Independant Variable"() -> (w3133:string)
                    n1764 = Equal?(x=w3133, y="Mobility-Sat (cm^2/Vs):") -> (x = y?=w3134:bool)
                    n1765 = case shown="True" w3134 {
                      frame False {
                      }
                      frame True {
                        n1766 = local write "X Axis Display Type"("2") -> ()
                        n1767 = local write "Opj X Axis"("2") -> ()
                      }
                    }
                  }
                  frame #3 {
                    n1768 = local read "Independant Variable"() -> (w3138:string)
                    n1769 = Equal?(x=w3138, y="Mobility-Lin (cm^2/Vs):") -> (x = y?=w3139:bool)
                    n1770 = case shown="True" w3139 {
                      frame False {
                      }
                      frame True {
                        n1771 = local write "X Axis Display Type"("2") -> ()
                        n1772 = local write "Opj X Axis"("2") -> ()
                      }
                    }
                  }
                  frame #4 {
                    n1773 = local read "Independant Variable"() -> (w3143:string)
                    n1774 = Equal?(x=w3143, y="On/Off I-Sat:") -> (x = y?=w3144:bool)
                    n1775 = case shown="True" w3144 {
                      frame False {
                      }
                      frame True {
                        n1776 = local write "X Axis Display Type"("2") -> ()
                        n1777 = local write "Opj X Axis"("2") -> ()
                      }
                    }
                  }
                  frame #5 {
                    n1778 = local read "Independant Variable"() -> (w3148:string)
                    n1779 = Equal?(x=w3148, y="Off I-Sat (A):") -> (x = y?=w3149:bool)
                    n1780 = case shown="True" w3149 {
                      frame False {
                      }
                      frame True {
                        n1781 = local write "X Axis Display Type"("2") -> ()
                        n1782 = local write "Opj X Axis"("2") -> ()
                      }
                    }
                  }
                  frame #6 {
                    n1783 = local read "Independant Variable"() -> (w3153:string)
                    n1784 = Equal?(x=w3153, y="Vt-Sat (V):") -> (x = y?=w3154:bool)
                    n1785 = case shown="True" w3154 {
                      frame False {
                      }
                      frame True {
                        n1786 = local write "X Axis Display Type"("1") -> ()
                        n1787 = local write "Opj X Axis"("1") -> ()
                      }
                    }
                  }
                  frame #7 {
                    n1788 = local read "Independant Variable"() -> (w3158:string)
                    n1789 = Equal?(x=w3158, y="STS-Sat (V/decade):") -> (x = y?=w3159:bool)
                    n1790 = case shown="True" w3159 {
                      frame False {
                      }
                      frame True {
                        n1791 = local write "X Axis Display Type"("1") -> ()
                        n1792 = local write "Opj X Axis"("1") -> ()
                      }
                    }
                  }
                  frame #8 {
                    n1793 = local read "Independant Variable"() -> (w3163:string)
                    n1794 = Equal?(x=w3163, y="Trap Density-VT (Traps/Vcm^2):") -> (x = y?=w3164:bool)
                    n1795 = case shown="True" w3164 {
                      frame False {
                      }
                      frame True {
                        n1796 = local write "X Axis Display Type"("2") -> ()
                        n1797 = local write "Opj X Axis"("2") -> ()
                      }
                    }
                  }
                  frame #9 {
                    n1798 = local read "Independant Variable"() -> (w3168:string)
                    n1799 = Equal?(x=w3168, y="Trap Density-STS (Traps/Vcm^2):") -> (x = y?=w3169:bool)
                    n1800 = case shown="True" w3169 {
                      frame False {
                      }
                      frame True {
                        n1801 = local write "X Axis Display Type"("2") -> ()
                        n1802 = local write "Opj X Axis"("2") -> ()
                      }
                    }
                  }
                }
              }
              frame #1 {
                n1803 = local read "Transfer Folder"() -> (w3177:path)
                n1804 = Build Path(base path=w3177, name or relative path="Stats") -> (appended path=w3178:path)
                n1805 = local read "Origin Project File"() -> (w3189:path)
                n1806 = call <vilib>:"Check if File or Folder Exists.vi"("path"=w3178) -> ("file or folder exists?"=w3193:bool, "dup path"=w3192:path)  [unwired: 8 in, 1 out]
                n1807 = call <userlib>:"OA_ConnectToOrigin.vi"() -> ("error out"=w3190:errorcluster, "Origin.IOApplication"=w3191:refnum<k7>)  [unwired: 8 in]
                n1808 = case shown="False" w3193 {
                  tunnel: w3192 -> [w3366 w3367]
                  tunnel: [w3365 w3367] -> w3176
                  frame False {
                    n1809 = Create Folder(path (use dialog)=w3366) -> (created path=w3365:path)  [unwired: 2 in, 2 out]
                  }
                  frame True {
                  }
                }
                n1810 = call <userlib>:"OA_Load.vi"("error in (no error)"=w3190, "Path"=w3189, "Origin.IOApplication"=w3191) -> ("error out"=w3187:errorcluster, "Origin.IOApplication"=w3188:refnum<k7>)  [unwired: 1 out]
                n1811 = call <userlib>:"OAExecute.vi"("script"="document -m 3;", "Error IO"=w3187, "Origin.IOApplication"=w3188) -> ("Error IO Out"=w3185:errorcluster, "Origin.IOApplication"=w3186:refnum<k7>)  [unwired: 1 in, 1 out]
                n1812 = call "File Dialog"("start path"=w3178) -> ("selected path"=w3180:path)  [unwired: 11 in, 3 out]
                n1813 = local read "Independant Variable"() -> (w3173:string)
                n1814 = stacked-sequence {
                  tunnel: w3177 -> [w3204 w3234 w3246 w3268 w3288 w3309 w3330 w3353]
                  tunnel: w3176 -> [w3205 w3233 w3247 w3267 w3289 w3310 w3331 w3354]
                  tunnel: w3186 -> [w3207 w3231 w3249 w3270 w3291 w3312 w3333 w3356]
                  tunnel: w3185 -> [w3206 w3232 w3248 w3269 w3290 w3311 w3332 w3355]
                  tunnel: [_ _ _ _ _ _ _ w3351] -> w3175
                  tunnel: [_ _ _ _ _ _ _ w3352] -> w3174
                  tunnel: w3173 -> [w3203 w3224 w3245 w3266 w3287 w3308 w3329 w3350]
                  frame #0 {
                    n1815 = local read "X Axis Display Type"() -> (w3195:string)
                    n1816 = local read "Opj X Axis"() -> (w3200:string)
                    n1817 = Concatenate Strings("window -a MOBLGraph;\nlayer.x.type=", w3200, "; layer.x.label.numFormat = ", w3195, "; Y3 = 1; X3 = 1;", "window -a MOBLTable;\nwindow -s TV;") -> (w3198:string)
                    n1818 = call "Param_Analysis_7_24b_JW.vi"("Independant Variable"=w3203, "error in (no error)"=w3206, "Data Folder"=w3204, "Parameter String"="Mobility-Lin (cm^2/Vs):", "Parameter Name"="Mobility-Lin", "Stats Folder"=w3205) -> ("error out"=w3209:errorcluster, "Output Array"=w3211:string[][], "Variables"=w3202:T18)  [unwired: 2 in, 1 out]
                    n1819 = call "Origin_Export_7_27a_JW.vi"("Input Conditions"=w3202, "Analysis Array"=w3211, "error in (no error)"=w3209, "Parameter Worksheet Name"="[MOBLTable]Mobilities", "Parameter Folder Script"="pe_cd \"Mobility-Lin\";", "Origin.IOApplication"=w3207) -> ("error out"=w3208:errorcluster, "reference out"=w3210:refnum<k7>)  [unwired: 3 in, 1 out]
                    n1820 = call <userlib>:"OAExecute.vi"("script"=w3198, "Error IO"=w3208, "Origin.IOApplication"=w3210) -> ()  [unwired: 1 in, 3 out]
                  }
                  frame #1 {
                    n1821 = local read "X Axis Display Type"() -> (w3216:string)
                    n1822 = local read "Opj X Axis"() -> (w3221:string)
                    n1823 = Concatenate Strings("window -a MOBSGraph;\nlayer.x.type=", w3221, "; layer.x.label.numFormat = ", w3216, "; Y3 = 1; X3 = 1;", "window -a MOBSTable;\nwindow -s TV;") -> (w3219:string)
                    n1824 = call "Param_Analysis_7_24b_JW.vi"("Independant Variable"=w3224, "error in (no error)"=w3232, "Data Folder"=w3234, "Parameter String"="Mobility-Sat (cm^2/Vs):", "Parameter Name"="Mobility-Sat", "Stats Folder"=w3233) -> ("error out"=w3227:errorcluster, "Output Array"=w3225:string[][], "Variables"=w3223:T18)  [unwired: 2 in, 1 out]
                    n1825 = call "Origin_Export_7_27a_JW.vi"("Input Conditions"=w3223, "Analysis Array"=w3225, "error in (no error)"=w3227, "Parameter Worksheet Name"="[MOBSTable]Mobilities", "Parameter Folder Script"="pe_cd \"Mobility-Sat\";", "Origin.IOApplication"=w3231) -> ("error out"=w3226:errorcluster, "reference out"=w3228:refnum<k7>)  [unwired: 3 in, 1 out]
                    n1826 = call <userlib>:"OAExecute.vi"("script"=w3219, "Error IO"=w3226, "Origin.IOApplication"=w3228) -> ()  [unwired: 1 in, 3 out]
                  }
                  frame #2 {
                    n1827 = local read "X Axis Display Type"() -> (w3237:string)
                    n1828 = local read "Opj X Axis"() -> (w3242:string)
                    n1829 = Concatenate Strings("window -a NSTSGraph;\nlayer.x.type=", w3242, "; layer.x.label.numFormat = ", w3237, "; Y3 = 1; X3 = 1;", "window -a NSTSTable;\nwindow -s TV;") -> (w3240:string)
                    n1830 = call "Param_Analysis_7_24b_JW.vi"("Independant Variable"=w3245, "error in (no error)"=w3248, "Data Folder"=w3246, "Parameter String"="Trap Density-STS (Traps/Vcm^2):", "Parameter Name"="Trap Density-STS", "Stats Folder"=w3247) -> ("error out"=w3252:errorcluster, "Output Array"=w3250:string[][], "Variables"=w3244:T18)  [unwired: 2 in, 1 out]
                    n1831 = call "Origin_Export_7_27a_JW.vi"("Input Conditions"=w3244, "Analysis Array"=w3250, "error in (no error)"=w3252, "Parameter Worksheet Name"="[NSTSTable]Trap Densities", "Parameter Folder Script"="pe_cd \"N-STS\";", "Origin.IOApplication"=w3249) -> ("error out"=w3251:errorcluster, "reference out"=w3253:refnum<k7>)  [unwired: 3 in, 1 out]
                    n1832 = call <userlib>:"OAExecute.vi"("script"=w3240, "Error IO"=w3251, "Origin.IOApplication"=w3253) -> ()  [unwired: 1 in, 3 out]
                  }
                  frame #3 {
                    n1833 = local read "X Axis Display Type"() -> (w3258:string)
                    n1834 = local read "Opj X Axis"() -> (w3263:string)
                    n1835 = call "Param_Analysis_7_24b_JW.vi"("Independant Variable"=w3266, "error in (no error)"=w3269, "Data Folder"=w3268, "Parameter String"="Trap Density-VT (Traps/Vcm^2):", "Parameter Name"="Trap Density-Vt", "Stats Folder"=w3267) -> ("error out"=w3273:errorcluster, "Output Array"=w3271:string[][], "Variables"=w3265:T18)  [unwired: 2 in, 1 out]
                    n1836 = Concatenate Strings("window -a NVtGraph;\nlayer.x.type=", w3263, "; layer.x.label.numFormat = ", w3258, "; Y3 = 1; X3 = 1;", "window -a NVtTable;\nwindow -s TV;") -> (w3261:string)
                    n1837 = call "Origin_Export_7_27a_JW.vi"("Input Conditions"=w3265, "Analysis Array"=w3271, "error in (no error)"=w3273, "Parameter Worksheet Name"="[NVTTable]Trap Densities", "Parameter Folder Script"="pe_cd \"N-Vt\";", "Origin.IOApplication"=w3270) -> ("error out"=w3272:errorcluster, "reference out"=w3274:refnum<k7>)  [unwired: 3 in, 1 out]
                    n1838 = call <userlib>:"OAExecute.vi"("script"=w3261, "Error IO"=w3272, "Origin.IOApplication"=w3274) -> ()  [unwired: 1 in, 3 out]
                  }
                  frame #4 {
                    n1839 = local read "X Axis Display Type"() -> (w3279:string)
                    n1840 = local read "Opj X Axis"() -> (w3284:string)
                    n1841 = Concatenate Strings("window -a OffIGraph;\nlayer.x.type=", w3284, "; layer.x.label.numFormat = ", w3279, "; Y3 = 1; X3 = 1;", "window -a OffITable;\nwindow -s TV;") -> (w3282:string)
                    n1842 = call "Param_Analysis_7_24b_JW.vi"("Independant Variable"=w3287, "error in (no error)"=w3290, "Data Folder"=w3288, "Parameter String"="Off I-Sat (A):", "Parameter Name"="Off I-Sat", "Stats Folder"=w3289) -> ("error out"=w3294:errorcluster, "Output Array"=w3292:string[][], "Variables"=w3286:T18)  [unwired: 2 in, 1 out]
                    n1843 = call "Origin_Export_7_27a_JW.vi"("Input Conditions"=w3286, "Analysis Array"=w3292, "error in (no error)"=w3294, "Parameter Worksheet Name"="[OffItable]OffCurrents", "Parameter Folder Script"="pe_cd \"OffI-Sat\";", "Origin.IOApplication"=w3291) -> ("error out"=w3293:errorcluster, "reference out"=w3295:refnum<k7>)  [unwired: 3 in, 1 out]
                    n1844 = call <userlib>:"OAExecute.vi"("script"=w3282, "Error IO"=w3293, "Origin.IOApplication"=w3295) -> ()  [unwired: 1 in, 3 out]
                  }
                  frame #5 {
                    n1845 = local read "X Axis Display Type"() -> (w3300:string)
                    n1846 = local read "Opj X Axis"() -> (w3305:string)
                    n1847 = Concatenate Strings("window -a OnOffGraph;\nlayer.x.type=", w3305, "; layer.x.label.numFormat = ", w3300, "; Y3 = 1; X3 = 1;", "window -a OnOffTable;\nwindow -s TV;") -> (w3303:string)
                    n1848 = call "Param_Analysis_7_24b_JW.vi"("Independant Variable"=w3308, "error in (no error)"=w3311, "Data Folder"=w3309, "Parameter String"="On/Off I-Sat:", "Parameter Name"="OnOff Ratio", "Stats Folder"=w3310) -> ("error out"=w3315:errorcluster, "Output Array"=w3313:string[][], "Variables"=w3307:T18)  [unwired: 2 in, 1 out]
                    n1849 = call "Origin_Export_7_27a_JW.vi"("Input Conditions"=w3307, "Analysis Array"=w3313, "error in (no error)"=w3315, "Parameter Worksheet Name"="[OnOffTable]On/Off Ratios", "Parameter Folder Script"="pe_cd \"OnOff-Ratio\";", "Origin.IOApplication"=w3312) -> ("error out"=w3314:errorcluster, "reference out"=w3316:refnum<k7>)  [unwired: 3 in, 1 out]
                    n1850 = call <userlib>:"OAExecute.vi"("script"=w3303, "Error IO"=w3314, "Origin.IOApplication"=w3316) -> ()  [unwired: 1 in, 3 out]
                  }
                  frame #6 {
                    n1851 = local read "X Axis Display Type"() -> (w3321:string)
                    n1852 = local read "Opj X Axis"() -> (w3326:string)
                    n1853 = call "Param_Analysis_7_24b_JW.vi"("Independant Variable"=w3329, "error in (no error)"=w3332, "Data Folder"=w3330, "Parameter String"="STS-Sat (V/decade):", "Parameter Name"="STS-Sat", "Stats Folder"=w3331) -> ("error out"=w3336:errorcluster, "Output Array"=w3334:string[][], "Variables"=w3328:T18)  [unwired: 2 in, 1 out]
                    n1854 = Concatenate Strings("window -a SGraph;\nlayer.x.type=", w3326, "; layer.x.label.numFormat = ", w3321, "; Y3 = 1; X3 = 1;", "window -a STable;\nwindow -s TV;") -> (w3324:string)
                    n1855 = call "Origin_Export_7_27a_JW.vi"("Input Conditions"=w3328, "Analysis Array"=w3334, "error in (no error)"=w3336, "Parameter Worksheet Name"="[STable]Threshold Swing", "Parameter Folder Script"="pe_cd \"STS-Sat\";", "Origin.IOApplication"=w3333) -> ("error out"=w3335:errorcluster, "reference out"=w3337:refnum<k7>)  [unwired: 3 in, 1 out]
                    n1856 = call <userlib>:"OAExecute.vi"("script"=w3324, "Error IO"=w3335, "Origin.IOApplication"=w3337) -> ()  [unwired: 1 in, 3 out]
                  }
                  frame #7 {
                    n1857 = local read "X Axis Display Type"() -> (w3342:string)
                    n1858 = local read "Opj X Axis"() -> (w3347:string)
                    n1859 = Concatenate Strings("window -a VtGraph;\nlayer.x.type=", w3347, "; layer.x.label.numFormat = ", w3342, "; Y3 = 1; X3 = 1;", "window -a VtTable;\nwindow -s TV;") -> (w3345:string)
                    n1860 = call "Param_Analysis_7_24b_JW.vi"("Independant Variable"=w3350, "error in (no error)"=w3355, "Data Folder"=w3353, "Parameter String"="Vt-Sat (V):", "Parameter Name"="Vt-Sat", "Stats Folder"=w3354) -> ("error out"=w3359:errorcluster, "Output Array"=w3357:string[][], "Variables"=w3349:T18)  [unwired: 2 in, 1 out]
                    n1861 = call "Origin_Export_7_27a_JW.vi"("Input Conditions"=w3349, "Analysis Array"=w3357, "error in (no error)"=w3359, "Parameter Worksheet Name"="[VtTable]Threshold Voltages", "Parameter Folder Script"="pe_cd \"Vt-Sat\";", "Origin.IOApplication"=w3356) -> ("error out"=w3358:errorcluster, "reference out"=w3360:refnum<k7>)  [unwired: 3 in, 1 out]
                    n1862 = call <userlib>:"OAExecute.vi"("script"=w3345, "Error IO"=w3358, "Origin.IOApplication"=w3360) -> ("Error IO Out"=w3351:errorcluster, "Origin.IOApplication"=w3352:refnum<k7>)  [unwired: 1 in, 1 out]
                  }
                }
                n1863 = Path To String(path=w3180) -> (string=w3179:string)
                n1864 = call <userlib>:"OAExecute.vi"("script"="pe_cd /; ", "Error IO"=w3175, "Origin.IOApplication"=w3174) -> ("Error IO Out"=w3181:errorcluster, "Origin.IOApplication"=w3182:refnum<k7>)  [unwired: 1 in, 1 out]
                n1865 = call <userlib>:"OASaveProject.vi"("path"=w3179, "Error IO"=w3181, "Origin.IOApplication"=w3182) -> ()  [unwired: 3 out]
              }
            }
          }
          event "Blank Button": Mouse Down {
            n1866 = event-data() -> ()  [unwired: 1 in, 7 out]
            n1867 = local read "Transfer File"() -> (w3375:path)
            n1868 = disable-structure shown="Disabled" {
              frame Disabled {
                n1869 = local read "Folder Index"() -> (w3376:dbl)
                n1870 = Decrement(x=w3376) -> (x-1=w3377:dbl)
                n1871 = local write "Folder Index"(w3377) -> ()
              }
              frame Enabled {
              }
            }
            n1872 = Strip Path(path=w3375) -> (stripped path=w3371:path, name=w3373:string)
            n1873 = Path To String(path=w3371) -> (string=w3370:string)
            n1874 = Concatenate Strings(w3370, "\\", "X_", w3373) -> (w3369:string)
            n1875 = String To Path(string=w3369) -> (path=w3368:path)
            n1876 = Move(source path=w3375, 10:w3368) -> ()  [unwired: 3 in, 3 out]
            n1877 = local write "Transfer File"(w3368) -> ()
          }
          event "Cancel Button": Mouse Down {
            (unwired) 6
            n1878 = event-data() -> ()  [unwired: 1 in, 7 out]
            n1879 = call "Simulate_Keyboard.vi"("Action"=2, "Virtual Key"=162) -> ()  [unwired: 7 in, 1 out]
          }
        }
        n1880 = Multiply(x=w459, y=10) -> (x*y=w461:sgl)
        n1881 = case shown="\"0\"" w500 {
          tunnel: w474 -> [w639 w645 w649 w651 w655 w657 w659 w661 w663 w665 w667 w669 w671 w673 w675 w677 w679 w681 w683 w685 w687 w689 w691 w693 w695 w697 w699 w701 w703 w705 w707 w709 w711 w713 w715 w717 w719 w721 w723 w725 w727 w729 w731 w733 w735 w737 w739 w741 w743 w745 w747 w749 w751 w753 w755 w757 w759 w761 w763 w765 w767 w769 w771 w773 w775 w777 w779 w781 w783 w785 w787 w789 w791 w793 w795 w797 w799 w801 w803 w805 w807 w809 w811 w813 w815 w817 w819 w821 w823 w825 w827 w829 w831 w833 w835 w837 w839 w841 w843 w845 w847 w849 w851 w853 w855]
          tunnel: [w639 w644 w648 w651 w655 w657 w659 w661 w663 w665 w667 w669 w671 w673 w675 w677 w679 w681 w683 w685 w687 w689 w691 w693 w695 w697 w699 w701 w703 w705 w707 w709 w711 w713 w715 w717 w719 w721 w723 w725 w727 w729 w731 w733 w735 w737 w739 w741 w743 w745 w747 w749 w751 w753 w755 w757 w759 w761 w763 w765 w767 w769 w771 w773 w775 w777 w779 w781 w783 w785 w787 w789 w791 w793 w795 w797 w799 w801 w803 w805 w807 w809 w811 w813 w815 w817 w819 w821 w823 w825 w827 w829 w831 w833 w835 w837 w839 w841 w843 w845 w847 w849 w851 w853 w855] -> w499
          tunnel: w475 -> [w641 w643 w647 w653 w654 w656 w658 w660 w662 w664 w666 w668 w670 w672 w674 w676 w678 w680 w682 w684 w686 w688 w690 w692 w694 w696 w698 w700 w702 w704 w706 w708 w710 w712 w714 w716 w718 w720 w722 w724 w726 w728 w730 w732 w734 w736 w738 w740 w742 w744 w746 w748 w750 w752 w754 w756 w758 w760 w762 w764 w766 w768 w770 w772 w774 w776 w778 w780 w782 w784 w786 w788 w790 w792 w794 w796 w798 w800 w802 w804 w806 w808 w810 w812 w814 w816 w818 w820 w822 w824 w826 w828 w830 w832 w834 w836 w838 w840 w842 w844 w846 w848 w850 w852 w854]
          tunnel: [w640 w643 w647 w652 w654 w656 w658 w660 w662 w664 w666 w668 w670 w672 w674 w676 w678 w680 w682 w684 w686 w688 w690 w692 w694 w696 w698 w700 w702 w704 w706 w708 w710 w712 w714 w716 w718 w720 w722 w724 w726 w728 w730 w732 w734 w736 w738 w740 w742 w744 w746 w748 w750 w752 w754 w756 w758 w760 w762 w764 w766 w768 w770 w772 w774 w776 w778 w780 w782 w784 w786 w788 w790 w792 w794 w796 w798 w800 w802 w804 w806 w808 w810 w812 w814 w816 w818 w820 w822 w824 w826 w828 w830 w832 w834 w836 w838 w840 w842 w844 w846 w848 w850 w852 w854] -> w498
          tunnel: w461 -> [w638 w642 w646 w650 _ _ _ _ _ _ _ _ _ _ _ _ _ _ _ _ _ _ _ _ _ _ _ _ _ _ _ _ _ _ _ _ _ _ _ _ _ _ _ _ _ _ _ _ _ _ _ _ _ _ _ _ _ _ _ _ _ _ _ _ _ _ _ _ _ _ _ _ _ _ _ _ _ _ _ _ _ _ _ _ _ _ _ _ _ _ _ _ _ _ _ _ _ _ _ _ _ _ _ _ _]
          frame "DOWN" {
            n1882 = Add(x=w641, y=w638) -> (x+y=w640:sgl)
          }
          frame "LEFT" {
            n1883 = Subtract(x=w645, y=w642) -> (x-y=w644:sgl)
          }
          frame "RIGHT" {
            n1884 = Add(x=w649, y=w646) -> (x+y=w648:sgl)
          }
          frame "UP" {
            n1885 = Subtract(x=w653, y=w650) -> (x-y=w652:sgl)
          }
          frame "ENTER (num pad)" {
          }
          frame "' (quote)" {
          }
          frame "END" {
          }
          frame "EQUALS" {
          }
          frame "ESCAPE" {
          }
          frame "GRAVE (`)" {
          }
          frame "HOME" {
          }
          frame "INSERT" {
          }
          frame "LBRACKET" {
          }
          frame "LCONTROL" {
          }
          frame "L ALT" {
          }
          frame "LSHIFT" {
          }
          frame "LWIN" {
          }
          frame "MINUS" {
          }
          frame "MULTIPLY" {
          }
          frame "NEXT" {
          }
          frame "NUMLOCK" {
          }
          frame "NUMPAD_0" {
          }
          frame "NUMPAD_1" {
          }
          frame "NUMPAD_2" {
          }
          frame "NUMPAD_3" {
          }
          frame "NUMPAD_4" {
          }
          frame "NUMPAD_5" {
          }
          frame "NUMPAD_6" {
          }
          frame "NUMPAD_7" {
          }
          frame "NUMPAD_8" {
          }
          frame "NUMPAD_9" {
          }
          frame "PAUSE" {
          }
          frame "PERIOD" {
          }
          frame "PRIOR (PG UP)" {
          }
          frame "RBRACKET" {
          }
          frame "RCONTROL" {
          }
          frame "RETURN" {
          }
          frame "R ALT" {
          }
          frame "RSHIFT" {
          }
          frame "RWIN" {
          }
          frame "SCROLL" {
          }
          frame "SEMICOLON" {
          }
          frame "SLASH" {
          }
          frame "SPACE" {
          }
          frame "SUBTRACT" {
          }
          frame "TAB" {
          }
          frame "DIVIDE" {
          }
          frame "DELETE" {
          }
          frame "DECIMAL" {
          }
          frame "COMMA" {
          }
          frame "CAPITAL" {
          }
          frame "BACKSLASH" {
          }
          frame "BACK" {
          }
          frame "ADD" {
          }
          frame "F15" {
          }
          frame "F14" {
          }
          frame "F13" {
          }
          frame "F12" {
          }
          frame "F11" {
          }
          frame "F10" {
          }
          frame "F9" {
          }
          frame "F8" {
          }
          frame "F7" {
          }
          frame "F6" {
          }
          frame "F5" {
          }
          frame "F4" {
          }
          frame "F3" {
          }
          frame "F2" {
          }
          frame "F1" {
          }
          frame "Z" {
          }
          frame "Y" {
          }
          frame "X" {
          }
          frame "W" {
          }
          frame "V" {
          }
          frame "U" {
          }
          frame "T" {
          }
          frame "S" {
          }
          frame "R" {
          }
          frame "Q" {
          }
          frame "P" {
          }
          frame "O" {
          }
          frame "N" {
          }
          frame "M" {
          }
          frame "L" {
          }
          frame "K" {
          }
          frame "J" {
          }
          frame "I" {
          }
          frame "H" {
          }
          frame "G" {
          }
          frame "F" {
          }
          frame "E" {
          }
          frame "D" {
          }
          frame "C" {
          }
          frame "B" {
          }
          frame "A" {
          }
          frame "9" {
          }
          frame "8" {
          }
          frame "7" {
          }
          frame "6" {
          }
          frame "5" {
          }
          frame "4" {
          }
          frame "3" {
          }
          frame "2" {
          }
          frame "1" {
          }
          frame "0" {
          }
        }
        n1886 = Bundle(w477, w476, w491, w490, 0.0) -> (w489:cluster{dbl, dbl, dbl, dbl, dbl})  [unwired: 1 in]
        n1887 = Bundle("X"=w499, "Y"=w498) -> (w493:cluster{"X":sgl, "Y":sgl})  [unwired: 1 in]
        n1888 = Divide(x=20, y=w460) -> (x/y=w463:sgl)
        n1889 = property on="Image Out" class="ImageControl"("Image Center Position"=w493) -> ()  [unwired: 2 in, 2 out]
        n1890 = call "IMAQ Convert Rectangle to ROI (Polygon)"("Rectangle"=w489) -> ("ROI Descriptor"=w487:T4)  [unwired: 7 in, 2 out]
        n1891 = Bundle("Application Font", w463, w467, w467, w467, w467, w467, TRUE, w465) -> (w469:T19)  [unwired: 1 in]
        n1892 = property on="Image Out 2" class="ImageControl"("ROI"=w487) -> ()  [unwired: 2 in, 2 out]
        n1893 = Bundle(w465, w469, w465, w465) -> (w468:T20)  [unwired: 1 in]
        n1894 = property on="Image Out" class="ImageControl"() -> ("ROI"=w452:T12)  [unwired: 2 in, 2 out]
        n1895 = Unbundle By Name(w452) -> ("Contours"=w516:T16)
        n1896 = local read "Image Out"() -> (w471:T2)
        n1897 = call "IMAQ Clear Overlay"("Image"=w471) -> ("Image Out"=w470:T2)  [unwired: 9 in, 1 out]
        n1898 = Initialize Array(0) -> (w514:i32[])  [unwired: 1 in]
        n1899 = local read "Magnification"() -> (w505:u16)
        n1900 = Array Size(array=w516) -> (size(s)=w515:i32)
        n1901 = Build Array(0.505025, 0.252522, 0.127742, 0.050345, 0.031129) -> (w506:dbl[])
        n1902 = Array Subset(array=w506, index=w505, length=1) -> (w503:dbl[])
        n1903 = property on="Image Out" class="ImageControl"() -> ("ZoomInteger"=w495:cluster{"X":i32, "Y":i32})  [unwired: 2 in, 2 out]
        n1904 = To Double Precision Float(number=w503) -> (double precision float=w502:dbl[])
        n1905 = for {
          N: w515 -> [_]
          shift-right: [w878] -> _
          shift-left: w516 -> [w878]
          shift-right: [w876] -> w501
          shift-left: w514 -> [w875]
          tunnel: w502 -> [w874]
          shift-right: [w871] -> _
          shift-left: w470 -> [w873]
          tunnel: w468 -> [w866]
          i -> [w870]
          n1906 = Index Array(array=w878, index=w870) -> (element=w887:T21)
          n1907 = Unbundle(w887) -> ("Points"=w886:i32[])  [unwired: 2 out]
          n1908 = Array To Cluster(array=w886) -> (cluster=w885:T22)
          n1909 = Unbundle(w885) -> ("Points[0]"=w865:i32, "Points[1]"=w862:i32, "Points[2]"=w877:i32, "Points[3]"=w883:i32)  [unwired: 5 out]
          n1910 = Add(x=w865, y=10) -> (x+y=w863:i32)
          n1911 = Subtract(x=w862, y=w883) -> (x-y=w882:i32)
          n1912 = Subtract(x=w865, y=w877) -> (x-y=w884:i32)
          n1913 = Square(x=w882) -> (x^2=w880:i32)
          n1914 = Square(x=w884) -> (x^2=w881:i32)
          n1915 = Add(x=w881, y=w880) -> (x+y=w879:i32)
          n1916 = Square Root(x=w879) -> (sqrt(x)=w856:dbl)
          n1917 = Multiply(x=w856, y=0.5) -> (x*y=w859:dbl)
          n1918 = Add(x=w859, y=w862) -> (x+y=w861:dbl)
          n1919 = Bundle(w863, w861) -> (w872:cluster{i32, dbl})  [unwired: 1 in]
          n1920 = Multiply(x=w856, y=w874) -> (x*y=w869:dbl[])
          n1921 = Index Array(array=w869) -> (element=w868:dbl)  [unwired: 1 in]
          n1922 = Number To Fractional String(number=w868) -> (F-format string=w867:string)  [unwired: 3 in]
          n1923 = call "IMAQ Overlay Text"("BG Color (Transparent)"=u32 0, "Text Color (black)"=u32 16448250, "Font, Size & Style"=w866, "String"=w867, "Origin"=w872, "Image"=w873) -> ("Image Out"=w871:T2)  [unwired: 4 in, 1 out]
          n1924 = Build Array (concatenate)(w875, w869) -> (w876:dbl[])
          n1925 = local write "Numeric 3"(w856) -> ()
        }
        n1926 = local write "ROI Descriptor"(w452) -> ()
        n1927 = Unbundle(w495) -> ("X"=w494:i32)  [unwired: 1 out]
        n1928 = Add Array Elements(numeric array=w501) -> (sum=w512:dbl)
        n1929 = local write "Distances"(w501) -> ()
        n1930 = local write "Total Width"(w512) -> ()
        n1931 = local write "Zoom"(w494) -> ()
        n1932 = local read "Manual-Width"() -> (w418:bool)
        n1933 = local read "Total Width"() -> (w455:dbl)
        n1934 = local read "Rec: Width"() -> (w453:dbl)
        n1935 = case shown="False" w418 {
          frame False {
            n1936 = property on="New: Width" class="DigNum (strict)"("DisabledEnum"=1) -> ()  [unwired: 2 in, 2 out]
          }
          frame True {
            n1937 = property on="New: Width" class="DigNum (strict)"("DisabledEnum"=0) -> ()  [unwired: 2 in, 2 out]
          }
        }
        n1938 = Not(x=w418) -> (.not. x?=w450:bool)
        n1939 = Equal To 0?(x=w455) -> (x = 0?=w451:bool)
        n1940 = Or(x=w451, y=w418) -> (x .or. y?=w454:bool)
        n1941 = And(x=w451, y=w450) -> (x .and. y?=w449:bool)
        n1942 = case shown="True" w449 {
          tunnel: w453 -> [_ w614]
          frame False {
          }
          frame True {
            n1943 = local write "New: Width"(w614) -> ()
          }
        }
        n1944 = case shown="False" w454 {
          tunnel: w455 -> [w616 _]
          frame False {
            n1945 = local write "New: Width"(w616) -> ()
            n1946 = property on="New: Width" class="DigNum (strict)"("DisabledEnum"=1) -> ()  [unwired: 2 in, 2 out]
          }
          frame True {
            n1947 = property on="New: Width" class="DigNum (strict)"("DisabledEnum"=0) -> ()  [unwired: 2 in, 2 out]
          }
        }
        n1948 = local read "Manual Comments"() -> (w419:bool)
        n1949 = local read "Rec: Comments"() -> (w420:string)
        n1950 = local read "Manuel-Dielectric"() -> (w446:bool)
        n1951 = local read "Rec: Dielectric (d)"() -> (w445:dbl)
        n1952 = local read "Manuel-Length"() -> (w447:bool)
        n1953 = local read "Rec: Length"() -> (w448:dbl)
        n1954 = case shown="True" w419 {
          tunnel: w420 -> [w597 _]
          frame False {
            n1955 = local write "Comments:"(w597) -> ()
            n1956 = property on="Comments:" class="Str"("DisabledEnum"=1) -> ()  [unwired: 2 in, 2 out]
          }
          frame True {
            n1957 = property on="Comments:" class="Str"("DisabledEnum"=0) -> ()  [unwired: 2 in, 2 out]
          }
        }
        n1958 = case shown="True" w447 {
          tunnel: w448 -> [w612 _]
          frame False {
            n1959 = local write "New: Length"(w612) -> ()
            n1960 = property on="New: Length" class="DigNum (strict)"("DisabledEnum"=1) -> ()  [unwired: 2 in, 2 out]
          }
          frame True {
            n1961 = property on="New: Length" class="DigNum (strict)"("DisabledEnum"=0) -> ()  [unwired: 2 in, 2 out]
          }
        }
        n1962 = case shown="True" w446 {
          tunnel: w445 -> [w609 _]
          frame False {
            n1963 = local write "New: Dielectric"(w609) -> ()
            n1964 = property on="New: Dielectric" class="DigNum (strict)"("DisabledEnum"=1) -> ()  [unwired: 2 in, 2 out]
          }
          frame True {
            n1965 = property on="New: Dielectric" class="DigNum (strict)"("DisabledEnum"=0) -> ()  [unwired: 2 in, 2 out]
          }
        }
      }
    }
  }
  n1966 = disable-structure shown="Disabled" {
    frame Disabled {
      # "Transformer Work"
      n1967 = Build Array("DeviceID", "Fabricator", "Deposition", "Date", "Sample", "Row", "Column", "L (um)", "W (um)", "Material", "Treatment", "TC (mM)", "Solvent", "C (%)", "ST (C)", "Drops", "Wait (s)", "RT (F)", "RH (%)", "Ramp (s)", "RPM", "Accel (RPM/s)", "Time (s)", "Mobility", "On/Off", "Vt", "S.T.S") -> (→"Transformer \nHeaders":string[])
    }
    frame Enabled {
    }
  }
